vi "test exe main.vi"(6 "Offset":dbl=5.0, 7 "CustormMode":bool, 8 "error in":errorcluster, 10 "HWcurrent limt":sgl=0.5, 11 "Main State Cluster":T1={"Application Status"="", "Switch Output Array"=[], "Switch Value Configuration"=[], "NVH Configuration"={"NVH Station?"=FALSE, "nvh app instance path"="", "NVH_ErrorMessages sv url"="", "NVH_Inputs sv url"="", "NVH_MotionNumber sv url"="", "NVH_Outputs sv url"="", "NVH_PartNumber sv url"="", "NVH_PartNumber_Echo sv url"="", "NVH_SerialNumber sv url"="", "NVH_AmbientTempF sv url"=""}, "rs232 port map"={"PMAC"="COM3", "PS Port"="COM27", "LVDT Unit"="COM36", "RS232"="COM24"}, "ethernet address map"={"LVDT 1 Unit"="172.17.53.143", "LVDT Unit 1 port"=0}, "paths"={"Base Path"=path "", "system error log path"=path "", "Error Table Path"=path "C/Labview Code/System/Error Table", "Store errors log path"=path "C/Labview Code/System/Error Table", "data bytes log path"=path "C/Labview Code/System/Error Table", "network path"=path "C/Labview Code/System/Error Table"}, "Station Index"=0, "Store Data"={"Motion Data Array"=[], "Error Table"=[], "Sun Shade Close Force Limits"={"Overall Min"=0.0, "Overall Max"=0.0, "Avg Min"=0.0, "Avg Max"=0.0, "Truncation Start"=0.0, "Truncation End"=0.0, "Variance"=0.0, "Check Noise"=FALSE}, "Sun Shade Open Force Limits"={"Overall Min"=0.0, "Overall Max"=0.0, "Avg Min"=0.0, "Avg Max"=0.0, "Truncation Start"=0.0, "Truncation End"=0.0, "Variance"=0.0, "Check Noise"=FALSE}, "Sunshade Open Data"=[], "Sunshade Close Data"=[], "Module Info"={"Serial Number"="", "Pallet Number"="", "Sunshade Color"="", "Inalfa Part Number"="", "Customer Number"=""}, "Sunsahde Close Raw Data"=[], "Sunshade Open Raw Data"=[], "Software Version"=[], "Constant Version"=[], "Hardware Version"=[], "Inalfa Part Number ECU"=[], "LVDT Data"=[], "Communication Line 1"=[], "Communication Line 2"=[], "Anti Pinch Force"=[], "Cycle Time"="", "Anti Pinch Vent Force"=[], "iGPS LVDT Data"=[], "data bytes log"=""}, "D in map"={"Abort Test"=enum."Dev2/port2/line6", "Start Test"=enum."Dev2/port2/line6"}, "DO Task"="station 1 dio", "ctl refs"={"Start Test"=refnum, "Abort Test"=refnum, "Manual Control"=refnum, "Route to Repair"=refnum, "Waveform Graph"=refnum, "Motion Data"=refnum, "all station status"=refnum, "Individual Station Status"=refnum, "exit program"=refnum, "Sunshade Servo Data Open"=refnum, "Sunshade Servo Data Close"=refnum, "Red-Rabbit Mode"=refnum, "Direct Manual Ctrl"=refnum}, "misc station config"={"Station Name"="", "is AT station?"=FALSE, "is audit station?"=FALSE, "power supply type"=enum."GENser", "use alt China TP2 LVDT Logic Seq"=FALSE, "hmi operator abort timeout"=0, "dump all analog values even if pass"=FALSE, "debug log pre-filter ap stream bytes"=FALSE, "use separate lvdt x and z extend tags"=FALSE, "is print"=FALSE}, "ethernet tcp refs"={"LVDT Unit"=refnum}, "Sunshade Barcode Scan"={"Sunshade Number 2"="", "Sunshade Number 1"="", "Keyence tuning bank idx"=0}, "AP Test Data"={"Raw Sunshade AP Data"="", "Raw Glass AP Data"="", "PMAC Read Counter"=0.0, "Database AP Data"=[]}, "Motion Status"={"hmi operator abort start time"=0, "Current Data Index"=0, "Analog Data"=[], "Motor Position Hex"=0, "Messages Index"=0, "Last Bytes"=[], "Current Hall Position"=0, "Motion Stop Timer"=0, "Position Test"=enum."Not Tested", "Noise Test"=enum."Not Tested", "motion stop check initialized"=FALSE, "remote sense enabled"=FALSE, "Motion"=enum."Glass Teach"}, "LVDT Status"={"LVDT's stored config"=[], "lvdt precision"={"truncate instead of rounding"=FALSE, "decimal places"=0}}, "Sequence State"={"Step Description"="", "Cycle Start Time"=0, "Step Data String"="", "Pass?"=FALSE, "Seqence"=[], "Active Step"=0, "Testing?"=FALSE, "Red-Rabbit Mode"=FALSE, "route-to-repair mode"=FALSE, "NVH Status"={"Restart IRQ Counter"=0, "NVH Test Needed?"=FALSE, "NVH Test Running?"=FALSE}, "Present (s)"=0.0, "Hold Mode?"=FALSE, "Hold?"=FALSE, "Rx Invalid?"=FALSE}, "misc status"={"delay start time (ticks)"=0, "In Vehicle Mode?"=FALSE, "Diag Mode?"=FALSE, "Serial Port Configured?"=FALSE, "PS Voltage"=0.0, "Diag Serial Port"="", "Part Setup"={"Communication Type"=enum."None", "Send Messages to"=enum."Glass", "RAP Signal"=enum."High", "Motor Type"=enum."Smart Motor", "NVH Part Number"=0, "Turn Off Timer"=0, "Part Type"=""}, "Part History Number"="", "Plant Number"=0, "AP Data Type"=enum."91/61", "Real Rollo?"=FALSE}, "NVH Operator?"=FALSE, "NVH Pass?"=FALSE, "Operator Pass?"=FALSE, "Operator Action?"=FALSE, "Noise Source"=0, "USBHandle"=0, "PeakInfo"="", "PeakNumber"=0, "NVH Motion Steps"=[], "Second Check?"=FALSE, "Decibel data"=[], "Direct Control Info"={"EnableStopOnHome"=FALSE, "EnableStopOnPos"=FALSE, "TeachEvent"=FALSE, "open offset"=0, "close offset"=0, "Derect control"=FALSE, "set position"=[], "teach pass "=FALSE, "Drift offsets"=[], "Hall Positions"=[]}, "manual control(direct)"=FALSE, "LIN INFO"={"Toolkit Type"=enum."Inalfa LIN", "NAD"=36, "Inalfa LIN"={"Master Frame(3C)"="", "Slave Frame(3D)"="NIXNET_exampleLDF", "Request Schedule"="NIXNET_exampleLDF", "Response Schedule"="CEMLIN3DiagResponseSchedule\nSPA3414_ConfigurationsCMAGeely_CEMCALYPSOSDB34XX0Cfg_LIN3_190709_", "Frame Write SCU"="", "Frame Read SCU"="", "LIN Name"=""}, "ADCS LIN"={"Port"="MasterReq\nSPA3414_ConfigurationsCMAGeely_CEMCALYPSOSDB34XX0Cfg_LIN3_190709_", "HW select"=0, "XNET Cluster"="SlaveResp\nSPA3414_ConfigurationsCMAGeely_CEMCALYPSOSDB34XX0Cfg_LIN3_190709_", "ByteCmd Path"=path "C/Labview Code/System/ByteCmdConfig.txt"}, "TS LIN"={"ref info"=refnum, "LIN Channel"=0, "ByteCmd Path"=path "C/Labview Code/System/ByteCmdConfig.txt"}}, "Config Info"=variant} {"LIN INFO"."NAD" format="%.0x"; "LIN INFO"."ADCS LIN"."HW select" items=["NI-XNET", "NI-CAN"]; "LVDT Status"."LVDT's stored config"."Lower Limit" format="%.2f"; "LVDT Status"."LVDT's stored config"."Upper Limit" format="%.2f"; "Store Data"."Sun Shade Open Force Limits"."Variance" format="%.2g"; "Store Data"."Sun Shade Open Force Limits"."Truncation End" format="%.2g"; "Store Data"."Sun Shade Open Force Limits"."Truncation Start" format="%.2g"; "Store Data"."Sun Shade Open Force Limits"."Avg Max" format="%.2g"; "Store Data"."Sun Shade Open Force Limits"."Avg Min" format="%.2g"; "Store Data"."Sun Shade Open Force Limits"."Overall Max" format="%.2g"; "Store Data"."Sun Shade Open Force Limits"."Overall Min" format="%.2g"; "Store Data"."Sun Shade Close Force Limits"."Variance" format="%.2g"; "Store Data"."Sun Shade Close Force Limits"."Truncation End" format="%.2g"; "Store Data"."Sun Shade Close Force Limits"."Truncation Start" format="%.2g"; "Store Data"."Sun Shade Close Force Limits"."Avg Max" format="%.2g"; "Store Data"."Sun Shade Close Force Limits"."Avg Min" format="%.2g"; "Store Data"."Sun Shade Close Force Limits"."Overall Max" format="%.2g"; "Store Data"."Sun Shade Close Force Limits"."Overall Min" format="%.2g"; "Store Data"."Motion Data Array"."Motion Data Limits"."LIN Msg"."Msg" format="%02x"; "Store Data"."Motion Data Array"."Motion Data Limits"."LIN Msg"."ID" format="%02x"}) -> (0 "error out":errorcluster)   [LabVIEW 2018]
uses:
  02.Type Def's/main state cluster.ctl
  02.Type Def's/All Switch Configuration Cluster.ctl
  02.Type Def's/All Motions.ctl
  02.Type Def's/EOL Switch Value Configuration Cluster.ctl
  02.Type Def's/EOL Switch Max Min Check Cluster.ctl
  02.Type Def's/station nvh config.ctl
  02.Type Def's/station rs232 port map.ctl
  02.Type Def's/station ethernet address map.ctl
  02.Type Def's/station paths.ctl
  02.Type Def's/EOL Save Module Test Data Control.ctl
  02.Type Def's/EOL Motion Database Table.ctl
  05.UserVI's/type defs/17x Audit Motion Data Seq Control.ctl
  05.UserVI's/type defs/17x AP Data Type.ctl
  05.UserVI's/type defs/17x Sunshade Limts Seq.ctl
  02.Type Def's/EOL Module Info Control.ctl
  02.Type Def's/station DI map.ctl
  05.UserVI's/type defs/EOL Global Digital Input Control.ctl
  02.Type Def's/control refs.ctl
  02.Type Def's/station motion data indicator.ctl
  02.Type Def's/Screen Motion Data.ctl
  02.Type Def's/Pass Fail Control.ctl
  02.Type Def's/station hmi.ctl
  02.Type Def's/lvdt name val pair.ctl
  02.Type Def's/individual station status.ctl
  02.Type Def's/misc station config.ctl
  05.UserVI's/Lambda Power/power supply types.ctl
  05.UserVI's/type defs/EOL LVDT's Check Controller.ctl
  05.UserVI's/LVDT's/lvdt precision.ctl
  02.Type Def's/sequence state.ctl
  05.UserVI's/sequence/type defs/Sequence Info.ctl
  05.UserVI's/type defs/EOL Part Setup.ctl
  02.Type Def's/All Communication Types.ctl
  05.UserVI's/type defs/Communication with Motors.ctl
  05.UserVI's/type defs/RAP Signal Control.ctl
  05.UserVI's/type defs/EOL Motor Type.ctl
  02.Type Def's/station LIN config.ctl
  03.Inalfa LIN/LIN Device.ctl
  <vilib>/CMC.AME/Inalfa ADCS/Ctl'Def/ADCS_LIN info.ctl
  C:/Program Files (x86)/National Instruments/LabVIEW 2018/vi.lib/CMC.AME/Inalfa TS LIN/TOSUN/TSMaster/bin/Interop.TSMasterAPI.dll
  Program Files (x86)/National Instruments/LabVIEW 2018/vi.lib/CMC.AME/Inalfa TS LIN/TOSUN/TSMaster/bin/Interop.TSMasterAPI.dll
  Sub'VIs/Type Def's/Config Info.ctl
  02.Type Def's/NVH Mode Control 2.0.ctl
  02.Type Def's/NVH Digital Input.ctl
  02.Type Def's/EOL Analog Input Control.ctl
  02.Type Def's/failure behaviors.ctl
  05.UserVI's/type defs/RSLinx Boolean Cluster.ctl
  05.UserVI's/type defs/plc path and tag.ctl
  <vilib>/Platform/dataskt.llb/DataSocket Reference Type.ctl
  05.UserVI's/type defs/sequence goto step params.ctl
  05.UserVI's/type defs/EOL Global Digital Output Cluster Control.ctl
  05.UserVI's/type defs/EOL Global Digital Output Control.ctl
  05.UserVI's/BarCode/typedefs/barcode format params.ctl
  05.UserVI's/BarCode/typedefs/barcode printer types.ctl
  02.Type Def's/Sunshade Color Configuration Cluster.ctl
  05.UserVI's/type defs/Anti Pinch Test Data Control.ctl
  05.UserVI's/type defs/Goto Position Control.ctl
  02.Type Def's/NVH Digital Output.ctl
  <vilib>/Instr/_visa.llb/VISA Configure Serial Port (Instr).vi
  04.SubVI's/Fergus/ZUP_Current/Data buffer/ST0 current buffer.vi
  04.SubVI's/Fergus/ZUP_Current/Data buffer/ST1 current buffer.vi
  04.SubVI's/Fergus/ZUP_Current/Data buffer/ST2 current buffer.vi
  04.SubVI's/Fergus/ZUP_Current/Data buffer/ST3 current buffer.vi
  04.SubVI's/Fergus/ZUP_Current/Data buffer/ST4 current buffer.vi
  04.SubVI's/Fergus/ZUP_Current/Data buffer/ST5 current buffer.vi
  04.SubVI's/Others VI's/ftd2xx.dll
  <vilib>/Utility/config.llb/NI_LVConfig.lvlib
  <vilib>/Utility/config.llb/Read Key (String).vi
panel:
  in  "VI路径":path=path "C:/Labview Code/04.SubVI's/Direct Control Test/MotorDirectControl.vi"
  # "Sunroof Barcode"
  # "Pallet Number"
  # "Part Type"
  # "Application Status"
  # "Current Step"
  # "Cycle Time"
  # "Pass / Fail"
  # "Shade Close"
  # "Actual Data"
  # "Limits"
  # "Avg Current"
  # "Run Time"
  # "Speed"
  # "Noise Test"
  # "Position"
  # "Shade Open"
  # "Actual Data"
  # "Limits"
  # "Avg Current"
  # "Run Time"
  # "Speed"
  # "Noise Test"
  # "Position"
  # "Vent Close"
  # "Actual Data"
  # "Limits"
  # "Avg Current"
  # "Run Time"
  # "Speed"
  # "Noise Test"
  # "Position"
  # "Vent Open"
  # "Actual Data"
  # "Limits"
  # "Avg Current"
  # "Run Time"
  # "Speed"
  # "Noise Test"
  # "Position"
  # "Slide Close"
  # "Actual Data"
  # "Limits"
  # "Avg Current"
  # "Run Time"
  # "Speed"
  # "Noise Test"
  # "Position"
  # "Slide Open"
  # "Actual Data"
  # "Limits"
  # "Avg Current"
  # "Run Time"
  # "Speed"
  # "Noise Test"
  # "Position"
  # "Min"
  # "N"
  # "Min"
  # "Start"
  # "N"
  # "Max"
  # "N"
  # "Max"
  # "N"
  # "End"
  # "Min"
  # "N"
  # "Min"
  # "Start"
  # "N"
  # "Max"
  # "N"
  # "Max"
  # "N"
  # "End"
  # "Min"
  # "Max"
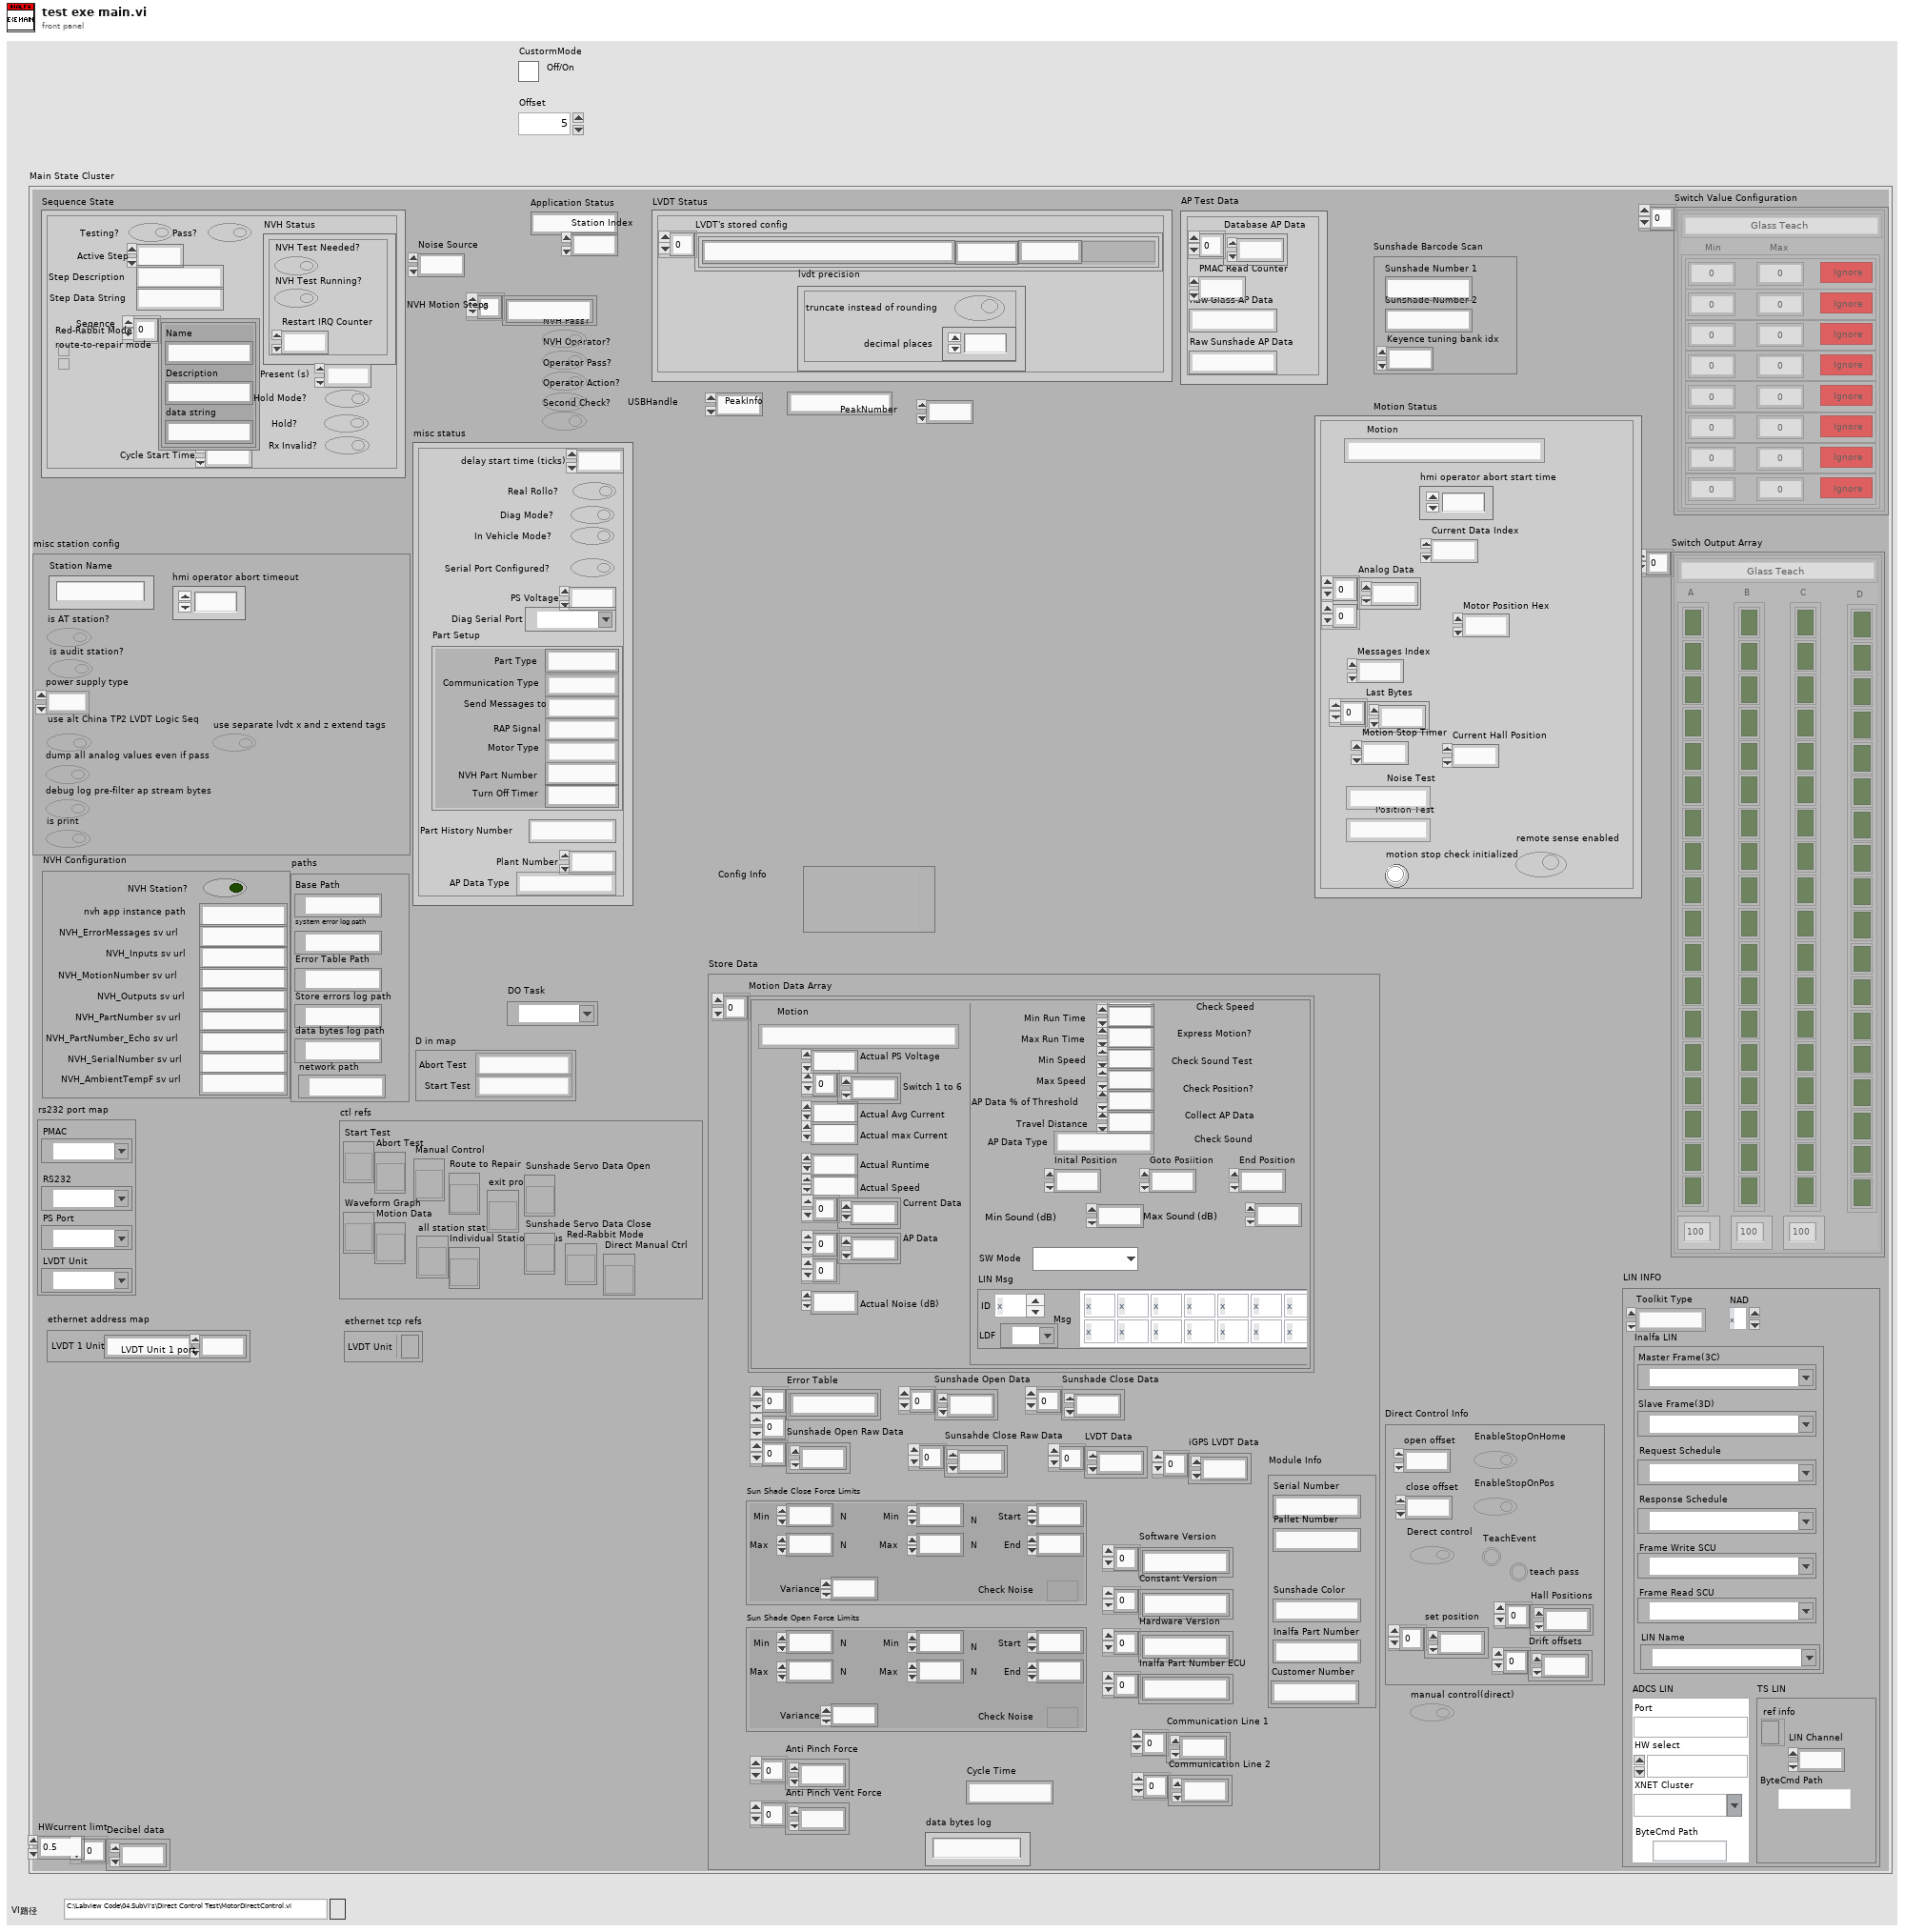
[diagram p1: front panel]
types:
  T1 = typedef "main state cluster.ctl" = cluster{"Application Status":string, "Switch Output Array":T2[], "Switch Value Configuration":T4[], "NVH Configuration":T6, "rs232 port map":T7, "ethernet address map":T8, "paths":T9, "Station Index":i32, "Store Data":T10, "D in map":T16, "DO Task":refnum<k21>, "ctl refs":T18, "misc station config":T19, "ethernet tcp refs":cluster{"LVDT Unit":refnum<k5>}, "Sunshade Barcode Scan":cluster{"Sunshade Number 2":string, "Sunshade Number 1":string, "Keyence tuning bank idx":i32}, "AP Test Data":cluster{"Raw Sunshade AP Data":string, "Raw Glass AP Data":string, "PMAC Read Counter":dbl, "Database AP Data":dbl[]}, "Motion Status":cluster{"hmi operator abort start time":u32, "Current Data Index":i32, "Analog Data":sgl[][], "Motor Position Hex":u16, "Messages Index":u16, "Last Bytes":u8[], "Current Hall Position":i16, "Motion Stop Timer":u32, "Position Test":T21, "Noise Test":T21, "motion stop check initialized":bool, "remote sense enabled":bool, "Motion":T3}, "LVDT Status":cluster{"LVDT's stored config":T22[], "lvdt precision":T23}, "Sequence State":T24, "misc status":cluster{"delay start time (ticks)":u32, "In Vehicle Mode?":bool, "Diag Mode?":bool, "Serial Port Configured?":bool, "PS Voltage":dbl, "Diag Serial Port":refnum<visa-resource-name>, "Part Setup":T26, "Part History Number":string, "Plant Number":u8, "AP Data Type":T13, "Real Rollo?":bool}, "NVH Operator?":bool, "NVH Pass?":bool, "Operator Pass?":bool, "Operator Action?":bool, "Noise Source":u32, "USBHandle":i32, "PeakInfo":string, "PeakNumber":i32, "NVH Motion Steps":string[], "Second Check?":bool, "Decibel data":dbl[], "Direct Control Info":cluster{"EnableStopOnHome":bool, "EnableStopOnPos":bool, "TeachEvent":bool, "open offset":i32, "close offset":i32, "Derect control":bool, "set position":i32[], "teach pass ":bool, "Drift offsets":i32[], "Hall Positions":i32[]}, "manual control(direct)":bool, "LIN INFO":T31, "Config Info":T34}
  T2 = typedef "All Switch Configuration Cluster.ctl" = cluster{"All Motions":T3, "A":bool[], "B":bool[], "C":bool[], "D":bool[], "A activation time (ms)":u32, "B activation time (ms)":u32, "C activation time (ms)":u32}
  T3 = typedef "All Motions.ctl" = enum16{"Glass Teach", "Glass Slide Open", "Glass Slide Close", "Glass Vent Open", "Glass Vent Close", "Sunshade Teach", "Sunshade Open", "Sunshade Close", "Idle", "Sunshade Open 2", "Sunshade Close 2", "Glass Slide Open Sunshade Open", "Glass Slide Open Sunshade Close", "Glass Slide Close Sunshade Open", "Glass Slide Close Sunshade Close", "Glass Vent Open Sunshade Open", "Glass Vent Open Sunshade Close", "Glass Vent Close Sunshade Open", "Glass Vent Close Sunshade Close", "Express Glass Slide Open", "Express Glass Slide Close", "Express Glass Vent Open", "Express Glass Vent Close", "Express Sunshade Open", "Express Sunshade Close", "Express Sunshade Open 2", "Express Sunshade Close 2", "Express Glass Slide Open Sunshade Open", "Express Glass Slide Open Sunshade Close", "Express Glass Slide Close Sunshade Open", "Express Glass Slide Close Sunshade Close", "Express Glass Vent Open Sunshade Open", "Express Glass Vent Open Sunshade Close", "Express Glass Vent Close Sunshade Open", "Express Glass Vent Close Sunshade Close", "Goto Position Glass", "Goto Position Sunshade", "Sunshade Teach 2"}
  T4 = typedef "EOL Switch Value Configuration Cluster.ctl" = cluster{"All Motions":T3, "Array":T5[]}
  T5 = typedef "EOL Switch Max Min Check Cluster.ctl" = cluster{"Min":dbl, "Max":dbl, "Check?":bool}
  T6 = typedef "station nvh config.ctl" = cluster{"NVH Station?":bool, "nvh app instance path":string, "NVH_ErrorMessages sv url":string, "NVH_Inputs sv url":string, "NVH_MotionNumber sv url":string, "NVH_Outputs sv url":string, "NVH_PartNumber sv url":string, "NVH_PartNumber_Echo sv url":string, "NVH_SerialNumber sv url":string, "NVH_AmbientTempF sv url":string}
  T7 = typedef "station rs232 port map.ctl" = cluster{"PMAC":refnum<visa-resource-name>, "PS Port":refnum<visa-resource-name>, "LVDT Unit":refnum<visa-resource-name>, "RS232":refnum<visa-resource-name>}
  T8 = typedef "station ethernet address map.ctl" = cluster{"LVDT 1 Unit":string, "LVDT Unit 1 port":u16}
  T9 = typedef "station paths.ctl" = cluster{"Base Path":path, "system error log path":path, "Error Table Path":path, "Store errors log path":path, "data bytes log path":path, "network path":path}
  T10 = typedef "EOL Save Module Test Data Control.ctl" = cluster{"Motion Data Array":T11[], "Error Table":string[][], "Sun Shade Close Force Limits":T14, "Sun Shade Open Force Limits":T14, "Sunshade Open Data":sgl[], "Sunshade Close Data":sgl[], "Module Info":T15, "Sunsahde Close Raw Data":sgl[], "Sunshade Open Raw Data":sgl[], "Software Version":string[], "Constant Version":string[], "Hardware Version":string[], "Inalfa Part Number ECU":string[], "LVDT Data":sgl[], "Communication Line 1":sgl[], "Communication Line 2":sgl[], "Anti Pinch Force":sgl[], "Cycle Time":string, "Anti Pinch Vent Force":sgl[], "iGPS LVDT Data":sgl[], "data bytes log":string}
  T11 = typedef "EOL Motion Database Table.ctl" = cluster{"Motion":T3, "Actual Avg Current":dbl, "Actual Runtime":dbl, "Actual Speed":dbl, "Current Data":sgl[], "Motion Data Limits":T12, "Switch 1 to 6":dbl[], "Actual PS Voltage":dbl, "AP Data":i16[][], "Actual max Current":dbl, "Actual Noise (dB)":dbl}
  T12 = typedef "17x Audit Motion Data Seq Control.ctl" = cluster{"Power Supply Voltage":dbl, "Min Avg Current":dbl, "Max Avg Current":dbl, "Min Run Time":dbl, "Max Run Time":dbl, "Min Speed":dbl, "Max Speed":dbl, "AP Data % of Threshold":dbl, "Travel Distance":dbl, "AP Data Type":T13, "Check Current":bool, "Check Run Time":bool, "Check Speed":bool, "Express Motion?":bool, "Check Sound Test":bool, "Check Position?":bool, "Collect AP Data":bool, "Inital Position":u16, "End Position":u16, "Goto Posiition":u16, "Max max Current":dbl, "Min max Current":dbl, "Check max Current":bool, "Check Sound":bool, "Min Sound (dB)":dbl, "Max Sound (dB)":dbl, "SW Mode":enum16{"Hard Switch", "Uncond Frame"}, "LIN Msg":cluster{"ID":u8, "Msg":u8[][], "LDF":refnum<k21>}}
  T13 = typedef "17x AP Data Type.ctl" = enum16{"91/61", "92/62", "93/63", "67", "68", "6F", "71", "91 Msg", "92 Msg", "93 Msg", "94 Msg", "HiRain 91", "HiRain 92 Speed", "HiRain 92 HS", "HiRain 92", "HiRain 93", "SnT"}
  T14 = typedef "17x Sunshade Limts Seq.ctl" = cluster{"Overall Min":dbl, "Overall Max":dbl, "Avg Min":dbl, "Avg Max":dbl, "Truncation Start":dbl, "Truncation End":dbl, "Variance":dbl, "Check Noise":bool}
  T15 = typedef "EOL Module Info Control.ctl" = cluster{"Serial Number":string, "Pallet Number":string, "Sunshade Color":string, "Inalfa Part Number":string, "Customer Number":string}
  T16 = typedef "station DI map.ctl" = cluster{"Abort Test":T17, "Start Test":T17}
  T17 = typedef "EOL Global Digital Input Control.ctl" = enum16{"Dev2/port0/line0", "Dev2/port0/line1", "Dev2/port0/line2", "Dev2/port0/line3", "Dev2/port0/line4", "Dev2/port0/line5", "Dev2/port0/line6", "Dev2/port0/line7", "Dev2/port1/line0", "Dev2/port1/line1", "Dev2/port1/line2", "Dev2/port1/line3", "Dev2/port1/line4", "Dev2/port1/line5", "Dev2/port1/line6", "Dev2/port1/line7", "Dev2/port2/line0", "Dev2/port2/line1", "Dev2/port2/line2", "Dev2/port2/line3", "Dev2/port2/line4", "Dev2/port2/line5", "Dev2/port2/line6", "Dev2/port2/line7", "Prerun Start Test", "Prerun Abort Test", "Audit Start Test", "Audit Abort Test", "Dev2/port3/line4", "Dev2/port3/line5", "Breakin Start Test", "Breakin Abort Test", "Not Implemented"}
  T18 = typedef "control refs.ctl" = cluster{"Start Test":refnum<vi>, "Abort Test":refnum<vi>, "Manual Control":refnum<vi>, "Route to Repair":refnum<vi>, "Waveform Graph":refnum<vi>, "Motion Data":refnum<vi>, "all station status":refnum<vi>, "Individual Station Status":refnum<vi>, "exit program":refnum<vi>, "Sunshade Servo Data Open":refnum<vi>, "Sunshade Servo Data Close":refnum<vi>, "Red-Rabbit Mode":refnum<vi>, "Direct Manual Ctrl":refnum<vi>}
  T19 = typedef "misc station config.ctl" = cluster{"Station Name":string, "is AT station?":bool, "is audit station?":bool, "power supply type":T20, "use alt China TP2 LVDT Logic Seq":bool, "hmi operator abort timeout":u32, "dump all analog values even if pass":bool, "debug log pre-filter ap stream bytes":bool, "use separate lvdt x and z extend tags":bool, "is print":bool}
  T20 = typedef "power supply types.ctl" = enum16{"GENser", "ZUPser", "GENeth", "Manual", "ITECH"}
  T21 = typedef "Pass Fail Control.ctl" = enum16{"Not Tested", "Pass", "Fail"}
  T22 = typedef "EOL LVDT's Check Controller.ctl" = cluster{"Upper Limit":dbl, "Lower Limit":dbl, "LVDT Name":string, "Check":bool}
  T23 = typedef "lvdt precision.ctl" = cluster{"truncate instead of rounding":bool, "decimal places":u8}
  T24 = typedef "sequence state.ctl" = cluster{"Step Description":string, "Cycle Start Time":u32, "Step Data String":string, "Pass?":bool, "Seqence":T25[], "Active Step":u8, "Testing?":bool, "Red-Rabbit Mode":bool, "route-to-repair mode":bool, "NVH Status":cluster{"Restart IRQ Counter":u8, "NVH Test Needed?":bool, "NVH Test Running?":bool}, "Present (s)":dbl, "Hold Mode?":bool, "Hold?":bool, "Rx Invalid?":bool}
  T25 = typedef "Sequence Info.ctl" = cluster{"Name":string, "Description":string, "data string":string}
  T26 = typedef "EOL Part Setup.ctl" = cluster{"Communication Type":T27, "Send Messages to":T28, "RAP Signal":T29, "Motor Type":T30, "NVH Part Number":u16, "Turn Off Timer":u16, "Part Type":string}
  T27 = typedef "All Communication Types.ctl" = enum16{"None", "CAN", "RS 232", "RS 232 LIN", "GM LIN", "SnT LIN", "K Line", "Robel CAN", "P42M-Continental", "Inalfa SCU LIN", "Spare 3"}
  T28 = typedef "Communication with Motors.ctl" = enum16{"Glass", "Rollo", "Both"}
  T29 = typedef "RAP Signal Control.ctl" = enum16{"High", "Low", "None"}
  T30 = typedef "EOL Motor Type.ctl" = enum16{"Smart Motor", "Sensor Motor"}
  T31 = typedef "station LIN config.ctl" = cluster{"Toolkit Type":enum16{"Inalfa LIN", "ADCS LIN", "TS LIN"}, "NAD":u8, "Inalfa LIN":T32, "ADCS LIN":T33, "TS LIN":cluster{"ref info":refnum<k24>, "LIN Channel":i32, "ByteCmd Path":path}}
  T32 = typedef "LIN Device.ctl" = cluster{"Master Frame(3C)":refnum<k21>, "Slave Frame(3D)":refnum<k21>, "Request Schedule":refnum<k21>, "Response Schedule":refnum<k21>, "Frame Write SCU":refnum<k21>, "Frame Read SCU":refnum<k21>, "LIN Name":refnum<k21>}
  T33 = typedef "ADCS_LIN info.ctl" = cluster{"Port":string, "HW select":u16, "XNET Cluster":string, "ByteCmd Path":path}
  T34 = typedef "Config Info.ctl" = variant
  T35 = typedef "lvdt name val pair.ctl" = cluster{"lvdt name":string, "value":dbl}
  T36 = typedef "NVH Mode Control 2.0.ctl" = enum16{"Init", "Write", "Write String", "Read", "Write Part Number", "Write Motion Number", "Write Ambient TempF"}
  T37 = typedef "EOL Analog Input Control.ctl" = enum16{"SW PS  Volage", "Switch A", "Switch B", "Switch C", "Motor Voltage", "Motor Current", "ATS"}
  T38 = typedef "failure behaviors.ctl" = enum16{"stop immediately", "stop immediately if not rabbit", "stop at next 'check sequence' if not rabbit"}
  T39 = typedef "sequence goto step params.ctl" = cluster{"Data Boolean":bool, "PLC Path and Tag":T40, "goto step":u8}
  T40 = typedef "plc path and tag.ctl" = cluster{"Tag Name":string, "Network Path":string, "use opc":bool, "DataSocket Reference":T41}
  T41 = typedef "DataSocket Reference Type.ctl" = cluster{"CWDSLib._DCWDataSocket":refnum<k7>, "CWDSLib._DCWData":refnum<k7>, "OnDataUpdated":u32, "OnStatusUpdated":u32}
  T42 = typedef "RSLinx Boolean Cluster.ctl" = cluster{"Data Boolean":bool, "PLC Path and Tag":T40, "Error No.":u16, "timeout (ms)":i32, "Continue on Fail for Red-Rabbit":bool}
  T43 = typedef "EOL Global Digital Output Control.ctl" = enum16{"Battery", "IGN High", "IGN Low", "LIN", "CAN", "Switch 1", "Switch 2", "Switch 3", "Switch 4", "Switch 5", "Switch 6", "Glass Analog Switch 1", "Glass Analog Switch 2", "Glass Analog Switch 3", "Glass Analog Switch 4", "Sunshade Analog Switch 1", "Sunshade Analog Switch 2", "Sunshade Analog Switch 3", "Sunshade Analog Switch 4", "Glass Motor Relay 1", "Glass Motor Relay 2", "Sunshade Motor Relay 1", "Sunshade Motor Relay 2"}
  T44 = typedef "EOL Global Digital Output Cluster Control.ctl" = cluster{"Status":bool, "Global DO Ch":T43}
  T45 = enum16{"Init", "Write", "Write All", "Clear All", "Stop"}
  T46 = typedef "Sunshade Color Configuration Cluster.ctl" = cluster{"Sunshade 1 Number":string, "Sunshade 2 Number":string, "keyence tuning bank param idx":i32}
  T47 = enum16{"SW PS Voltage", "SW IGN Bat", "Switch A", "Switch B", "Motor Voltage", "Motor Current"}
  T48 = typedef "Anti Pinch Test Data Control.ctl" = cluster{"Power Supply Voltage":dbl, "Glass  Max Reversal Force":dbl, "Rollo Max Reversal Force":dbl, "Rollo02 Max Reversal Force":dbl, "Vent Max Reversal Force":dbl}
  T49 = cluster{"Baud Rate":i32, "DataBits":u8, "StopBits":u8, "Parity":u8}
  T50 = typedef "Goto Position Control.ctl" = cluster{"AP Data Type":T13, "Glass Motor?":bool, "Collect AP Data?":bool, "Go To Position":u16, "Rear Rollo?":bool}
  T51 = typedef "individual station status.ctl" = cluster{"Line Number":u8, "Serial Port":bool, "Loop Stopped?":bool, "Nidec Serial #":string, "Platform Constant":string, "ATS Constant":string, "Position Constant":string, "Schematic Ver":string, "Bootloader Ver":string, "Hardware Ver":string, "Vehicle Type":string, "Inalfa Motor P/N":string, "System Mode":string, "DTC's?":bool, "Calibrated?":bool, "Slide Count":u16, "Vent Count":u16, "Glass Voltage":dbl, "Anti Pinch Test?":bool, "Station":string}
  T52 = typedef "station hmi.ctl" = cluster{"Error Table Br":string[][], "Pass / Fail":u32, "Cycle Time Br":dbl, "Sunroof Barcode":string, "Pallet Number":string, "Part Type":string, "Current Step Br":string, "Application Status":string, "Station Name":string, "Database LVDT's Data Out":T35[], "NVH System":bool, "Date":string, "Time":string}
  T53 = cluster{"Noise Test":T21, "Avg Current":dbl, "Run Time":dbl, "Speed":dbl, "Position":T21}
  T54 = typedef "station motion data indicator.ctl" = cluster{"Shade Close Limits":T55, "Shade Close Data 2":T55, "Shade Open Limits":T55, "Shade Open Data":T55, "Vent Close Limits":T55, "Vent Close Data":T55, "Vent Open Limits":T55, "Vent Open Data":T55, "Slide Close Limits":T55, "Slide Close Data":T55, "Slide Open Limits":T55, "Slide Open Data":T55}
  T55 = typedef "Screen Motion Data.ctl" = cluster{"Noise Test":T21, "Avg Current":dbl, "Run Time":dbl, "Speed":dbl, "Position":T21}
  T56 = typedef "plc comms params.ctl" = cluster{"PLC boolean read Tags":T57, "PLC bool write Tags":T58, "PLC string read Tags":T59, "PLC string write Tags":T60, "use opc":bool, "PLC/OPC Path":string}
  T57 = typedef "station plc read boolean tags.ctl" = cluster{"AT glass position":T40, "AT shade position":T40, "AT in glass wand lower pos":T40, "AT in glass wand up pos":T40, "AT in sunshad wand lower pos":T40, "AT in sunshad wand up pos":T40, "AT in wand home pos":T40, "LVDT's Extended":T40, "bolt check 1":T40, "bolt check 2":T40, "bolt check 3":T40, "bolt check 4":T40, "bolt check 5":T40, "bolt check 6":T40, "bolt check 7":T40, "bolt check 8":T40, "start":T40, "abort":T40, "LVDT's Retracted":T40, "manual barcode print":T40, "ss servo at open":T40, "ss servo at close":T40, "ss servo opening":T40, "ss servo closing":T40, "control slide at home":T40, "control slide left good":T40, "control slide left over stroke":T40, "control slide right good":T40, "control slide right over stroke":T40, "wind deflector high speed pos":T40, "wind deflector low speed pos":T40, "AT VentPMACatHome":T40, "AT VentPMACisExtend":T40, "SS Barcode Scanner Bypassed":T40, "Check Frame Barcode":T40, "Z LVDTs Extended":T40, "NVH Operator Pass":T40, "NVH Operator Fail":T40, "NVH Operator Express Glass Open":T40, "NVH Operator Express Glass Close":T40, "NVH Operator Express Rollo Open01":T40, "NVH Operator Express Rollo Close01":T40, "NVH Operator Express Rollo Open02":T40, "NVH Operator Express Rollo Close02":T40, "NVH Operator Vent Open Noise":T40, "NVH Operator Vent Close Noise":T40, "NVH Operator Sunshade Open Noise":T40, "NVH Operator Sunshade Close Noise":T40, "NVH Operator Glass Open Noise":T40, "NVH Operator Glass Close Noise":T40, "NVH Operator Finish":T40, "NVH Operator Check":T40, "windproof position":T40, "NVH Operator Express Glass vent Open":T40, "NVH Operator Express Glass Vent Close":T40, "NVH Operator Re-do":T40, "AT at vent ATS test pos":T40, "AT at vent ATS Home pos":T40, "Start Adjust LVDT":T40, "Finish Adjust LVDT":T40}
  T58 = typedef "station plc write boolean tags.ctl" = cluster{"AT set glass wand lower":T40, "AT set sunshade wand lower":T40, "AT set sunshade wand up":T40, "AT set glass wand up":T40, "AT set wand home pos":T40, "Test Complete Pass":T40, "Test Complete Fail":T40, "Test Started":T40, "Retract LVDT's":T40, "Extend LVDT's":T40, "ss servo open":T40, "ss servo close":T40, "control slide start":T40, "control slide stop":T40, "AT VentPMACHome":T40, "AT VentPMACExtended":T40, "Good Frame Barcode":T40, "Bad Frame Barcode":T40, "Extend Z LVDTS":T40, "NVH SunRoof Moving":T40, "NVH SunRoof Stop":T40, "NVH Pass":T40, "NVH Fail":T40, "NVH Operator Express Glass Opened":T40, "NVH Operator Express Glass Closed":T40, "NVH Operator Express Rollo Opened01":T40, "NVH Operator Express Rollo Closed01":T40, "NVH Operator Express Rollo Opened02":T40, "NVH Operator Pass":T40, "NVH Operator Fail":T40, "NVH Operator Check":T40, "NVH Operator Vent Open Noise":T40, "NVH Operator Vent Close Noise":T40, "NVH Operator Sunshade Open Noise":T40, "NVH Operator Sunshade Close Noise":T40, "NVH Operator Glass Open Noise":T40, "NVH Operator Glass Close Noise":T40, "NVH Operator Finish":T40, "Barcode01 OK":T40, "Barcode02 OK":T40, "AT set to Vent ATS Test Pos":T40, "AT set to Vent ATS Home Pos":T40, "Move LVDT Adjust Station":T40}
  T59 = typedef "station plc read string tags.ctl" = cluster{"Serial Number":T40, "Pallet Number":T40, "Inalfa Part Number":T40, "Shade Color":T40, "Model Type":T40, "Customer Number":T40, "Part History Number":T40, "Shade 1 Barcode":T40, "Shade 2 Barcode":T40, "Manual Serial Number":T40, "Manual Inalfa Part Number":T40, "Manual Shade Color":T40, "Manual Model Type":T40, "Manual Customer Number":T40, "Manual Part History Number":T40}
  T60 = typedef "station plc write string tags.ctl" = cluster{"barcode station error":T40, "error message 0":T40, "error message 1":T40, "error message 2":T40, "error message 3":T40}
  T61 = typedef "NVH Digital Input.ctl" = enum16{"Online", "Pass", "Fail", "Testing", "Ready for Model", "Error Bit 1", "Error Bit 2", "Error Bit 3", "Failure Bit 1", "Failure Bit 2", "Failure Bit 3", "Failure Bit 4", "Echo Bit 1", "Echo Bit 2", "Echo Bit 3", "Echo Bit 4", "Serial Number Read Ok", "Ready for Serrial Number"}
  T62 = typedef "barcode format params.ctl" = cluster{"Format String":string, "Print String":string, "Quantity":u8, "printer type":T63, "RS232 Port":string, "IP Address":string, "Ethernet Port":u32}
  T63 = typedef "barcode printer types.ctl" = enum16{"Intermec RS232", "Intermec Ethernet"}
  T64 = cluster{"Serial Number":string, "Pallet Number":string, "Inalfa Part Number":string, "Part Type":string, "Shade Color":string, "Customer Number":string, "Part History Number":string, "Sunshade Barcode 2":string, "Sunshade Barcode 1":string}
  T65 = cluster{"ref info":refnum<k24>, "LIN Channel":i32, "ByteCmd Path":path}
  T66 = enum16{"NO read", "Softeware version", "Hardware version", "Calfile version"}
  T67 = cluster{"Step Description":string, "Cycle Start Time":u32, "Step Data String":string, "Pass?":bool, "Seqence":cluster{"Name":string, "Description":string, "data string":string}[], "Active Step":u8, "Testing?":bool, "Red-Rabbit Mode":bool, "route-to-repair mode":bool, "NVH Status":cluster{"Restart IRQ Counter":u8, "NVH Test Needed?":bool, "NVH Test Running?":bool}, "Present (s)":dbl, "Hold Mode?":bool, "Hold?":bool, "Rx Invalid?":bool}
  T68 = typedef "NI_LVConfig.lvlib/Config Data RefNum.ctl" = refnum<k1>
  T69 = typedef "NVH Digital Output.ctl" = enum16{"Restart IRQ", "Abort Test IRQ", "Read Model", "Start Test", "Stop Test", "End of Test IRQ", "Test Bit 1", "Test Bit 2", "Test Bit 3", "Test Bit 4", "Model Bit 1", "Model Bit 2", "Model Bit 3", "Model Bit 4", "Manual Restart IRQ"}
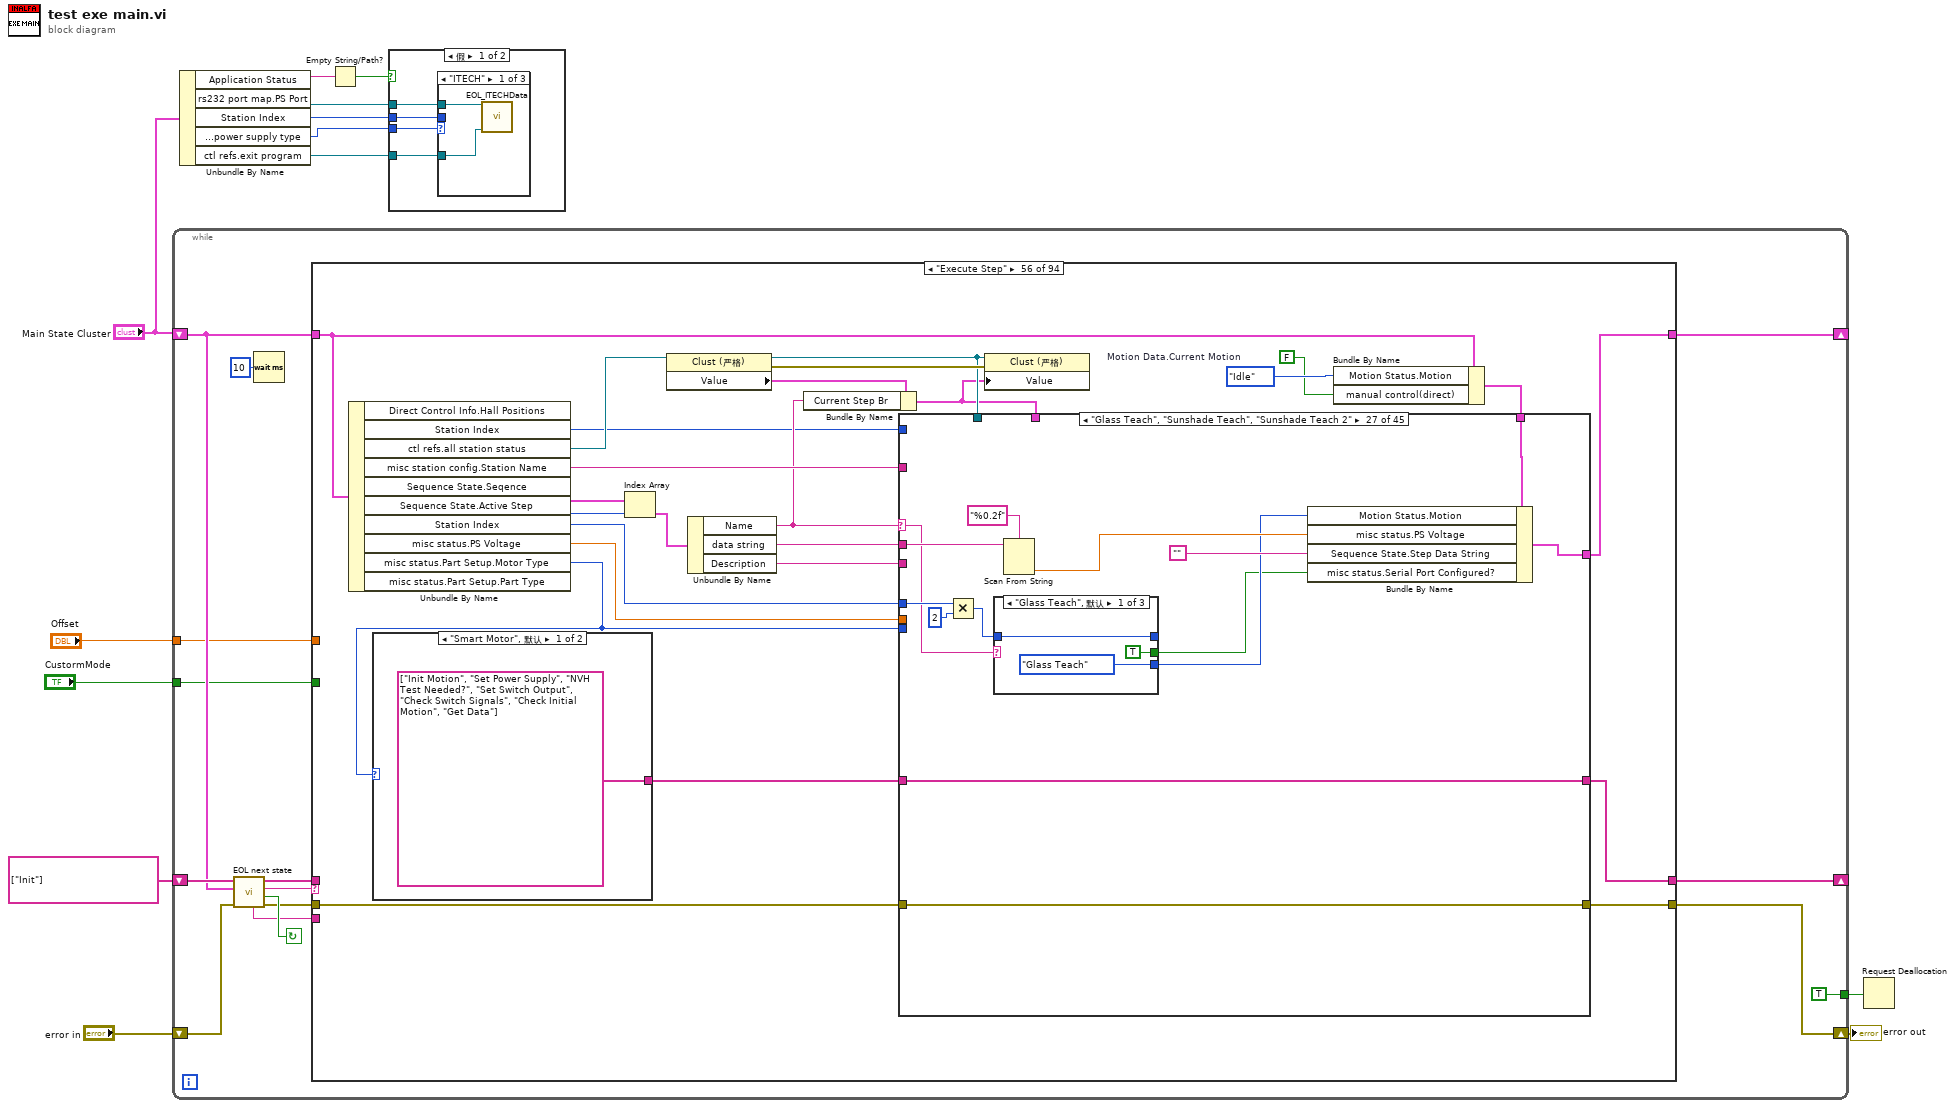
[diagram p0: block diagram]
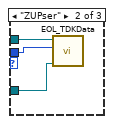
[diagram p2: hidden frame]
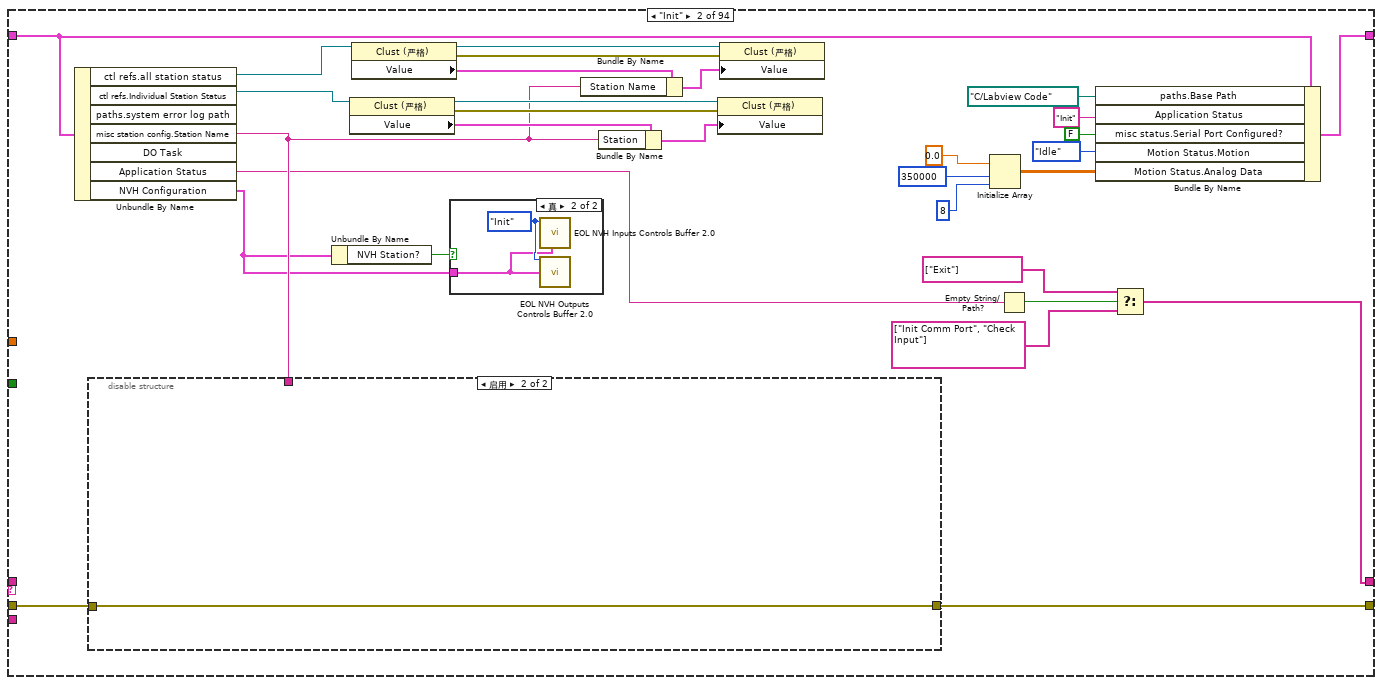
[diagram p6: hidden frame]
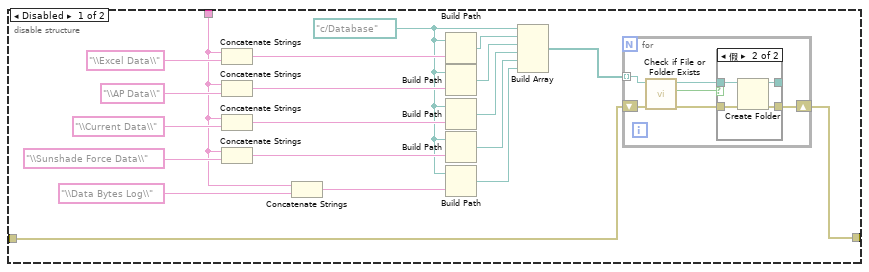
[diagram p7: hidden frame]
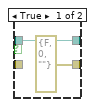
[diagram p8: hidden frame]
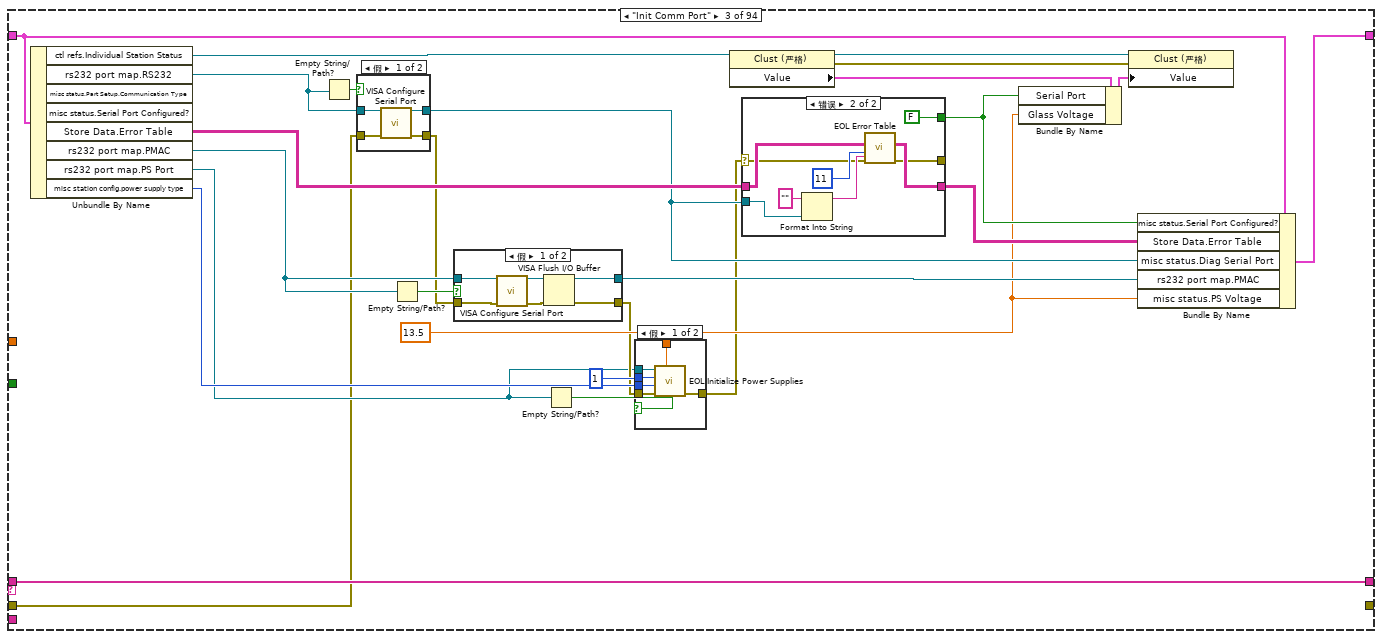
[diagram p10: hidden frame]
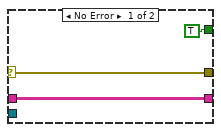
[diagram p14: hidden frame]
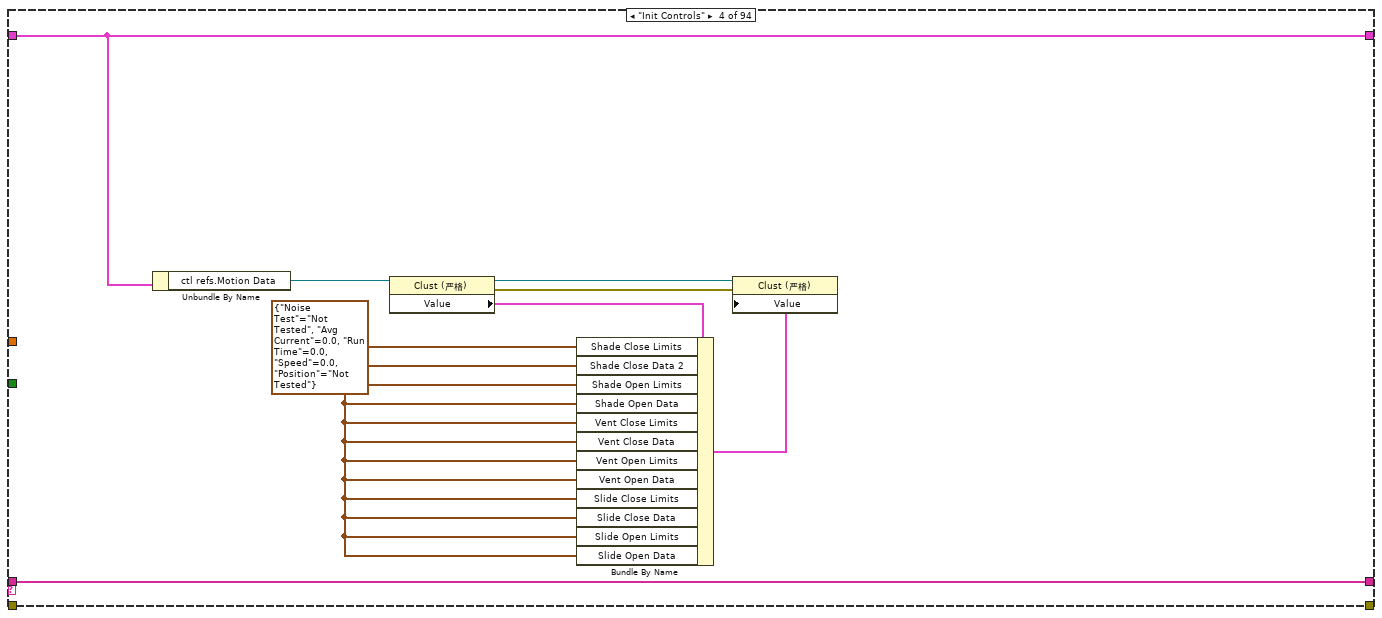
[diagram p15: hidden frame]
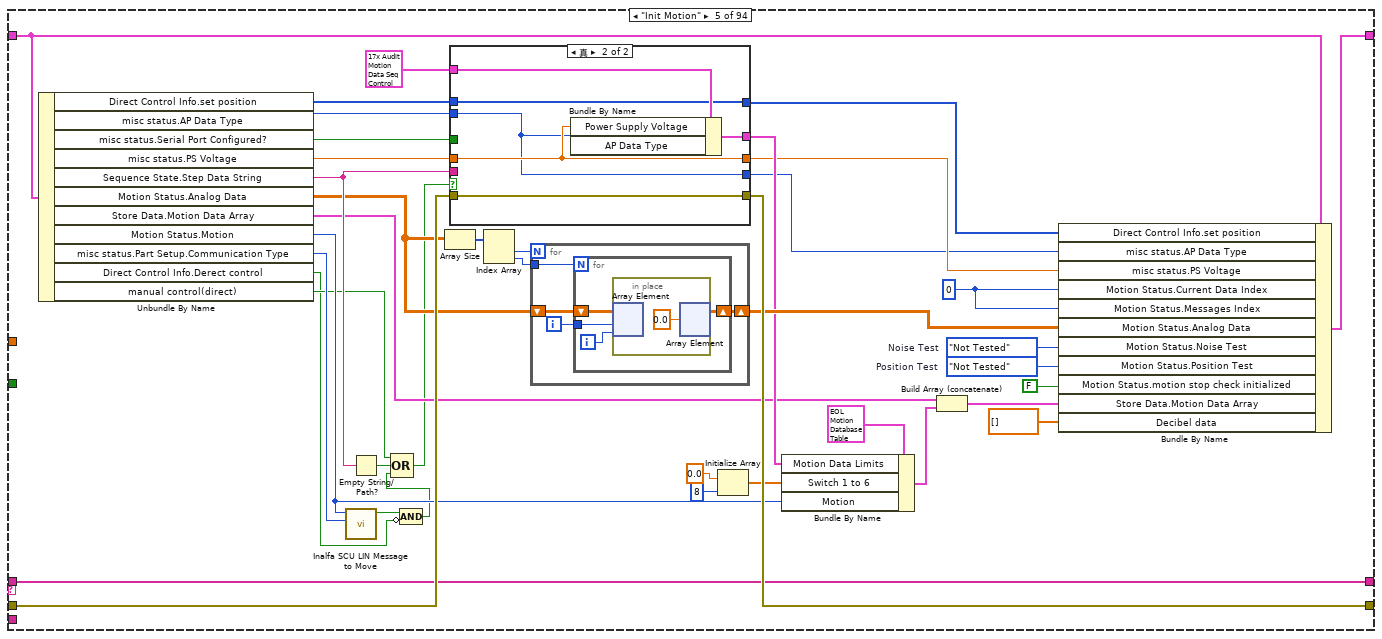
[diagram p16: hidden frame]
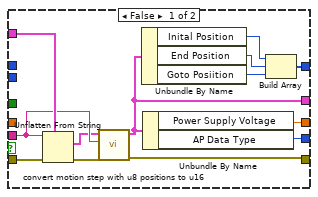
[diagram p17: hidden frame]
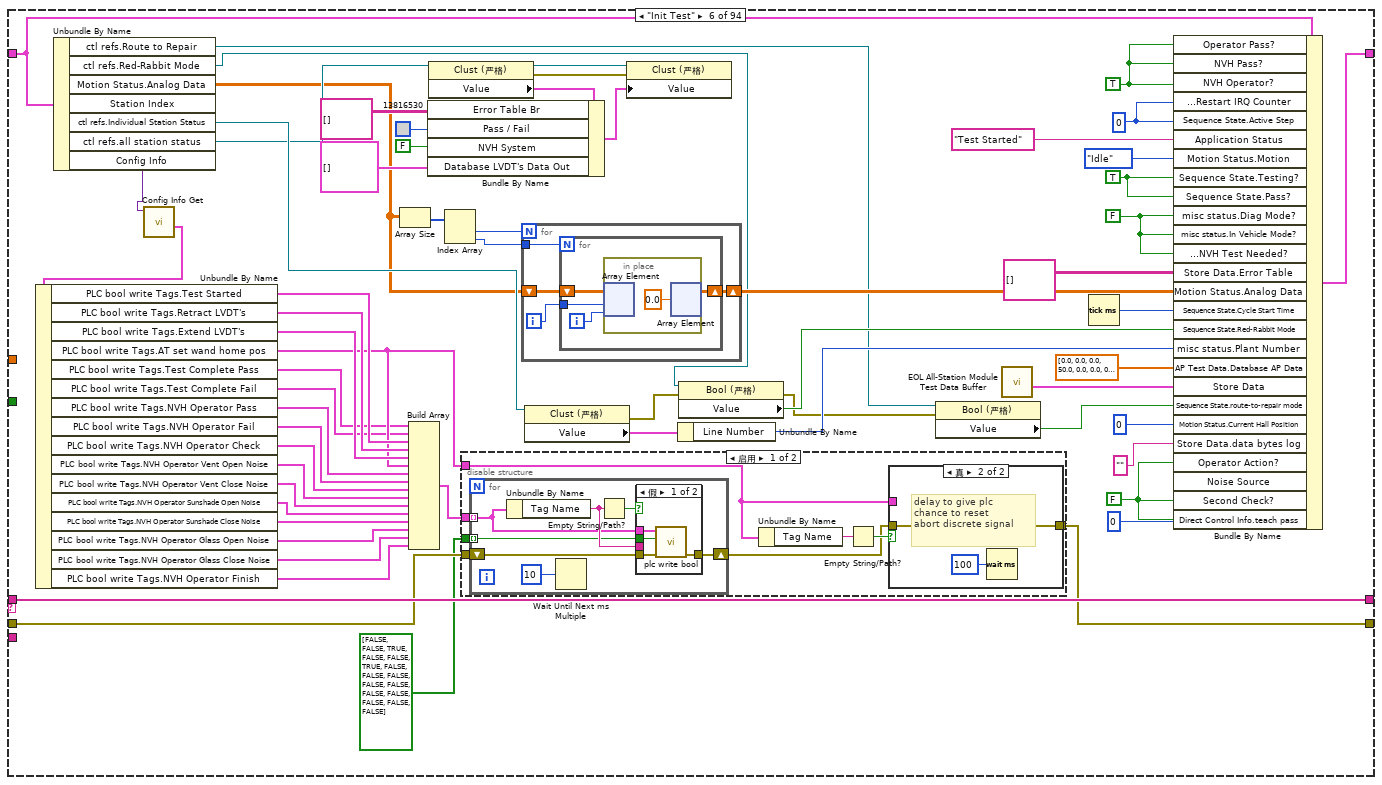
[diagram p18: hidden frame]
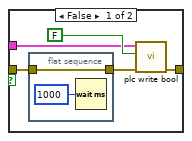
[diagram p19: hidden frame]
diagram:
  n1 = while {
    shift-right: [w28] -> _
    shift-left: string[] ["Init"] ("event queue out") -> [w25]
    shift-right: [w27] -> _
    shift-left: "Main State Cluster" -> [w20]
    shift-right: [w19] -> w13
    shift-left: "error in" -> [w23]
    tunnel: "Offset" -> [w16]
    tunnel: "CustormMode" -> [w15]
    tunnel: [TRUE ("标志")] -> w1
    stop <- w22 continue-if-true
    n2 = call "EOL next state.vi"("error in"=w23, "Main State Cluster"=w20, "event queue in"=w25) -> ("error out"=w17:errorcluster, "Condition (Exit:F)"=w22:bool, "next event"=w18:string, "event queue out"=w24:string[], "Previous Event"=w21:string)  [unwired: 4 in]
    n3 = Wait (ms)(milliseconds to wait=u32 10) -> ()  [unwired: 1 out]
    n4 = case shown="\"Execute Step\"" w18 {
      selector: w18 -> [_ _ _ _ _ _ _ _ _ _ _ _ _ _ _ _ _ _ _ _ _ _ _ _ _ _ _ _ _ _ _ _ _ _ _ _ _ _ _ w1332 _ _ w1426 w1483 _ w1567 _ _ _ _ _ _ _ _ _ _ _ _ _ _ _ _ _ _ _ _ _ _ _ _ _ _ _ _ _ _ _ _ _ _ _ _ _ w3187 _ w3224 _ _ _ _ _ _ _ w3775]
      tunnel: w24 -> [w30 _ w120 w163 w184 w285 w338 w361 _ _ _ w458 w471 w509 w533 _ w610 w624 w642 w660 w684 w717 _ w747 w757 w779 _ w846 _ w935 w989 w1018 w1059 w1175 w1196 _ w1226 w1245 w1290 w1324 w1380 w1411 w1431 w1473 w1507 w1570 w1639 w1658 w1677 w1689 w1707 w1717 w1729 w1747 _ _ w2236 _ w2330 w2339 _ _ w2490 w2498 w2536 w2576 w2600 w2632 w2671 w2717 w2753 w2826 w2897 _ _ w2988 w2995 w3035 w3057 w3077 w3111 w3117 w3146 w3188 w3213 w3219 w3258 w3289 w3297 w3329 w3356 w3385 _ w3769]
      tunnel: [w30 w34 w120 w163 w184 w285 w337 w361 string[] ["Init Controls", "Init Test", "Read Barcode", "Get Sequences", "Initialize NVH Test", "Turn RAP On", "Turn Power On", "Check Motor Connection", "Execute Step"] w367 w411 w457 w470 w508 w529 w569 w609 w622 w639 w656 w682 w716 w733 w747 w757 w778 w813 w846 w883 w935 w989 w1015 w1058 w1174 w1196 string[] ["Exit"] ("event queue out") w1226 w1246 w1291 w1323 w1381 w1411 w1431 w1472 w1506 w1569 w1639 w1658 w1677 w1688 w1707 w1717 w1728 w1747 w1757 w1782 w2234 w2295 w2330 w2339 w2371 w2457 w2490 w2497 w2535 w2575 w2600 w2631 w2670 w2718 w2752 w2825 w2896 w2948 string[] ["check NVH Operator result"] ("Event queue out") w2988 w2993 w3035 w3055 w3076 w3111 w3117 w3146 w3188 w3213 w3218 w3258 w3289 w3297 w3329 w3357 w3385 w3420 w3774] -> w28
      tunnel: w20 -> [w31 w41 w122 w158 w192 w239 w335 w362 w363 w375 w408 w466 w482 w499 w535 w554 w615 w629 w651 w663 w687 w720 w736 w746 w756 w786 w817 w845 w910 w932 w988 w1027 w1038 w1169 w1188 w1214 w1227 w1261 w1306 w1329 w1395 w1410 w1433 w1485 w1513 w1561 w1641 w1660 w1679 w1684 w1704 w1714 w1725 w1748 w1756 w1775 w2227 w2297 w2331 w2334 w2360 w2448 w2491 w2499 w2548 w2578 w2602 w2643 w2672 w2716 w2756 w2830 w2899 w2939 w2975 w2989 w3005 w3033 w3060 w3080 w3094 w3116 w3145 w3186 w3214 w3231 w3249 w3280 w3294 w3302 w3366 w3377 w3398 w3772]
      tunnel: [w31 w60 w121 w158 w202 w287 w336 w362 w363 w376 w412 w465 w481 w510 w523 w568 w616 w630 w652 w670 w694 w719 w737 w744 w756 w786 w816 w845 w909 w932 w990 w1028 w1039 w1170 w1188 w1214 w1227 w1260 w1305 w1336 w1394 w1410 w1432 w1484 w1512 w1588 w1640 w1659 w1678 w1693 w1704 w1714 w1736 w1748 w1755 w1783 w2253 w2308 w2331 w2338 w2372 w2458 w2491 w2496 w2547 w2577 w2601 w2629 w2669 w2715 w2757 w2829 w2898 w2946 w2975 w2989 w3004 w3033 w3067 w3087 w3109 w3116 w3145 w3186 w3214 w3225 w3249 w3279 w3294 w3302 w3365 w3377 w3421 w3771] -> w27
      tunnel: [w29 w38 _ _ w193 w277 _ w360 _ w371 w383 w462 w473 w494 w524 _ _ _ _ w661 w685 w703 w734 w741 _ _ _ _ w882 w916 w957 _ _ w1161 w1186 _ w1225 w1253 w1298 w1321 w1388 w1408 w1427 w1475 w1509 w1584 w1638 w1657 w1676 w1691 _ _ w1731 w1746 _ w1771 w2225 w2296 w2329 _ w2374 w2460 w2489 _ _ _ _ _ _ _ _ _ _ w2949 w2972 w2987 w2996 w3045 w3058 w3078 w3107 w3113 w3141 w3182 w3212 _ _ w3268 w3290 w3319 w3362 w3384 w3410 w3763] -> w19
      tunnel: w17 -> [w29 w37 w97 _ w194 w283 _ w360 _ w372 w385 w462 w474 w495 w524 _ _ _ _ w662 w686 w703 w734 w742 _ _ _ _ w882 w917 w987 _ _ w1165 w1187 _ w1225 w1254 w1299 w1335 w1389 w1409 w1430 w1476 w1510 w1575 w1638 w1657 w1676 w1692 _ _ w1735 w1746 _ w1772 w2244 w2281 w2329 _ w2374 w2460 w2489 _ _ _ _ _ _ _ _ _ _ w2949 _ w2987 w2997 w3046 w3059 w3079 w3095 w3112 w3142 w3183 w3212 _ _ w3269 w3291 w3311 w3354 w3384 w3411 w3764]
      tunnel: w21 -> [_ _ _ _ _ _ _ _ _ _ _ _ _ _ _ _ _ _ _ _ _ _ _ _ _ _ _ _ _ _ _ _ _ _ _ _ _ _ _ _ _ _ _ _ _ _ _ _ _ _ _ _ _ _ _ _ _ _ _ _ _ _ _ _ _ _ _ _ _ _ _ _ _ _ _ _ _ _ _ _ _ _ _ _ _ _ _ _ _ _ w3369 _ _ _]
      tunnel: w16 -> [_ _ _ _ _ _ _ _ _ _ _ _ _ _ _ _ _ _ _ _ _ _ _ _ _ _ _ _ _ _ _ _ _ _ _ _ _ _ _ _ _ _ _ _ _ _ w1629 w1647 w1666 _ _ _ _ _ _ _ _ _ _ _ _ _ _ _ _ _ _ _ _ _ _ _ _ _ _ _ _ _ _ _ _ _ _ _ _ _ _ _ _ _ _ _ _ _]
      tunnel: w15 -> [_ _ _ _ _ _ _ _ _ _ _ _ _ _ _ _ _ _ _ _ _ _ _ _ _ _ _ _ _ _ _ _ _ _ _ _ _ _ _ _ _ _ _ _ _ _ w1625 w1646 w1665 _ _ _ _ _ _ _ _ _ _ _ _ _ _ _ _ _ _ _ _ _ _ _ _ _ _ _ _ _ _ _ _ _ _ _ _ _ _ _ _ _ _ _ _ _]
      frame "--------Initialize--------" {
      }
      frame "Init" {
        n5 = Unbundle By Name(w41) -> ("ctl refs.all station status"=w50:refnum<vi>, "ctl refs.Individual Station Status"=w49:refnum<vi>, "misc station config.Station Name"=w48:string, "Application Status"=w36:string, "NVH Configuration"=w47:T6)  [unwired: 2 out]
        n6 = disable-structure shown="启用" {
          disable-tunnel: w48 -> [w72 _]
          disable-tunnel: [w63 w94] -> w38
          disable-tunnel: w37 -> [w62 w94]
          frame Disabled {
            w64 = path "c:/Database"
            n7 = Concatenate Strings(w72, "\\Excel Data\\" ("Audit")) -> (w76:string)
            n8 = Concatenate Strings(w72, "\\AP Data\\") -> (w75:string)
            n9 = Concatenate Strings(w72, "\\Current Data\\") -> (w74:string)
            n10 = Concatenate Strings(w72, "\\Sunshade Force Data\\") -> (w73:string)
            n11 = Concatenate Strings(w72, "\\Data Bytes Log\\" ("Audit")) -> (w71:string)
            n12 = Build Path(base path=w64, name or relative path=w76) -> (appended path=w70:path)
            n13 = Build Path(base path=w64, name or relative path=w75) -> (appended path=w68:path)
            n14 = Build Path(base path=w64, name or relative path=w74) -> (appended path=w67:path)
            n15 = Build Path(base path=w64, name or relative path=w73) -> (appended path=w66:path)
            n16 = Build Path(base path=w64, name or relative path=w71) -> (appended path=w65:path)
            n17 = Build Array(w64, w70, w68, w67, w66, w65) -> (w69:path[])
            n18 = for {
              shift-right: [w85] -> w63
              shift-left: w62 -> [w84]
              tunnel: w69 -> [w82] mode=indexing
              n19 = call <vilib>:"Check if File or Folder Exists.vi"("error in (no error)"=w84, "path"=w82) -> ("error out"=w83:errorcluster, "file or folder exists?"=w87:bool, "dup path"=w86:path)  [unwired: 7 in]
              n20 = case shown="假" w87 {
                tunnel: w86 -> [w89 w93]
                tunnel: [w89 w92] -> _
                tunnel: w83 -> [_ w91]
                tunnel: [errorcluster {"status"=FALSE, "code"=0, "source"=""} ("error out") w90] -> w85
                frame True {
                }
                frame False {
                  n21 = Create Folder(path (use dialog)=w93, error in=w91) -> (created path=w92:path, error out=w90:errorcluster)  [unwired: 1 in, 1 out]
                }
              }
            }
          }
          frame Enabled {
          }
        }
        n22 = Unbundle By Name(w47) -> ("NVH Station?"=w39:bool)
        n23 = property class="Clust (严格)"(reference=w49) -> (reference out=w51:refnum<vi>, error out=w54:errorcluster, "Value"=w53:T51)  [unwired: 1 in]
        n24 = property class="Clust (严格)"(reference=w50) -> (reference out=w58:refnum<vi>, error out=w55:errorcluster, "Value"=w56:T52)  [unwired: 1 in]
        n25 = case shown="真" w39 {
          tunnel: w47 -> [_ w95]
          frame False {
          }
          frame True {
            w96 = NVH_Mode_Control_2.0."Init" ("Mode")
            n26 = call "EOL NVH Inputs Controls Buffer 2.0.vi"("NVH Configuration"=w95, "Mode"=w96) -> ()  [unwired: 5 in, 5 out]
            n27 = call "EOL NVH Outputs Controls Buffer 2.0.vi"("Mode"=w96, "NVH Configuration"=w95) -> ()  [unwired: 8 in, 6 out]
          }
        }
        n28 = Bundle By Name(cluster=w56, "Station Name"=w48) -> (w57:T52)
        n29 = Bundle By Name(cluster=w53, "Station"=w48) -> (w52:T51)
        n30 = property class="Clust (严格)"(reference=w51, error in=w54, "Value"=w52) -> ()  [unwired: 2 out]
        n31 = property class="Clust (严格)"(reference=w58, error in=w55, "Value"=w57) -> ()  [unwired: 2 out]
        n32 = Initialize Array(sgl 0.0 ("element"), 350000 ("dimension size"), 8 ("dimension size")) -> (w42:sgl[][])
        n33 = Empty String/Path?(string/path=w36) -> (empty?=w35:bool)
        n34 = Bundle By Name(cluster=w41, "paths.Base Path"=path "C:/Labview Code", "Application Status"="Init", "misc status.Serial Port Configured?"=FALSE ("Serial Port Configured?"), "Motion Status.Motion"=All_Motions."Idle" ("Current Motion"), "Motion Status.Analog Data"=w42) -> (w60:T1)
        n35 = Select(t=string[] ["Exit"], s=w35, f=string[] ["Init Comm Port", "Check Input"] ("event queue out")) -> (s? t:f=w34:string[])
      }
      frame "Init Comm Port" {
        w101 = 13.5 ("Volt Limit")
        n36 = Unbundle By Name(w122) -> ("ctl refs.Individual Station Status"=w110:refnum<vi>, "rs232 port map.RS232"=w107:refnum<visa-resource-name>, "Store Data.Error Table"=w118:string[][], "rs232 port map.PMAC"=w117:refnum<visa-resource-name>, "rs232 port map.PS Port"=w99:refnum<visa-resource-name>, "misc station config.power supply type"=w102:T20)  [unwired: 2 out]
        n37 = Empty String/Path?(string/path=w107) -> (empty?=w108:bool)
        n38 = case shown="假" w108 {
          tunnel: w107 -> [w133 w134]
          tunnel: w97 -> [w132 w135]
          tunnel: [w131 w135] -> w106
          tunnel: [w130 w134] -> w105
          frame False {
            n39 = call-poly "VISA Configure Serial Port"("VISA resource name"=w133, "error in (no error)"=w132) -> ("VISA resource name out"=w130:refnum<visa-resource-name>, "error out"=w131:errorcluster)  [unwired: 12 in]
          }
          frame True {
          }
        }
        n40 = Empty String/Path?(string/path=w117) -> (empty?=w116:bool)
        n41 = case shown="假" w116 {
          tunnel: w117 -> [w140 w143]
          tunnel: [w139 w143] -> w115
          tunnel: w106 -> [w138 w142]
          tunnel: [w136 w142] -> w100
          frame False {
            n42 = call-poly "VISA Configure Serial Port"("VISA resource name"=w140, "error in (no error)"=w138) -> ("VISA resource name out"=w141:refnum<visa-resource-name>, "error out"=w137:errorcluster)  [unwired: 12 in]
            n43 = VISA Flush I/O Buffer(VISA resource name=w141, error in (no error)=w137) -> (VISA resource name out=w139:refnum<visa-resource-name>, error out=w136:errorcluster)  [unwired: 1 in]
          }
          frame True {
          }
        }
        n44 = Empty String/Path?(string/path=w99) -> (empty?=w103:bool)
        n45 = case shown="假" w103 {
          tunnel: [w128 w129] -> w98
          tunnel: w99 -> [w127 _]
          tunnel: 1 ("No. of Power Supplies") -> [w126 _]
          tunnel: w102 -> [w125 _]
          tunnel: w100 -> [w124 w129]
          tunnel: w101 -> [w123 _]
          frame False {
            n46 = call "EOL Initialize Power Supplies.vi"("Volt Limit"=w123, "Error In"=w124, "power supply model"=w125, "No. of Power Supplies"=w126, "VISA resource name"=w127) -> ("error out"=w128:errorcluster)  [unwired: 6 in]
          }
          frame True {
          }
        }
        n47 = property class="Clust (严格)"(reference=w110) -> (reference out=w114:refnum<vi>, error out=w111:errorcluster, "Value"=w112:T51)  [unwired: 1 in]
        n48 = case shown="错误" w98 {
          selector: w98 -> [w144 w148]
          tunnel: [w146 w151] -> w119
          tunnel: w105 -> [_ w154]
          tunnel: w118 -> [w146 w153]
          tunnel: [TRUE FALSE] -> w109
          tunnel: [w144 w147] -> _
          frame No Error {
          }
          frame Error {
            n49 = Format Into String(initial string="", w154) -> (resulting string=w149:string)  [unwired: 2 in, 1 out]
            n50 = call "EOL Error Table.vi"("Error Description"=w149, "error in"=w148, "Error No."=u16 11, "Error Table In"=w153) -> ("error out"=w147:errorcluster, "Error Table Out"=w151:string[][])  [unwired: 6 in]
          }
        }
        n51 = Bundle By Name(cluster=w112, "Serial Port"=w109, "Glass Voltage"=w101) -> (w113:T51)
        n52 = property class="Clust (严格)"(reference=w114, error in=w111, "Value"=w113) -> ()  [unwired: 2 out]
        n53 = Bundle By Name(cluster=w122, "misc status.Serial Port Configured?"=w109, "Store Data.Error Table"=w119, "misc status.Diag Serial Port"=w105, "rs232 port map.PMAC"=w115, "misc status.PS Voltage"=w101) -> (w121:T1)
      }
      frame "Init Controls" {
        w156 = T53 {"Noise Test"=enum."Not Tested", "Avg Current"=0.0, "Run Time"=0.0, "Speed"=0.0, "Position"=enum."Not Tested"}
        n54 = Unbundle By Name(w158) -> ("ctl refs.Motion Data"=w157:refnum<vi>)
        n55 = property class="Clust (严格)"(reference=w157) -> (reference out=w162:refnum<vi>, error out=w159:errorcluster, "Value"=w160:T54)  [unwired: 1 in]
        n56 = Bundle By Name(cluster=w160, "Shade Close Limits"=w156, "Shade Close Data 2"=w156, "Shade Open Limits"=w156, "Shade Open Data"=w156, "Vent Close Limits"=w156, "Vent Close Data"=w156, "Vent Open Limits"=w156, "Vent Open Data"=w156, "Slide Close Limits"=w156, "Slide Close Data"=w156, "Slide Open Limits"=w156, "Slide Open Data"=w156) -> (w161:T54)
        n57 = property class="Clust (严格)"(reference=w162, error in=w159, "Value"=w161) -> ()  [unwired: 2 out]
      }
      frame "Init Motion" {
        w201 = 0 ("Current Data Index")
        w198 = Pass_Fail_Control."Not Tested"  # Position Test
        w199 = Pass_Fail_Control."Not Tested"  # Noise Test
        n58 = Unbundle By Name(w192) -> ("Direct Control Info.set position"=w169:i32[], "misc status.AP Data Type"=w175:T13, "misc status.Serial Port Configured?"=w185:bool, "misc status.PS Voltage"=w195:dbl, "Sequence State.Step Data String"=w200:string, "Motion Status.Analog Data"=w189:sgl[][], "Store Data.Motion Data Array"=w179:T11[], "Motion Status.Motion"=w173:T3, "misc status.Part Setup.Communication Type"=w171:T27, "Direct Control Info.Derect control"=w164:bool, "manual control(direct)"=w165:bool)
        n59 = call "Inalfa SCU LIN Message to Move.vi"("Communication Type"=w171, "Motion"=w173) -> ("Have Swtich?"=w167:bool)  [unwired: 9 in]
        n60 = Empty String/Path?(string/path=w200) -> (empty?=w172:bool)
        n61 = Compound Arithmetic op=AND ("复合运算")(w167, invert w164) -> (w166:bool)
        n62 = Compound Arithmetic op=OR ("复合运算")(w165, w172, w166) -> (w170:bool)
        n63 = Array Size(array=w189) -> (size(s)=w188:i32[])
        n64 = case shown="真" w170 {
          tunnel: T12 {"Power Supply Voltage"=13.0, "Min Avg Current"=0.0, "Max Avg Current"=0.0, "Min Run Time"=0.0, "Max Run Time"=0.0, "Min Speed"=0.0, "Max Speed"=0.0, "AP Data % of Threshold"=0.0, "Travel Distance"=0.0, "AP Data Type"=enum."91/61", "Check Current"=FALSE, "Check Run Time"=FALSE, "Check Speed"=FALSE, "Express Motion?"=FALSE, "Check Sound Test"=FALSE, "Check Position?"=FALSE, "Collect AP Data"=FALSE, "Inital Position"=0, "End Position"=0, "Goto Posiition"=0, "Max max Current"=0.0, "Min max Current"=0.0, "Check max Current"=FALSE, "Check Sound"=FALSE, "Min Sound (dB)"=0.0, "Max Sound (dB)"=0.0, "SW Mode"=enum."Hard Switch", "LIN Msg"={"ID"=0, "Msg"=[], "LDF"="EX1H"}} ("Motion Data Cluster") -> [w225 w231]
          tunnel: [w214 w230] -> w183
          tunnel: w200 -> [w221 _]
          tunnel: [w224 w229] -> w177
          tunnel: w195 -> [_ w229]
          tunnel: w194 -> [w223 w228]
          tunnel: [w222 w228] -> w193
          tunnel: w185 -> [_ _]
          tunnel: [w218 w227] -> w176
          tunnel: w175 -> [_ w227]
          tunnel: [w213 w226] -> w168
          tunnel: w169 -> [_ w226]
          frame False {
            n65 = Unflatten From String(type=w225, binary string=w221, error in (no error)=w223) -> (value=w219:T12, error out=w220:errorcluster)  [unwired: 2 in, 1 out]
            n66 = call "convert motion step with u8 positions to u16.vi"("error in"=w220, "data string"=w221, "Motion Data Cluster in"=w219) -> ("error out"=w222:errorcluster, "Motion Data Cluster out"=w214:T12)  [unwired: 7 in]
            n67 = Unbundle By Name(w214) -> ("Inital Position"=w217:u16, "End Position"=w216:u16, "Goto Posiition"=w215:u16)
            n68 = Unbundle By Name(w214) -> ("Power Supply Voltage"=w224:dbl, "AP Data Type"=w218:T13)
            n69 = Build Array(w217, w216, w215) -> (w213:u16[])
          }
          frame True {
            n70 = Bundle By Name(cluster=w231, "Power Supply Voltage"=w229, "AP Data Type"=w227) -> (w230:T12)
          }
        }
        n71 = Index Array(array=w188) -> (element #1=w187:i32, element #2=w186:i32)  [unwired: 2 in]
        n72 = for {
          N: w187 -> [_]
          shift-right: [w206] -> w190
          shift-left: w189 -> [w207]
          tunnel: w186 -> [w205]
          i -> [w204]
          n73 = for {
            N: w205 -> [_]
            shift-right: [w210] -> w206
            shift-left: w207 -> [w211]
            tunnel: w204 -> [w209]
            i -> [w208]
            n74 = in-place {
              n75 = in-place-array #1(w211, w209, w208) -> ()  [unwired: 1 out]
              n76 = in-place-array #1(sgl 0.0 ("element")) -> (w210:sgl[][])  [unwired: 2 out]
            }
          }
        }
        n77 = Initialize Array(0.0 ("element"), 8 ("dimension size")) -> (w182:dbl[])
        n78 = Bundle By Name(cluster=T11 {"Motion"=enum."Glass Teach", "Actual Avg Current"=0.0, "Actual Runtime"=0.0, "Actual Speed"=0.0, "Current Data"=[], "Motion Data Limits"={"Power Supply Voltage"=0.0, "Min Avg Current"=0.0, "Max Avg Current"=0.0, "Min Run Time"=0.0, "Max Run Time"=0.0, "Min Speed"=0.0, "Max Speed"=0.0, "AP Data % of Threshold"=10.0, "Travel Distance"=0.0, "AP Data Type"=enum."91/61", "Check Current"=FALSE, "Check Run Time"=FALSE, "Check Speed"=FALSE, "Express Motion?"=FALSE, "Check Sound Test"=FALSE, "Check Position?"=FALSE, "Collect AP Data"=FALSE, "Inital Position"=0, "End Position"=0, "Goto Posiition"=0, "Max max Current"=0.0, "Min max Current"=0.0, "Check max Current"=FALSE, "Check Sound"=FALSE, "Min Sound (dB)"=0.0, "Max Sound (dB)"=0.0, "SW Mode"=enum."Hard Switch", "LIN Msg"={"ID"=0, "Msg"=[], "LDF"="EX1H"}}, "Switch 1 to 6"=[], "Actual PS Voltage"=0.0, "AP Data"=[], "Actual max Current"=0.0, "Actual Noise (dB)"=0.0} ("Motion Data"), "Motion Data Limits"=w183, "Switch 1 to 6"=w182, "Motion"=w173) -> (w180:T11)
        n79 = Build Array (concatenate)(w179, w180) -> (w178:T11[])
        n80 = Bundle By Name(cluster=w192, "Direct Control Info.set position"=w168, "misc status.AP Data Type"=w176, "misc status.PS Voltage"=w177, "Motion Status.Current Data Index"=w201, "Motion Status.Messages Index"=w201, "Motion Status.Analog Data"=w190, "Motion Status.Noise Test"=w199, "Motion Status.Position Test"=w198, "Motion Status.motion stop check initialized"=FALSE ("motion stop check initialized"), "Store Data.Motion Data Array"=w178, "Decibel data"=dbl[] []) -> (w202:T1)
      }
      frame "Init Test" {
        w241 = FALSE ("Operator Action?")
        w253 = TRUE ("NVH Operator?")
        w288 = FALSE ("Ext Diag Mode?")
        w291 = TRUE ("Cycling?")
        w289 = u8 0 ("Motion Index")
        n81 = Unbundle By Name(w239) -> ("ctl refs.Route to Repair"=w233:refnum<vi>, "ctl refs.Red-Rabbit Mode"=w234:refnum<vi>, "Motion Status.Analog Data"=w232:sgl[][], "ctl refs.Individual Station Status"=w236:refnum<vi>, "ctl refs.all station status"=w235:refnum<vi>, "Config Info"=w238:T34)  [unwired: 1 out]
        n82 = call "Config Info Get.vi"("Config Info"=w238) -> ("PLC Comms"=w237:T56)  [unwired: 7 in, 3 out]
        n83 = Unbundle By Name(w237) -> ("PLC bool write Tags.Test Started"=w282:T40, "PLC bool write Tags.Retract LVDT's"=w281:T40, "PLC bool write Tags.Extend LVDT's"=w280:T40, "PLC bool write Tags.AT set wand home pos"=w266:T40, "PLC bool write Tags.Test Complete Pass"=w264:T40, "PLC bool write Tags.Test Complete Fail"=w263:T40, "PLC bool write Tags.NVH Operator Pass"=w251:T40, "PLC bool write Tags.NVH Operator Fail"=w250:T40, "PLC bool write Tags.NVH Operator Check"=w249:T40, "PLC bool write Tags.NVH Operator Vent Open Noise"=w248:T40, "PLC bool write Tags.NVH Operator Vent Close Noise"=w247:T40, "PLC bool write Tags.NVH Operator Sunshade Open Noise"=w246:T40, "PLC bool write Tags.NVH Operator Sunshade Close Noise"=w245:T40, "PLC bool write Tags.NVH Operator Glass Open Noise"=w244:T40, "PLC bool write Tags.NVH Operator Glass Close Noise"=w243:T40, "PLC bool write Tags.NVH Operator Finish"=w242:T40)
        n84 = Array Size(array=w232) -> (size(s)=w262:i32[])
        n85 = Build Array(w264, w263, w282, w281, w280, w266, w251, w250, w249, w248, w247, w246, w245, w244, w243, w242) -> (w279:T40[])
        n86 = property class="Clust (严格)"(reference=w235) -> (reference out=w275:refnum<vi>, error out=w272:errorcluster, "Value"=w273:T52)  [unwired: 1 in]
        n87 = Bundle By Name(cluster=w273, "Error Table Br"=string[][] [] ("Error Table Au"), "Pass / Fail"=u32 13816530 ("Pass/Fail AU"), "NVH System"=FALSE ("B&K System"), "Database LVDT's Data Out"=T35[] []) -> (w274:T52)
        n88 = Index Array(array=w262) -> (element #1=w261:i32, element #2=w260:i32)  [unwired: 2 in]
        n89 = disable-structure shown="启用" {
          disable-tunnel: w283 -> [w301 _]
          disable-tunnel: w279 -> [w300 _]
          disable-tunnel: bool[] [FALSE, FALSE, TRUE, FALSE, FALSE, TRUE, FALSE, FALSE, FALSE, FALSE, FALSE, FALSE, FALSE, FALSE, FALSE, FALSE] -> [w299 _]
          disable-tunnel: [w295 _] -> w277
          disable-tunnel: w266 -> [w294 _]
          frame Enabled {
            n90 = for {
              tunnel: w300 -> [w313] mode=indexing
              shift-right: [w316] -> w296
              shift-left: w301 -> [w317]
              tunnel: w299 -> [w312] mode=indexing
              n91 = Unbundle By Name(w313) -> ("Tag Name"=w314:string)
              n92 = Wait Until Next ms Multiple(millisecond multiple=u32 10 ("milliseconds to wait")) -> ()  [unwired: 1 out]
              n93 = Empty String/Path?(string/path=w314) -> (empty?=w315:bool)
              n94 = case shown="假" w315 {
                tunnel: w317 -> [w320 w322]
                tunnel: w314 -> [_ _]
                tunnel: [w321 w322] -> w316
                tunnel: w313 -> [w319 _]
                tunnel: w312 -> [w318 _]
                frame False {
                  n95 = call "plc write bool.vi"("error in"=w320, "value"=w318, "addr,tag"=w319) -> ("error out"=w321:errorcluster)  [unwired: 8 in]
                }
                frame True {
                }
              }
            }
            n96 = Unbundle By Name(w294) -> ("Tag Name"=w298:string)
            n97 = Empty String/Path?(string/path=w298) -> (empty?=w297:bool)
            n98 = case shown="真" w297 {
              tunnel: w296 -> [w306 w310]
              tunnel: [w305 w310] -> w295
              tunnel: w294 -> [w302 _]
              frame False {
                n99 = flat-sequence {
                  tunnel: [w307] -> w304
                  tunnel: w306 -> [w307]
                  frame #0 {
                    n100 = Wait (ms)(milliseconds to wait=u32 1000) -> ()  [unwired: 1 out]
                  }
                }
                n101 = call "plc write bool.vi"("error in"=w304, "value"=FALSE, "addr,tag"=w302) -> ("error out"=w305:errorcluster)  [unwired: 8 in]
              }
              frame True {
                # "delay to give plc\nchance to reset\nabort discrete signal"
                n102 = Wait (ms)(milliseconds to wait=u32 100) -> ()  [unwired: 1 out]
              }
            }
          }
          frame Disabled {
          }
        }
        n103 = for {
          N: w261 -> [_]
          shift-right: [w325] -> w259
          shift-left: w232 -> [w326]
          tunnel: w260 -> [w324]
          i -> [w323]
          n104 = for {
            N: w324 -> [_]
            shift-right: [w329] -> w325
            shift-left: w326 -> [w330]
            tunnel: w323 -> [w328]
            i -> [w327]
            n105 = in-place {
              n106 = in-place-array #2(w330, w328, w327) -> ()  [unwired: 1 out]
              n107 = in-place-array #2(sgl 0.0 ("element")) -> (w329:sgl[][])  [unwired: 2 out]
            }
          }
        }
        n108 = property class="Clust (严格)"(reference=w236) -> (error out=w258:errorcluster, "Value"=w268:T51)  [unwired: 1 in, 1 out]
        n109 = property class="Clust (严格)"(reference=w275, error in=w272, "Value"=w274) -> ()  [unwired: 2 out]
        n110 = Unbundle By Name(w268) -> ("Line Number"=w267:u8)
        n111 = property class="Bool (严格)"(reference=w234, error in=w258) -> (error out=w256:errorcluster, "Value"=w257:bool)  [unwired: 1 out]
        n112 = property on="Property Node" class="Bool (严格)"(reference=w233, error in=w256) -> ("Value"=w255:bool)  [unwired: 2 out]
        n113 = call "EOL All-Station Module Test Data Buffer.vi"() -> ("Store Data out"=w276:T10)  [unwired: 11 in]
        n114 = Tick Count (ms)() -> (millisecond timer value=w286:u32)
        n115 = Bundle By Name(cluster=w239, "Operator Pass?"=w253, "NVH Pass?"=w253, "NVH Operator?"=w253, "Sequence State.NVH Status.Restart IRQ Counter"=w289, "Sequence State.Active Step"=w289, "Application Status"="Test Started", "Motion Status.Motion"=All_Motions."Idle" ("Current Motion"), "Sequence State.Testing?"=w291, "Sequence State.Pass?"=w291, "misc status.Diag Mode?"=w288, "misc status.In Vehicle Mode?"=w288, "Sequence State.NVH Status.NVH Test Needed?"=w288, "Store Data.Error Table"=string[][] [] ("Error Table"), "Motion Status.Analog Data"=w259, "Sequence State.Cycle Start Time"=w286, "Sequence State.Red-Rabbit Mode"=w257, "misc status.Plant Number"=w267, "AP Test Data.Database AP Data"=dbl[] [0.0, 0.0, 0.0, 50.0, 0.0, 0.0, 0.0, 0.0, 0.0] ("Database AP Data"), "Store Data"=w276, "Sequence State.route-to-repair mode"=w255, "Motion Status.Current Hall Position"=i16 0, "Store Data.data bytes log"="", "Operator Action?"=w241, "Noise Source"=u32 0, "Second Check?"=w241, "Direct Control Info.teach pass"=w241) -> (w287:T1)
      }
      frame "Initialize NVH Test" {
        n116 = Unbundle By Name(w335) -> ("ctl refs.all station status"=w333:refnum<vi>, "NVH Configuration.NVH Station?"=w334:bool, "NVH Configuration"=w332:T6)
        n117 = case shown="真" w334 {
          tunnel: w338 -> [w339 w351]
          tunnel: [w339 w350] -> w337
          tunnel: [w340 w349] -> w336
          tunnel: w335 -> [w340 w348]
          tunnel: w333 -> [_ w343]
          tunnel: w332 -> [_ w342]
          frame False {
          }
          frame True {
            w357 = T61[] [enum."Online", enum."Ready for Model"] items=["Online", "Pass", "Fail", "Testing", "Ready for Model", "Error Bit 1", "Error Bit 2", "Error Bit 3", "Failure Bit 1", "Failure Bit 2", "Failure Bit 3", "Failure Bit 4", "Echo Bit 1", "Echo Bit 2", "Echo Bit 3", "Echo Bit 4", "Serial Number Read Ok", "Ready for Serrial Number"] ("B&K Inputs Control")
            n118 = property class="Clust (严格)"(reference=w343) -> (reference out=w347:refnum<vi>, error out=w344:errorcluster, "Value"=w345:T52)  [unwired: 1 in]
            n119 = call "EOL NVH Inputs Controls Buffer 2.0.vi"("NVH Configuration"=w342, "NVHK Inputs Control"=w357, "Mode"=NVH_Mode_Control_2.0."Read") -> ("NVH Inputs Out"=w352:bool[])  [unwired: 4 in, 4 out]
            n120 = Index Array(array=w352) -> (element #1=w341:bool, element #2=w356:bool)  [unwired: 2 in]
            n121 = Bundle By Name(cluster=w345, "NVH System"=w341) -> (w346:T52)
            n122 = Bundle By Name(cluster=w348, "Sequence State.NVH Status.NVH Test Running?"=w341) -> (w349:T1)
            n123 = Compound Arithmetic op=AND(w341, invert w356) -> (w355:bool)
            n124 = property class="Clust (严格)"(reference=w347, error in=w344, "Value"=w346) -> ()  [unwired: 2 out]
            n125 = Select(t=string[] ["NVH Check Echo"] ("event queue out"), s=w355, f=string[] ["NVH Restart IRQ"] ("event queue out")) -> (s? t:f=w359:string[])
            n126 = call "Insert Multiple Events.vi"("Events to Insert"=w359, "Event queue in"=w351) -> ("Event queue out"=w350:string[])  [unwired: 2 in, 3 out]
          }
        }
      }
      frame "--------Test Loop--------" {
      }
      frame "Start Test" {
      }
      frame "Abort Test" {
        n127 = Unbundle By Name(w375) -> ("Store Data.Error Table"=w377:string[][], "Sequence State"=w368:T24)
        n128 = call "EOL Error Table.vi"("error in"=w372, "Error No."=u16 28, "Error Table In"=w377) -> ("error out"=w371:errorcluster, "Error Table Out"=w374:string[][])  [unwired: 7 in]
        n129 = call "pass fail action decision.vi"("Pass?"=FALSE, "Sequence State in"=w368, "event queue in"=string[] []) -> ("Sequence State out"=w366:T24, "Event queue out"=w367:string[])  [unwired: 7 in]
        n130 = Bundle By Name(cluster=w375, "Store Data.Error Table"=w374, "Sequence State"=w366, "Sequence State.Testing?"=FALSE) -> (w376:T1)
      }
      frame "Check Input" {
        w384 = FALSE ("Testing?")
        n131 = Unbundle By Name(w408) -> ("NVH Configuration"=w388:T6, "Station Index"=w389:i32, "ctl refs.Individual Station Status"=w400:refnum<vi>, "ctl refs.Manual Control"=w397:refnum<vi>, "ctl refs.Start Test"=w396:refnum<vi>, "ctl refs.exit program"=w395:refnum<vi>, "misc status.Serial Port Configured?"=w399:bool, "ctl refs.Direct Manual Ctrl"=w381:refnum<vi>, "D in map.Start Test"=w382:T17, "D in map.Abort Test"=w407:T17)
        n132 = Wait (ms)(milliseconds to wait=u32 100) -> ()  [unwired: 1 out]
        n133 = Build Array(w382, w407) -> (w386:T17[])
        n134 = call "EOL Digital Inputs v2.vi"("Sys Error In"=w385, "Digital Inputs Array"=w386, "Mode"=enum16{"Init", "Read", "Read All", "Close"}."Read") -> ("Sys Error Out"=w394:errorcluster, "DI Status"=w419:bool[])  [unwired: 6 in, 1 out]
        n135 = call "Elapsed Time"("Time Target (s)"=2.0) -> ("Time has Elapsed"=w390:bool)  [unwired: 11 in, 7 out]
        n136 = case shown="真" w390 {
          tunnel: w389 -> [_ w431]
          tunnel: w388 -> [_ w423]
          frame False {
          }
          frame True {
            n137 = call "EOL All-Station AI Circular Data Buffer.vi"("station idx"=w431, "Mode"=enum16{"Initialize", "Read", "Write"}."Read") -> ("Data Read (Samp-Ro, Ch-Col)"=w425:sgl[][])  [unwired: 9 in]
            n138 = Index Array(array=w425, index (col)=EOL_Analog_Input_Control."Motor Current" ("Analog Control")) -> (element=w428:sgl[])  [unwired: 1 in]
            n139 = Array Size(array=w428) -> (size(s)=w430:i32)
            n140 = Add Array Elements(numeric array=w428) -> (sum=w429:sgl)
            n141 = Divide(x=w429, y=w430) -> (x/y=w427:sgl)
            n142 = call "EOL NVH Outputs Controls Buffer 2.0.vi"("Mode"=NVH_Mode_Control_2.0."Write Ambient TempF", "NVH Configuration"=w423, "ambient  temp (deg F)"=w427) -> ()  [unwired: 7 in, 6 out]
          }
        }
        n143 = property class="Clust (严格)"(reference=w400, error in=w394) -> (reference out=w404:refnum<vi>, error out=w401:errorcluster, "Value"=w402:T51)
        n144 = Bundle By Name(cluster=w402, "Serial Port"=w399) -> (w403:T51)
        n145 = property class="Clust (严格)"(reference=w404, error in=w401, "Value"=w403) -> (error out=w393:errorcluster)  [unwired: 1 out]
        n146 = property on="Property Node" class="Bool (严格)"(reference=w397, error in=w393) -> (error out=w392:errorcluster, "Value"=w406:bool)  [unwired: 1 out]
        n147 = property on="Property Node" class="Bool (严格)"(reference=w396, error in=w392) -> (error out=w387:errorcluster, "Value"=w405:bool)  [unwired: 1 out]
        n148 = Index Array(array=w419) -> (element #1=w418:bool, element #2=w410:bool)  [unwired: 2 in]
        n149 = Compound Arithmetic op=AND(w418, invert w410) -> (w409:bool)
        n150 = Or(x=w405, y=w409) -> (x .or. y?=w414:bool)
        n151 = property on="Property Node" class="Bool (严格)"(reference=w395, error in=w387) -> (error out=w380:errorcluster, "Value"=w398:bool)  [unwired: 1 out]
        n152 = Bundle By Name(cluster=w408, "Application Status"="Idle", "Sequence State.Testing?"=w384, "Sequence State.Hold Mode?"=w384, "Sequence State.Hold?"=w384, "Sequence State.Rx Invalid?"=w384) -> (w412:T1)
        n153 = property on="Property Node" class="Bool (严格)"(reference=w381, error in=w380) -> (error out=w378:errorcluster, "Value"=w379:bool)  [unwired: 1 out]
        n154 = Build Array(w406, w414, w398, w379) -> (w417:bool[])
        n155 = Search 1D Array(1D array=w417, element=TRUE) -> (index of element=w415:i32)  [unwired: 1 in]
        n156 = Increment(x=w415) -> (x+1=w413:i32)
        n157 = case shown="1" w413 {
          tunnel: [string[] ["Check Input"] ("f") string[] ["Start Test"] ("t") string[] ["Exit"] ("t") string[] ["Direct Manual Control", "Check Input"] ("t") string[] ["Manual Control", "Check Input"] ("t")] -> w411
          frame 0, Default {
          }
          frame 2 {
          }
          frame 3 {
          }
          frame 4 {
          }
          frame 1 {
          }
        }
        n158 = call <vilib>:"Clear Errors.vi"("error in (no error)"=w378) -> ("error out"=w383:errorcluster)  [unwired: 5 in, 1 out]
      }
      frame "Check Current Data" {
        n159 = Unbundle By Name(w466) -> ("Station Index"=w446:i32, "misc status.Part Setup.Motor Type"=w463:T30, "Sequence State"=w460:T24, "Store Data.Error Table"=w467:string[][], "Store Data.Motion Data Array"=w453:T11[], "Motion Status.Motion"=w441:T3, "Decibel data"=w443:dbl[])
        n160 = Array Size(array=w453) -> (size(s)=w456:i32)
        n161 = Decrement(x=w456) -> (x-1=w455:i32)
        n162 = Index Array(array=w453, index=w455) -> (element=w451:T11)
        n163 = Unbundle By Name(w451) -> ("Motion Data Limits"=w442:T12)
        n164 = call "EOL All-Station AI Debug Buffer Speed.vi"("station idx"=w446, "Mode"=enum16{"Initialize", "Read", "Write"}."Read") -> ("Data Read (Samp-Ro, Ch-Col)"=w445:sgl[][])  [unwired: 9 in]
        n165 = call "EOL Check Current Data.vi"("Motor Type"=w463, "Motion Data"=w445, "Decibel data"=w443, "Current Motion"=w441, "Audit Motion Data Cluster"=w442, "Error Table In"=w467) -> ("max Current"=w448:dbl, "Current Out"=w450:sgl[], "Pass? Out"=w461:bool, "Run Time"=w439:dbl, "Sound (dB)"=w444:dbl, "Avg Current"=w440:dbl, "Error Table Out"=w464:string[][], "Speed"=w438:dbl)  [unwired: 2 in]
        n166 = Bundle By Name(cluster=w451, "Current Data"=w450, "Actual Runtime"=w439, "Actual Avg Current"=w440, "Actual Speed"=w438, "Actual max Current"=w448, "Actual Noise (dB)"=w444) -> (w454:T11)
        n167 = call "pass fail action decision.vi"("fail behavior"=failure_behaviors."stop at next 'check sequence' if not rabbit", "Pass?"=w461, "Sequence State in"=w460, "event queue in"=w458) -> ("Sequence State out"=w459:T24, "Event queue out"=w457:string[])  [unwired: 6 in]
        n168 = Replace Array Subset(array=w453, new element=w454, index=w455) -> (w452:T11[])
        n169 = Bundle By Name(cluster=w466, "Store Data.Motion Data Array"=w452, "Sequence State"=w459, "Store Data.Error Table"=w464) -> (w465:T1)
      }
      frame "Check Digital Input" {
        n170 = Unbundle By Name(w482) -> ("Sequence State"=w468:T24, "Sequence State.Step Data String"=w480:string, "Sequence State.Step Description"=w476:string, "Store Data.Error Table"=w479:string[][])
        n171 = call "State Check Digital Input 2.0.vi"("Sys Error In"=w474, "Step Description"=w476, "Step Data String"=w480) -> ("Sys Error Out"=w473:errorcluster, "Error No."=w478:u16, "Error String"=w475:string, "Pass?"=w472:bool)  [unwired: 5 in]
        n172 = case shown="假" w472 {
          tunnel: w479 -> [w486 w487]
          tunnel: [w485 w487] -> w477
          tunnel: w475 -> [w484 _]
          tunnel: w478 -> [w483 _]
          frame False {
            n173 = call "EOL Error Table.vi"("Error Description"=w484, "Error No."=w483, "Error Table In"=w486) -> ("Error Table Out"=w485:string[][])  [unwired: 7 in, 1 out]
          }
          frame True {
          }
        }
        n174 = call "pass fail action decision.vi"("Pass?"=w472, "Sequence State in"=w468, "event queue in"=w471) -> ("Sequence State out"=w469:T24, "Event queue out"=w470:string[])  [unwired: 7 in]
        n175 = Bundle By Name(cluster=w482, "Sequence State"=w469, "Store Data.Error Table"=w477) -> (w481:T1)
      }
      frame "Check Goto Step" {
        n176 = Unbundle By Name(w499) -> ("Sequence State.Active Step"=w507:u8, "Sequence State.Step Data String"=w488:string)
        n177 = Unflatten From String(type=T39 {"Data Boolean"=FALSE, "PLC Path and Tag"={"Tag Name"="S060.PXI.Signals.PlltData.SN", "Network Path"="172.15.51.1,1,0", "use opc"=FALSE, "DataSocket Reference"={"CWDSLib._DCWDataSocket"=refnum, "CWDSLib._DCWData"=refnum, "OnDataUpdated"=0, "OnStatusUpdated"=0}}, "goto step"=0}, binary string=w488, error in (no error)=w495) -> (value=w492:T39, error out=w497:errorcluster)  [unwired: 2 in, 1 out]
        n178 = Unbundle By Name(w492) -> ("Data Boolean"=w491:bool, "PLC Path and Tag"=w490:T40, "goto step"=w489:u8)
        n179 = Bundle By Name(cluster=T42 {"Data Boolean"=FALSE, "PLC Path and Tag"={"Tag Name"="", "Network Path"="", "use opc"=FALSE, "DataSocket Reference"={"CWDSLib._DCWDataSocket"=refnum, "CWDSLib._DCWData"=refnum, "OnDataUpdated"=0, "OnStatusUpdated"=0}}, "Error No."=157, "timeout (ms)"=0, "Continue on Fail for Red-Rabbit"=FALSE} ("RSLinx String Cluster in"), "Data Boolean"=w491, "PLC Path and Tag"=w490, "Error No."=u16 0, "timeout (ms)"=0) -> (w502:T42)
        n180 = Flatten To String(anything=w502, error in (no error)=w497) -> (data string=w501:string, error out=w498:errorcluster)  [unwired: 2 in, 1 out]
        n181 = call "State Check RSLinx Tag Boolean 2.0.vi"("Sys Error In"=w498, "Main State Cluster"=w499, "Step Data String"=w501) -> ("Sys Error Out"=w493:errorcluster, "Pass?"=w500:bool)  [unwired: 4 in, 3 out]
        n182 = case shown="真" w500 {
          tunnel: [w513 w519] -> w508
          tunnel: w509 -> [w513 w518]
          tunnel: w489 -> [_ w516]
          tunnel: [w512 w515] -> w506
          tunnel: w507 -> [w512 _]
          tunnel: [w511 w517] -> w494
          tunnel: w493 -> [w511 w517]
          frame False {
          }
          frame True {
            # "*** -2 becuase sequence definition number are base 1, but seqeuence exe step numbers are base 0.  also, the 'check sequence' state increments the step number"
            n183 = Subtract(x=w516, y=2) -> (x-y=w515:i32)
            n184 = call "Insert Multiple Events.vi"("Events to Insert"=string[] ["Check Sequence"], "Event queue in"=w518) -> ("Event queue out"=w519:string[])  [unwired: 5 in]
          }
        }
        n185 = Bundle By Name(cluster=w499, "Sequence State.Active Step"=w506) -> (w510:T1)
      }
      frame "Check Initial Motion" {
        n186 = Unbundle By Name(w535) -> ("Sequence State"=w532:T24, "Motion Status.Analog Data"=w538:sgl[][], "Motion Status.Current Data Index"=w537:i32, "Motion Status.Motion"=w527:T3, "Store Data.Error Table"=w540:string[][], "Station Index"=w526:i32, "misc status.Part Setup.Motor Type"=w534:T30)
        n187 = call "EOL Check Initial Motion.vi"("Motor Type"=w534, "Station Index"=w526, "Error Table In"=w540, "Current Motion"=w527, "Current Data Index"=w537, "Current Data"=w538) -> ("Error Table"=w539:string[][], "Pass?"=w522:bool, "Current Data Index Out"=w536:i32, "Current Data Out"=w525:sgl[][])  [unwired: 2 in]
        n188 = call "pass fail action decision.vi"("Pass?"=w522, "Sequence State in"=w532, "event queue in"=w533) -> ("Sequence State out"=w531:T24, "Event queue out"=w530:string[])  [unwired: 7 in]
        n189 = Not(x=w522) -> (.not. x?=w521:bool)
        n190 = Bundle By Name(cluster=w535, "Sequence State"=w531, "Motion Status.Analog Data"=w525, "Motion Status.Current Data Index"=w536, "Store Data.Error Table"=w539) -> (w523:T1)
        n191 = call "Insert Multiple Events.vi"("Insert all? (T)"=w521, "Events to Insert"=string[] ["Reset Switch Outputs"], "Event queue in"=w530) -> ("Event queue out"=w529:string[])  [unwired: 4 in]
      }
      frame "Check Motion Stop Current" {
        w541 = 160 ("length")
        n192 = Unbundle By Name(w554) -> ("Motion Status.Motion"=w558:T3, "Motion Status.Motion Stop Timer"=w574:u32, "Motion Status.Analog Data"=w565:sgl[][], "Motion Status.Current Data Index"=w570:i32, "misc status.Part Setup.Motor Type"=w566:T30, "Motion Status.motion stop check initialized"=w560:bool, "Operator Action?"=w557:bool)
        n193 = Unbundle By Name(w554) -> ("Station Index"=w553:i32)
        n194 = case shown="0, 默认" w553 {
          tunnel: enum16{"Read", "Write"}."Read" ("Mode") -> [w578 w580 w582 w584 w586 w588]
          tunnel: [w577 w579 w581 w583 w585 w587] -> w551
          frame 0, Default {
            n195 = call-poly "EOL_GetPS Data.vi"("Mode"=w578) -> ("out(ALL)"=w577:dbl[])  [unwired: 9 in, 1 out]
          }
          frame 1 {
            n196 = call-poly "EOL_GetPS Data.vi"("Mode"=w580) -> ("out(ALL)"=w579:dbl[])  [unwired: 9 in, 1 out]
          }
          frame 2 {
            n197 = call-poly "EOL_GetPS Data.vi"("Mode"=w582) -> ("out(ALL)"=w581:dbl[])  [unwired: 9 in, 1 out]
          }
          frame 3 {
            n198 = call-poly "EOL_GetPS Data.vi"("Mode"=w584) -> ("out(ALL)"=w583:dbl[])  [unwired: 9 in, 1 out]
          }
          frame 4 {
            n199 = call-poly "EOL_GetPS Data.vi"("Mode"=w586) -> ("out(ALL)"=w585:dbl[])  [unwired: 9 in, 1 out]
          }
          frame 5 {
            n200 = call-poly "EOL_GetPS Data.vi"("Mode"=w588) -> ("out(ALL)"=w587:dbl[])  [unwired: 9 in, 1 out]
          }
        }
        n201 = Tick Count (ms)() -> (millisecond timer value=w575:u32)
        n202 = case shown="\"Glass Teach\", \"Sunshade Teach\", \"Sunshade Teach 2\"" w558 {
          tunnel: [u32 6000 ("y") u32 1000 ("y")] -> w567
          tunnel: [TRUE FALSE] -> _
          frame "Glass Teach", "Sunshade Teach", "Sunshade Teach 2" {
            (unwired) u32 2000 ("y")
            (unwired) u32 7000 ("y")
          }
          frame Default {
            (unwired) u32 500 ("y")
          }
        }
        n203 = call "select current channel.vi"("Current Motion"=w558, "Motor Type"=w566) -> ("Analog channel"=w563:T37)  [unwired: 9 in]
        n204 = Array Max & Min(array=w551) -> (max value=w548:dbl)  [unwired: 3 out]
        n205 = Subtract(x=w570, y=w541) -> (x-y=w564:i32)
        n206 = Equal To 0?(x=w551) -> (x = 0?=w550:bool[])
        n207 = And Array Elements(Boolean array=w550) -> (logical AND=w545:bool)
        n208 = Less Or Equal?(x=w548, y="HWcurrent limt") -> (x <= y?=w544:bool)
        n209 = Subtract(x=w575, y=w574) -> (x-y=w573:u32)
        n210 = Array Subset(array=w565, index (row)=w564, length (row)=w541, index (col)=w563, length (col)=1 ("length")) -> (w547:sgl[][])
        n211 = Less Or Equal?(x=w547, y="HWcurrent limt") -> (x <= y?=w571:bool[][])
        n212 = Empty Array?(array=w547) -> (empty?=w556:bool)
        n213 = And Array Elements(Boolean array=w571) -> (logical AND=w546:bool)
        n214 = Not(x=w556) -> (.not. x?=w555:bool)
        n215 = Greater Or Equal?(x=w573, y=w567) -> (x >= y?=w572:bool)
        n216 = Select(t=w546, s=w545, f=w544) -> (s? t:f=w549:bool)
        n217 = Compound Arithmetic op=AND(w555, w549, w560) -> (w543:bool)
        n218 = case shown="假" w543 {
          tunnel: [string[] ["Get Data"] ("event queue out") w598] -> w569
          tunnel: w574 -> [_ w597]
          tunnel: [w593 w597] -> w576
          tunnel: w572 -> [_ w596]
          tunnel: w557 -> [_ w595]
          frame False {
            n219 = Tick Count (ms)() -> (millisecond timer value=w593:u32)
          }
          frame True {
            n220 = case shown="假" w596 {
              tunnel: [string[] ["Get Data"] ("event queue out") w601] -> w598
              tunnel: w595 -> [_ w600]
              frame False {
              }
              frame True {
                n221 = case shown="真" w600 {
                  tunnel: [string[] ["Reset Switch Outputs", "Check Current Data", "Display Data", "wait for operator action"] ("event queue out") string[] ["Reset Switch Outputs", "Check Current Data", "NVH Stop Test", "Display Data", "Check Sequence"] ("event queue out")] -> w601
                  frame True {
                  }
                  frame False {
                  }
                }
              }
            }
          }
        }
        n222 = Tick Count (ms)() -> (millisecond timer value=w559:u32)
        n223 = Bundle By Name(cluster=w554, "Motion Status.Analog Data"=w565, "Motion Status.Motion Stop Timer"=w576, "Motion Status.motion stop check initialized"=TRUE ("motion stop check initialized"), "Motion Status.hmi operator abort start time"=w559) -> (w568:T1)
      }
      frame "Check Motor Connection" {
        n224 = Unbundle By Name(w615) -> ("Motion Status.Motion"=w605:T3, "misc status.Part Setup.Communication Type"=w606:T27, "Sequence State"=w608:T24, "Switch Value Configuration"=w612:T4[], "Store Data.Error Table"=w613:string[][], "Station Index"=w611:i32)
        n225 = call "EOL All-Station Check Switch Signals.vi"("Switch Value Configuration"=w612, "Communication Type"=w606, "Motion"=w605, "Check Switch Signals"=All_Motions."Idle", "Error Table In"=w613, "station idx"=w611) -> ("Pass?"=w604:bool, "Error Table Out"=w617:string[][])  [unwired: 5 in, 3 out]
        n226 = call "pass fail action decision.vi"("Pass?"=w604, "Sequence State in"=w608, "event queue in"=w610) -> ("Sequence State out"=w607:T24, "Event queue out"=w609:string[])  [unwired: 7 in]
        n227 = Bundle By Name(cluster=w615, "Sequence State"=w607, "Store Data.Error Table"=w617) -> (w616:T1)
      }
      frame "Check Motor Low Current" {
        n228 = Unbundle By Name(w629) -> ("Sequence State"=w621:T24, "Store Data.Error Table"=w627:string[][], "Motion Status.Analog Data"=w626:sgl[][], "Motion Status.Motion"=w619:T3, "misc status.Part Setup.Motor Type"=w625:T30)
        n229 = call "EOL Check Motor Low Current Detection.vi"("Error Table In"=w627, "Current Motion"=w619, "Current Data"=w626, "Motor Type"=w625) -> ("Pass? Out"=w623:bool, "Error Table Out"=w628:string[][])  [unwired: 6 in]
        n230 = call "pass fail action decision.vi"("fail behavior"=failure_behaviors."stop immediately if not rabbit", "Pass?"=w623, "Sequence State in"=w621, "event queue in"=w624) -> ("Sequence State out"=w620:T24, "Event queue out"=w622:string[])  [unwired: 6 in]
        n231 = Bundle By Name(cluster=w629, "Sequence State"=w620, "Store Data.Error Table"=w628) -> (w630:T1)
      }
      frame "Check Power Data" {
        n232 = Unbundle By Name(w651) -> ("misc station config.power supply type"=w644:T20, "Sequence State"=w641:T24, "rs232 port map.PS Port"=w650:refnum<visa-resource-name>, "misc status.PS Voltage"=w649:dbl, "Store Data.Error Table"=w648:string[][], "misc station config.Station Name"=w646:string, "Station Index"=w645:i32, "misc status.Part Setup.Motor Type"=w643:T30, "Store Data.Motion Data Array"=w634:T11[])
        n233 = case shown="\"Smart Motor\", 默认" w643 {
          tunnel: [EOL_Analog_Input_Control."Motor Voltage" ("Analog Control") EOL_Analog_Input_Control."SW PS  Volage" ("Analog Control")] -> w647
          frame "Smart Motor", Default {
          }
          frame "Sensor Motor" {
          }
        }
        n234 = call "Check Power Data.vi"("PS Channel Control"=w647, "station name"=w646, "power supply type"=w644, "Error Table In"=w648, "station idx"=w645, "Power Supply Voltage"=w649, "Power Supply Comm Port"=w650) -> ("Error Table Out"=w653:string[][], "Actual Voltage"=w633:dbl, "Pass?"=w631:bool)  [unwired: 2 in]
        n235 = Array Size(array=w634) -> (size(s)=w638:i32)
        n236 = Decrement(x=w638) -> (x-1=w637:i32)
        n237 = call "pass fail action decision.vi"("Pass?"=w631, "Sequence State in"=w641, "event queue in"=w642) -> ("Sequence State out"=w640:T24, "Event queue out"=w639:string[])  [unwired: 7 in]
        n238 = Index Array(array=w634, index=w637) -> (element=w636:T11)
        n239 = Bundle By Name(cluster=w636, "Actual PS Voltage"=w633) -> (w635:T11)
        n240 = Replace Array Subset(array=w634, new element=w635, index=w637) -> (w632:T11[])
        n241 = Bundle By Name(cluster=w651, "Sequence State"=w640, "Store Data.Motion Data Array"=w632, "Store Data.Error Table"=w653) -> (w652:T1)
      }
      frame "Check RSLinx Tag String" {
        n242 = Unbundle By Name(w663) -> ("Sequence State"=w658:T24, "Sequence State.Step Data String"=w669:string, "Sequence State.Step Description"=w665:string, "Store Data.Error Table"=w668:string[][])
        n243 = call "State Check RSLinx Tag String 2.0.vi"("Sys Error In"=w662, "Main State Cluster"=w663, "Step Description"=w665, "Step Data String"=w669) -> ("Sys Error Out"=w661:errorcluster, "Error No."=w667:u16, "Error String"=w664:string, "Pass?"=w659:bool)  [unwired: 4 in]
        n244 = case shown="假" w659 {
          tunnel: w668 -> [w674 w675]
          tunnel: [w673 w675] -> w666
          tunnel: w664 -> [w672 _]
          tunnel: w667 -> [w671 _]
          frame False {
            n245 = call "EOL Error Table.vi"("Error Description"=w672, "Error No."=w671, "Error Table In"=w674) -> ("Error Table Out"=w673:string[][])  [unwired: 7 in, 1 out]
          }
          frame True {
          }
        }
        n246 = call "pass fail action decision.vi"("Pass?"=w659, "Sequence State in"=w658, "event queue in"=w660) -> ("Sequence State out"=w657:T24, "Event queue out"=w656:string[])  [unwired: 7 in]
        n247 = Bundle By Name(cluster=w663, "Sequence State"=w657, "Store Data.Error Table"=w666) -> (w670:T1)
      }
      frame "Check RSLinx Tag Boolean" {
        n248 = Unbundle By Name(w687) -> ("Sequence State"=w681:T24, "Sequence State.Step Data String"=w693:string, "Sequence State.Step Description"=w689:string, "Store Data.Error Table"=w692:string[][])
        n249 = call "State Check RSLinx Tag Boolean 2.0.vi"("Sys Error In"=w686, "Main State Cluster"=w687, "Step Description"=w689, "Step Data String"=w693) -> ("Sys Error Out"=w685:errorcluster, "Error No."=w691:u16, "Error String"=w688:string, "Pass?"=w683:bool, "Continue on Fail for Red-Rabbit"=w679:bool)  [unwired: 3 in]
        n250 = case shown="假" w683 {
          tunnel: w692 -> [w698 w699]
          tunnel: [w697 w699] -> w690
          tunnel: w688 -> [w696 _]
          tunnel: w691 -> [w695 _]
          frame False {
            n251 = call "EOL Error Table.vi"("Error Description"=w696, "Error No."=w695, "Error Table In"=w698) -> ("Error Table Out"=w697:string[][])  [unwired: 7 in, 1 out]
          }
          frame True {
          }
        }
        n252 = Select(t=failure_behaviors."stop immediately if not rabbit" ("fail behavior"), s=w679, f=failure_behaviors."stop immediately" ("fail behavior")) -> (s? t:f=w676:T38)
        n253 = call "pass fail action decision.vi"("fail behavior"=w676, "Pass?"=w683, "Sequence State in"=w681, "event queue in"=w684) -> ("Sequence State out"=w680:T24, "Event queue out"=w682:string[])  [unwired: 6 in]
        n254 = Bundle By Name(cluster=w687, "Sequence State"=w680, "Store Data.Error Table"=w690) -> (w694:T1)
      }
      frame "Check Switch Signals" {
        n255 = Unbundle By Name(w720) -> ("Sequence State"=w714:T24, "Switch Value Configuration"=w718:T4[], "Motion Status.Analog Data"=w723:sgl[][], "Motion Status.Current Data Index"=w722:i32, "Store Data.Motion Data Array"=w709:T11[], "Store Data.Error Table"=w724:string[][], "Station Index"=w706:i32, "Motion Status.Motion"=w701:T3, "misc status.Part Setup.Communication Type"=w702:T27)
        n256 = Array Size(array=w709) -> (size(s)=w713:i32)
        n257 = Decrement(x=w713) -> (x-1=w712:i32)
        n258 = Index Array(array=w709, index=w712) -> (element=w710:T11)
        n259 = call "EOL All-Station Check Switch Signals.vi"("Current Data In"=w723, "Switch Value Configuration"=w718, "Communication Type"=w702, "Current Data Index In"=w722, "Motion"=w701, "Check Switch Signals"=w701, "Error Table In"=w724, "station idx"=w706) -> ("Current Data Out"=w705:sgl[][], "Current Data Index Out"=w721:i32, "Pass?"=w700:bool, "Switches 1 to 8"=w708:dbl[], "Error Table Out"=w704:string[][])  [unwired: 3 in]
        n260 = Bundle By Name(cluster=w710, "Switch 1 to 6"=w708) -> (w711:T11)
        n261 = call "pass fail action decision.vi"("Pass?"=w700, "Sequence State in"=w714, "event queue in"=w717) -> ("Sequence State out"=w715:T24, "Event queue out"=w716:string[])  [unwired: 7 in]
        n262 = Replace Array Subset(array=w709, new element=w711, index=w712) -> (w707:T11[])
        n263 = Bundle By Name(cluster=w720, "Sequence State"=w715, "Motion Status.Analog Data"=w705, "Motion Status.Current Data Index"=w721, "Store Data.Error Table"=w704, "Store Data.Motion Data Array"=w707) -> (w719:T1)
      }
      frame "Choose Noise Source" {
        n264 = Unbundle By Name(w736) -> ("Store Data.Error Table"=w738:string[][], "Noise Source"=w730:u32, "Config Info"=w728:T34)
        n265 = call "Config Info Get.vi"("Config Info"=w728) -> ("PLC Comms"=w727:T56)  [unwired: 7 in, 3 out]
        n266 = Unbundle By Name(w727) -> ("PLC boolean read Tags"=w726:T57, "PLC bool write Tags"=w725:T58)
        n267 = Wait (ms)(milliseconds to wait=u32 100) -> ()  [unwired: 1 out]
        n268 = call "check noise source.vi"("PLC bool write Tags"=w725, "Noise Source Input"=w730, "Error Table In"=w738, "input cluster"=w726) -> ("Operator Finish?"=w732:bool, "Noise Source output"=w729:u32, "Error Table Out"=w735:string[][])  [unwired: 5 in]
        n269 = case shown="真" w732 {
          tunnel: [string[] ["Choose Noise Source"] ("Event queue out") string[] ["Sequence Complete"] ("Event queue out")] -> w733
          frame False {
          }
          frame True {
          }
        }
        n270 = Bundle By Name(cluster=w736, "Store Data.Error Table"=w735, "Noise Source"=w729) -> (w737:T1)
      }
      frame "Close Comm Port" {
        n271 = Unbundle By Name(w746) -> ("misc status.Diag Serial Port"=w748:refnum<visa-resource-name>, "misc status.Serial Port Configured?"=w745:bool)
        n272 = Bundle By Name(cluster=w746, "misc status.Serial Port Configured?"=FALSE ("Serial Port Configured?")) -> (w744:T1)
        n273 = case shown="真" w745 {
          tunnel: w748 -> [_ w752]
          tunnel: w742 -> [w749 w751]
          tunnel: [w749 w750] -> w741
          frame False {
          }
          frame True {
            n274 = VISA Close(VISA resource name=w752, error in (no error)=w751) -> (error out=w750:errorcluster)
          }
        }
      }
      frame "Cycle RAP" {
        n275 = Unbundle By Name(w756) -> ("DO Task"=w753:refnum<k21>)
        n276 = flat-sequence {
          tunnel: [w760] -> w754
          tunnel: w753 -> [w758]
          tunnel: [w765] -> w755
          tunnel: w754 -> [w765]
          tunnel: w755 -> [w771]
          tunnel: w753 -> [w767]
          frame #0 {
            n277 = Bundle By Name(cluster=T44 {"Status"=FALSE, "Global DO Ch"=enum."Battery"} ("Cluster"), "Status"=FALSE, "Global DO Ch"=EOL_Global_Digital_Output_Control."IGN High") -> (w760:T44)
            n278 = Build Array(w760) -> (w761:T44[])
            n279 = call "EOL Digital Outputs v3.vi"("task/channels in"=w758, "DO Status"=w761, "Mode"=T45."Write") -> ()  [unwired: 7 in, 2 out]
          }
          frame #1 {
            n280 = Wait (ms)(milliseconds to wait=u32 3000) -> ()  [unwired: 1 out]
          }
          frame #2 {
            n281 = Bundle By Name(cluster=w771, "Status"=TRUE) -> (w769:T44)
            n282 = Build Array(w769) -> (w768:T44[])
            n283 = call "EOL Digital Outputs v3.vi"("task/channels in"=w767, "DO Status"=w768, "Mode"=T45."Write") -> ()  [unwired: 7 in, 2 out]
          }
        }
      }
      frame "Delay" {
        n284 = Unbundle By Name(w786) -> ("Sequence State.Step Data String"=w782:string, "misc status.delay start time (ticks)"=w777:u32)
        n285 = Scan From String(format string="%0.2f", input string=w782) -> (output 1=w783:dbl)  [unwired: 3 in, 3 out]
        n286 = Tick Count (ms)() -> (millisecond timer value=w776:u32)
        n287 = Subtract(x=w776, y=w777) -> (x-y=w775:u32)
        n288 = Multiply(x=w783, y=1000.0) -> (x*y=w774:dbl)
        n289 = Greater Or Equal?(x=w775, y=w774) -> (x >= y?=w773:bool)
        n290 = Not(x=w773) -> (.not. x?=w780:bool)
        n291 = call "Insert Multiple Events.vi"("Insert all? (T)"=w780, "Events to Insert"=string[] ["Delay"], "Event queue in"=w779) -> ("Event queue out"=w778:string[])  [unwired: 4 in]
      }
      frame "DirectControl" {
        n292 = Unbundle By Name(w817) -> ("misc status.Part Setup.Part Type"=w803:string, "ctl refs.all station status"=w810:refnum<vi>, "Motion Status.Analog Data"=w798:sgl[][], "ctl refs.Abort Test"=w807:refnum<vi>, "Store Data.Error Table"=w812:string[][], "Station Index"=w804:i32, "manual control(direct)"=w791:bool, "Direct Control Info.set position"=w802:i32[], "Motion Status.Motion"=w801:T3, "Config Info"=w790:T34)
        n293 = call "Config Info Get.vi"("Config Info"=w790) -> ("PLC Comms"=w789:T56)  [unwired: 7 in, 3 out]
        n294 = Unbundle By Name(w789) -> ("PLC boolean read Tags.NVH Operator Express Rollo Open01"=w788:T40, "PLC boolean read Tags.NVH Operator Express Rollo Close01"=w787:T40)
        n295 = case shown="真" w791 {
          tunnel: [string[] ["Reset Switch Outputs", "Check Current Data", "Check Sequence"] string[] ["Reset Switch Outputs", "Check Current Data", "Manual control operator action", "Check Sequence"]] -> w815
          tunnel: ["Direct Control" "Manual Direct Control"] -> w796
          tunnel: ["CMD-" "ManualCMD-"] -> w793
          frame False {
          }
          frame True {
          }
        }
        n296 = property class="Clust (严格)"(reference=w810) -> ("Controls[]"=w808:refnum<vi>[])  [unwired: 1 in, 2 out]
        n297 = Index Array(array=w808, index=9) -> (element=w800:refnum<vi>)
        n298 = call "MotorDirectControl.vi"("station index"=w804, "Hall Positions"=w802, "JKI_Prefix"=w793, "Exit Refnum"=w807, "Motion"=w801, "PatrType"=w803, "AnalogData in"=w798, "Manual operation"=w791, "open Switch"=w788, "test mode"=FALSE, "close Switch"=w787, "Position Refnum"=w800) -> ("AnalogData out"=w799:dbl[][], "结果"=w806:bool, "Error"=w805:string)  [unwired: 4 in, 1 out]
        n299 = case shown="假" w806 {
          selector: w806 -> [_ w829]
          tunnel: [FALSE ("PASS") w829] -> w797
          tunnel: w812 -> [w826 w830]
          tunnel: [w825 w830] -> w811
          tunnel: w805 -> [w824 _]
          frame False {
            n300 = call "EOL Error Table.vi"("Error Description"=w824, "Error No."=u16 212, "Error Table In"=w826) -> ("Error Table Out"=w825:string[][])  [unwired: 7 in, 1 out]
          }
          frame True {
          }
        }
        n301 = Select(t=w796, s=w797, f="Manual Direct Control") -> (s? t:f=w794:string)
        n302 = Bundle By Name(cluster=w817, "Application Status"=w794, "Motion Status.Analog Data"=w799, "Store Data.Error Table"=w811, "Sequence State.Pass?"=w797, "Direct Control Info.teach pass"=w797) -> (w816:T1)
        n303 = Select(t=w815, s=w797, f=string[] ["direct manual action"]) -> (s? t:f=w813:string[])
      }
      frame "Display Data" {
        n304 = Unbundle By Name(w845) -> ("ctl refs.Motion Data"=w838:refnum<vi>, "Store Data.Motion Data Array"=w833:T11[], "Motion Status.Noise Test"=w842:T21, "Motion Status.Position Test"=w841:T21)
        n305 = Array Size(array=w833) -> (size(s)=w835:i32)
        n306 = Decrement(x=w835) -> (x-1=w834:i32)
        n307 = property class="Clust (严格)"(reference=w838) -> (reference out=w840:refnum<vi>, error out=w839:errorcluster, "Value"=w836:T54)  [unwired: 1 in]
        n308 = Index Array(array=w833, index=w834) -> (element=w831:T11)
        n309 = Unbundle By Name(w831) -> ("Motion"=w832:T3)
        n310 = call "EOL Audit Display Data.vi"("Check Position"=w841, "Check Noise Test"=w842, "Audit Motion Database Table"=w831) -> ("Limits Data"=w843:T55, "Actual Data"=w844:T55)  [unwired: 5 in]
        n311 = case shown="\"Glass Vent Open Sunshade Close\"" w832 {
          tunnel: w844 -> [_ w849 w853 w857 w861 w865 w869 _ _ _ _ _ _ _ _ _ _]
          tunnel: w843 -> [_ w848 w852 w856 w860 w864 w868 _ _ _ _ _ _ _ _ _ _]
          tunnel: [w847 w850 w854 w858 w862 w866 w870 w872 w873 w874 w875 w876 w877 w878 w879 w880 w881] -> w837
          tunnel: w836 -> [w847 w851 w855 w859 w863 w867 w871 w872 w873 w874 w875 w876 w877 w878 w879 w880 w881]
          frame "Glass Teach" {
          }
          frame "Glass Slide Open", "Express Glass Slide Open" {
            n312 = Bundle By Name(cluster=w851, "Slide Open Data"=w849, "Slide Open Limits"=w848) -> (w850:T54)
          }
          frame "Glass Slide Close", "Express Glass Slide Close" {
            n313 = Bundle By Name(cluster=w855, "Slide Close Data"=w853, "Slide Close Limits"=w852) -> (w854:T54)
          }
          frame "Glass Vent Open", "Express Glass Vent Open" {
            n314 = Bundle By Name(cluster=w859, "Vent Open Data"=w857, "Vent Open Limits"=w856) -> (w858:T54)
          }
          frame "Glass Vent Close", "Express Glass Vent Close" {
            n315 = Bundle By Name(cluster=w863, "Vent Close Data"=w861, "Vent Close Limits"=w860) -> (w862:T54)
          }
          frame "Sunshade Open", "Sunshade Open 2", "Express Sunshade Open" {
            n316 = Bundle By Name(cluster=w867, "Shade Open Data"=w865, "Shade Open Limits"=w864) -> (w866:T54)
          }
          frame "Sunshade Close", "Sunshade Close 2", "Express Sunshade Close" {
            n317 = Bundle By Name(cluster=w871, "Shade Close Data 2"=w869, "Shade Close Limits"=w868) -> (w870:T54)
          }
          frame "Idle", Default {
          }
          frame "Sunshade Teach" {
          }
          frame "Glass Slide Open Sunshade Open" {
          }
          frame "Glass Slide Open Sunshade Close" {
          }
          frame "Glass Slide Close Sunshade Open" {
          }
          frame "Glass Slide Close Sunshade Close" {
          }
          frame "Glass Vent Open Sunshade Open" {
          }
          frame "Glass Vent Open Sunshade Close" {
          }
          frame "Glass Vent Close Sunshade Open" {
          }
          frame "Glass Vent Close Sunshade Close" {
          }
        }
        n318 = property class="Clust (严格)"(reference=w840, error in=w839, "Value"=w837) -> ()  [unwired: 2 out]
      }
      frame "Get Data" {
        # "***temporarily just writing current hall position for both glass and sunshade since we dont track both.\neventually we will have up to 3 motors to track.  probably should just update nvh hmi to display one motion\nat a time and only update 1 single hall position value for the relevant motion/grahpic/glass/rollo1/rollo2"
        n319 = Unbundle By Name(w910) -> ("Decibel data"=w896:dbl[], "rs232 port map.RS232"=w897:refnum<visa-resource-name>, "Motion Status.Analog Data"=w906:sgl[][], "Motion Status.Current Data Index"=w907:i32, "misc status.Part Setup.Communication Type"=w886:T27, "Motion Status.Last Bytes"=w884:u8[], "Motion Status.Current Hall Position"=w911:i16, "Store Data.Motion Data Array"=w902:T11[], "Station Index"=w898:i32, "Store Data.Motion Data Array"=w891:T11[], "Sequence State"=w889:T24, "Motion Status.Motion"=w887:T3)  [unwired: 3 out]
        n320 = Array Size(array=w891) -> (size(s)=w894:i32)
        n321 = Decrement(x=w894) -> (x-1=w893:i32)
        n322 = Index Array(array=w891, index=w893) -> (element=w892:T11)
        n323 = Unbundle By Name(w892) -> ("Motion Data Limits.Check Sound"=w890:bool)
        n324 = call "EOL All-Station Current Buffer.vi"("Check sound?"=w890, "RS232 in"=w897, "Decibel data in"=w896, "station idx"=w898, "Data Index In"=w907, "Data In"=w906) -> ("Decibel data out"=w895:dbl[], "Data Index Out"=w885:i32, "Data Out"=w908:sgl[][])  [unwired: 3 in]
        n325 = Array Size(array=w902) -> (size(s)=w905:i32)
        n326 = Decrement(x=w905) -> (x-1=w901:i32)
        n327 = Index Array(array=w902, index=w901) -> (element=w903:T11)
        n328 = Unbundle By Name(w903) -> ("AP Data"=w904:i16[][])  [unwired: 1 out]
        n329 = call "hold eol seesion decision.vi"("Communication Type"=w886, "Sequence State in"=w889, "Motion Status.Motion"=w887) -> ("Sequence State out"=w888:T24, "Event queue out"=w883:string[])  [unwired: 7 in]
        n330 = Bundle By Name(cluster=w903, "AP Data"=w904) -> (w900:T11)
        n331 = Replace Array Subset(array=w902, new element=w900, index=w901) -> (w899:T11[])
        n332 = Bundle By Name(cluster=w910, "Decibel data"=w895, "Motion Status.Analog Data"=w908, "Motion Status.Current Data Index"=w885, "Motion Status.Last Bytes"=w884, "Store Data.Motion Data Array"=w899, "Motion Status.Current Hall Position"=w911, "Sequence State"=w888) -> (w909:T1)
      }
      frame "Print 2D Barcode" {
        # "pass, and not in bypass to repair mode, and is audit station"
        n333 = Unbundle By Name(w932) -> ("paths.Base Path"=w920:path, "misc status.Plant Number"=w927:u8, "Sequence State.Pass?"=w928:bool, "Store Data.Module Info.Inalfa Part Number"=w931:string, "Store Data.Module Info.Serial Number"=w934:string, "Store Data.Module Info.Sunshade Color"=w933:string, "misc status.Part Setup.Part Type"=w915:string, "misc status.Part History Number"=w930:string, "Store Data.Module Info.Customer Number"=w929:string, "misc station config.is audit station?"=w925:bool, "Sequence State.route-to-repair mode"=w913:bool, "Sequence State.Red-Rabbit Mode"=w914:bool, "misc station config.is print"=w912:bool)
        n334 = call "get path to audit barcode formats.vi"("product"=w915, "paths.Base Path"=w920) -> ("path"=w921:path)  [unwired: 9 in]
        n335 = call <vilib>:"Check if File or Folder Exists.vi"("error in (no error)"=w917, "path"=w921) -> ("error out"=w922:errorcluster, "file or folder exists?"=w924:bool, "dup path"=w923:path)  [unwired: 7 in]
        n336 = Compound Arithmetic op=AND(w928, w925, invert w913, invert w914, w912) -> (w926:bool)
        n337 = case shown="真" w924 {
          tunnel: w923 -> [_ w941]
          tunnel: w922 -> [w937 w940]
          tunnel: [w937 w939] -> w919
          tunnel: [w936 w938] -> w918
          frame False {
            w936 = T62[] []  # Frame Barcode Formats
          }
          frame True {
            n338 = call "read barcode formats.vi"("error in"=w940, "configuration file path"=w941) -> ("error out"=w939:errorcluster, "Frame Barcode Formats"=w938:T62[])  [unwired: 8 in]
          }
        }
        n339 = case shown="真" w926 {
          tunnel: w934 -> [_ w953]
          tunnel: w933 -> [_ w952]
          tunnel: w931 -> [_ w951]
          tunnel: w930 -> [_ w945]
          tunnel: w929 -> [_ w946]
          tunnel: w927 -> [_ w947]
          tunnel: w919 -> [w942 w950]
          tunnel: w918 -> [_ w949]
          tunnel: [w942 w948] -> w916
          tunnel: w915 -> [_ w943]
          frame False {
          }
          frame True {
            n340 = call "Barcode Print.vi"("part type"=w943, "Manual?"=FALSE, "error in"=w950, "Part History Number"=w945, "Plant Number"=w947, "Customer Number"=w946, "Color"=w952, "Serial Number"=w953, "Inalfa Part Number"=w951, "Frame Barcode Formats"=w949) -> ("error out"=w948:errorcluster)  [unwired: 1 in]
          }
        }
      }
      frame "Read Barcode" {
        n341 = Unbundle By Name(w988) -> ("ctl refs.all station status"=w976:refnum<vi>, "paths.Base Path"=w970:path, "Config Info"=w956:T34)
        n342 = call "Config Info Get.vi"("Config Info"=w956) -> ("PLC Comms"=w955:T56)  [unwired: 7 in, 3 out]
        n343 = Unbundle By Name(w955) -> ("PLC string read Tags"=w954:T59)
        n344 = call "WKLXF25 Get Part Information 3.0.vi"("error in"=w987, "PLC Tags"=w954) -> ("error out"=w986:errorcluster, "part info"=w985:T64)  [unwired: 7 in, 1 out]
        n345 = Unbundle By Name(w985) -> ("Serial Number"=w972:string, "Pallet Number"=w974:string, "Inalfa Part Number"=w981:string, "Part Type"=w973:string, "Shade Color"=w982:string, "Customer Number"=w983:string, "Part History Number"=w984:string, "Sunshade Barcode 2"=w964:string, "Sunshade Barcode 1"=w965:string)
        n346 = Build Path(base path=w970, name or relative path="System\\Part Configuration\\Sunshade Color.txt") -> (appended path=w969:path)
        n347 = property class="Clust (严格)"(reference=w976) -> (reference out=w980:refnum<vi>, error out=w977:errorcluster, "Value"=w978:T52)  [unwired: 1 in]
        n348 = Format Into String(error in=w986, w973) -> (resulting string=w975:string, error out=w958:errorcluster)  [unwired: 2 in]
        n349 = call <vilib>:"Check if File or Folder Exists.vi"("error in (no error)"=w958, "path"=w969) -> ("error out"=w959:errorcluster, "file or folder exists?"=w967:bool, "dup path"=w968:path)  [unwired: 7 in]
        n350 = case shown="真" w967 {
          tunnel: w968 -> [_ w1005]
          tunnel: [_ w1003] -> w966
          tunnel: w959 -> [w1000 w1002]
          tunnel: [w1000 w1001] -> w957
          frame False {
          }
          frame True {
            n351 = call <vilib>:"Read Characters From File.vi"("file path (dialog if empty)"=w1005) -> ("character string"=w1004:string)  [unwired: 5 in, 3 out]
            n352 = Unflatten From String(type=T46[] [] ("Array"), binary string=w1004, error in (no error)=w1002) -> (value=w1003:T46[], error out=w1001:errorcluster)  [unwired: 2 in, 1 out]
          }
        }
        n353 = Bundle By Name(cluster=w978, "Part Type"=w975, "Pallet Number"=w974, "Sunroof Barcode"=w972) -> (w979:T52)
        n354 = for {
          tunnel: w966 -> [w999] mode=indexing
          tunnel: w965 -> [w998]
          tunnel: w964 -> [w997]
          tunnel: [w992] -> w963
          tunnel: [w991] -> w962
          stop <- w992 stop-if-true
          n355 = Unbundle By Name(w999) -> ("Sunshade 1 Number"=w996:string, "Sunshade 2 Number"=w995:string, "keyence tuning bank param idx"=w991:i32)
          n356 = Equal?(x=w998, y=w996) -> (x = y?=w993:bool)
          n357 = Equal?(x=w997, y=w995) -> (x = y?=w994:bool)
          n358 = And(x=w993, y=w994) -> (x .and. y?=w992:bool)
        }
        n359 = Select(t=w962, s=w963, f=0) -> (s? t:f=w961:i32)
        n360 = property class="Clust (严格)"(reference=w980, error in=w977, "Value"=w979) -> ()  [unwired: 2 out]
        n361 = Bundle By Name(cluster=w988, "misc status.Part History Number"=w984, "Store Data.Module Info.Customer Number"=w983, "misc status.Part Setup.Part Type"=w973, "Store Data.Module Info.Pallet Number"=w974, "Store Data.Module Info.Serial Number"=w972, "Store Data.Module Info.Sunshade Color"=w982, "Store Data.Module Info.Inalfa Part Number"=w981, "Sunshade Barcode Scan.Sunshade Number 1"=w965, "Sunshade Barcode Scan.Sunshade Number 2"=w964, "Sunshade Barcode Scan.Keyence tuning bank idx"=w961) -> (w990:T1)
      }
      frame "Set Power Supply" {
        n362 = Unbundle By Name(w1027) -> ("misc station config.power supply type"=w1020:T20, "Sequence State"=w1017:T24, "rs232 port map.PS Port"=w1026:refnum<visa-resource-name>, "misc status.PS Voltage"=w1025:dbl, "Store Data.Error Table"=w1024:string[][], "misc station config.Station Name"=w1022:string, "Station Index"=w1021:i32, "misc status.Part Setup.Motor Type"=w1019:T30, "Store Data.Motion Data Array"=w1010:T11[])
        n363 = case shown="\"Smart Motor\", 默认" w1019 {
          tunnel: [T47."Motor Voltage" EOL_Analog_Input_Control."SW PS  Volage" ("Analog Control")] -> w1023
          frame "Smart Motor", Default {
          }
          frame "Sensor Motor" {
          }
        }
        n364 = call "EOL Set Power Supply Voltage.vi"("PS Channel Control"=w1023, "station name"=w1022, "power supply type"=w1020, "Error Table In"=w1024, "station idx"=w1021, "Power Supply Voltage"=w1025, "Power Supply Comm Port"=w1026) -> ("Error Table Out"=w1029:string[][], "Actual Voltage"=w1009:dbl, "Pass?"=w1007:bool)  [unwired: 2 in]
        n365 = Array Size(array=w1010) -> (size(s)=w1014:i32)
        n366 = Decrement(x=w1014) -> (x-1=w1013:i32)
        n367 = call "pass fail action decision.vi"("Pass?"=w1007, "Sequence State in"=w1017, "event queue in"=w1018) -> ("Sequence State out"=w1016:T24, "Event queue out"=w1015:string[])  [unwired: 7 in]
        n368 = Index Array(array=w1010, index=w1013) -> (element=w1012:T11)
        n369 = Bundle By Name(cluster=w1012, "Actual PS Voltage"=w1009) -> (w1011:T11)
        n370 = Replace Array Subset(array=w1010, new element=w1011, index=w1013) -> (w1008:T11[])
        n371 = Bundle By Name(cluster=w1027, "Sequence State"=w1016, "Store Data.Motion Data Array"=w1008, "Store Data.Error Table"=w1029) -> (w1028:T1)
      }
      frame "Send LIN Message for inalfa SCU" {
        n372 = Unbundle By Name(w1038) -> ("LIN INFO.NAD"=w1032:u8, "LIN INFO.Toolkit Type"=w1035:enum16{"Inalfa LIN", "ADCS LIN", "TS LIN"}, "misc status.Part Setup.Part Type"=w1047:string, "Sequence State"=w1057:T24, "LIN INFO.Inalfa LIN"=w1056:T32, "Store Data.data bytes log"=w1055:string, "Sequence State.Step Description"=w1036:string, "Sequence State.Step Data String"=w1054:string, "LIN INFO.ADCS LIN"=w1034:T33, "LIN INFO.TS LIN"=w1033:T65, "Store Data.Error Table"=w1060:string[][], "Motion Status.Motion"=w1049:T3, "misc status.Part Setup.Communication Type"=w1048:T27, "ctl refs.Individual Station Status"=w1037:refnum<vi>)
        n373 = case shown="\"Inalfa LIN\", 默认" w1035 {
          tunnel: w1057 -> [w1076 w1090 w1105]
          tunnel: w1056 -> [w1075 _ _]
          tunnel: w1055 -> [w1074 w1089 w1104]
          tunnel: w1054 -> [w1073 w1087 w1103]
          tunnel: [w1072 w1085 w1101] -> w1053
          tunnel: [w1071 w1082 w1098] -> w1052
          tunnel: [w1070 w1083 w1099] -> w1051
          tunnel: [w1069 w1081 w1097] -> w1050
          tunnel: w1047 -> [w1068 w1086 w1102]
          tunnel: [w1067 w1079 w1095] -> w1046
          tunnel: [w1066 w1078 w1094] -> w1045
          tunnel: [w1065 w1084 w1100] -> w1044
          tunnel: [w1064 w1077 w1092] -> w1043
          tunnel: [w1063 w1080 w1096] -> w1040
          tunnel: w1036 -> [w1062 w1091 w1106]
          tunnel: w1034 -> [_ w1088 _]
          tunnel: w1033 -> [_ _ w1093]
          tunnel: w1032 -> [w1061 _ _]
          frame "Inalfa LIN", Default {
            n374 = call "Inalfa SCU_LIN Message.vi"("Sequence State in"=w1076, "LIN Device"=w1075, "data bytes log in"=w1074, "Sequence State.Step Description"=w1062, "Sequence State.Step Data String"=w1073, "Mode type"=w1068, "NAD"=w1061) -> ("Software version"=w1066:string[], "Calfile version"=w1064:string[], "Hardware version"=w1067:string[], "data bytes log out"=w1063:string, "Response Good?"=w1070:bool, "Error Description"=w1071:string, "version type"=w1065:T66, "Sequence State out"=w1069:T24, "Error No."=w1072:u16)  [unwired: 3 in, 1 out]
          }
          frame "ADCS LIN" {
            n375 = call <vilib>:"Inalfa ADCS LIN.vi"("seq in"=w1091, "Sequence State.Step Data String"=w1087, "ADCS_LIN info"=w1088, "Mode type"=w1086, "LINbyteLog"=w1089, "Sequence State in"=w1090) -> ("Software version"=w1078:string[], "Sequence State out"=w1081:T67, "Cal file version"=w1077:string[], "Hardware version"=w1079:string[], "error description"=w1082:string, "pass?"=w1083:bool, "version type"=w1084:T66, "error code"=w1085:u16, "LIN.LINbyteLog"=w1080:string)  [unwired: 3 in, 2 out]
          }
          frame "TS LIN" {
            n376 = call <vilib>:"Inalfa TS LIN.vi"("seq in"=w1106, "Sequence State.Step Data String"=w1103, "Ts_LIN info"=w1093, "Mode type"=w1102, "LINbyteLog"=w1104, "Sequence State in"=w1105) -> ("Software version"=w1094:string[], "Sequence State out"=w1097:T67, "Cal file version"=w1092:string[], "Hardware version"=w1095:string[], "Error Description"=w1098:string, "pass?"=w1099:bool, "version type"=w1100:T66, "error code"=w1101:u16, "LIN.LINbyteLog"=w1096:string)  [unwired: 3 in, 2 out]
          }
        }
        n377 = case shown="假" w1051 {
          tunnel: w1060 -> [w1155 w1156]
          tunnel: [w1154 w1156] -> w1042
          tunnel: w1053 -> [w1153 _]
          tunnel: w1052 -> [w1152 _]
          frame False {
            n378 = call "EOL Error Table.vi"("Error Description"=w1152, "Error No."=w1153, "Error Table In"=w1155) -> ("Error Table Out"=w1154:string[][])  [unwired: 7 in, 1 out]
          }
          frame True {
          }
        }
        n379 = call "pass fail action decision.vi"("Communication Type"=w1048, "Motion"=w1049, "Pass?"=w1051, "Sequence State in"=w1050, "event queue in"=w1059) -> ("Sequence State out"=w1041:T24, "Event queue out"=w1058:string[])  [unwired: 5 in]
        n380 = case shown="\"Hardware version\"" w1044 {
          tunnel: w1046 -> [_ _ w1138 _]
          tunnel: w1045 -> [_ w1117 _ _]
          tunnel: w1043 -> [_ _ _ w1151]
          tunnel: w1042 -> [w1109 w1114 w1143 w1150]
          tunnel: w1041 -> [w1111 w1116 w1145 w1147]
          tunnel: w1040 -> [w1110 w1115 w1144 w1146]
          tunnel: [w1108 w1112 w1142 w1149] -> w1039
          tunnel: w1038 -> [w1107 w1113 w1141 w1148]
          tunnel: w1037 -> [_ _ w1140 _]
          frame "NO read", Default {
            n381 = Bundle By Name(cluster=w1107, "Sequence State"=w1111, "Store Data.data bytes log"=w1110, "Store Data.Error Table"=w1109) -> (w1108:T1)
          }
          frame "Softeware version" {
            n382 = Bundle By Name(cluster=w1113, "Store Data.Software Version"=w1117, "Sequence State"=w1116, "Store Data.data bytes log"=w1115, "Store Data.Error Table"=w1114) -> (w1112:T1)
          }
          frame "Hardware version" {
            n383 = property class="Clust (严格)"(reference=w1140) -> (reference out=w1137:refnum<vi>, error out=w1135:errorcluster, "Value"=w1139:T51)  [unwired: 1 in]
            n384 = Index Array(array=w1138) -> (element #1=w1128:string, element #2=w1121:string)  [unwired: 2 in]
            n385 = Scan From String(format string="%x" ("格式字符串"), input string=w1121, default 1=u16 0) -> (output 1=w1126:u16)  [unwired: 2 in, 3 out]
            n386 = Scan From String(format string="%x" ("格式字符串"), input string=w1128, default 1=u16 0) -> (output 1=w1133:u16)  [unwired: 2 in, 3 out]
            n387 = Split Number(x=w1126) -> (hi(x)=w1125:u8, lo(x)=w1124:u8)
            n388 = Split Number(x=w1133) -> (hi(x)=w1132:u8, lo(x)=w1131:u8)
            n389 = Build Array(w1125, w1124) -> (w1123:u8[])
            n390 = Build Array(w1132, w1131) -> (w1130:u8[])
            n391 = Byte Array To String(unsigned byte array=w1123) -> (string=w1119:string)
            n392 = Byte Array To String(unsigned byte array=w1130) -> (string=w1120:string)
            n393 = Bundle By Name(cluster=w1139, "Hardware Ver"=w1120) -> (w1136:T51)
            n394 = property class="Clust (严格)"(reference=w1137, error in=w1135, "Value"=w1136) -> ()  [unwired: 2 out]
            n395 = Build Array(w1120, w1119) -> (w1118:string[])
            n396 = Bundle By Name(cluster=w1141, "Store Data.Hardware Version"=w1118, "Sequence State"=w1145, "Store Data.data bytes log"=w1144, "Store Data.Error Table"=w1143) -> (w1142:T1)
          }
          frame "Calfile version" {
            n397 = Bundle By Name(cluster=w1148, "Store Data.Constant Version"=w1151, "Sequence State"=w1147, "Store Data.data bytes log"=w1146, "Store Data.Error Table"=w1150) -> (w1149:T1)
          }
        }
      }
      frame "Send LIN Uncond Frame" {
        w1159 = TRUE
        n398 = Unbundle By Name(w1169) -> ("Store Data.data bytes log"=w1157:string, "LIN INFO.Toolkit Type"=w1168:enum16{"Inalfa LIN", "ADCS LIN", "TS LIN"}, "Sequence State"=w1160:T24, "LIN INFO.Inalfa LIN"=w1167:T32, "Sequence State.Step Data String"=w1164:string, "LIN INFO.TS LIN"=w1166:T65, "Store Data.Error Table"=w1176:string[][], "LIN INFO.ADCS LIN"=w1158:T33, "Motion Status.Motion"=w1163:T3, "misc status.Part Setup.Communication Type"=w1173:T27)
        n399 = call "Expr_Send LIN Uncond Frame.vi"("Toolkit Type"=w1168, "data string"=w1164, "byte log"=w1157, "Inalfa LIN"=w1167, "TS LIN"=w1166, "ADCS LIN"=w1158, "error in"=w1165, "Current Motion"=w1163) -> ("byte log"=w1162:string, "error out"=w1161:errorcluster)  [unwired: 6 in]
        n400 = case shown="假" w1159 {
          tunnel: w1176 -> [w1179 w1180]
          tunnel: [w1178 w1180] -> w1172
          frame False {
            n401 = call "EOL Error Table.vi"("Error No."=u16 132, "Error Table In"=w1179) -> ("Error Table Out"=w1178:string[][])  [unwired: 8 in, 1 out]
          }
          frame True {
          }
        }
        n402 = call "pass fail action decision.vi"("Communication Type"=w1173, "Motion"=w1163, "Pass?"=w1159, "Sequence State in"=w1160, "event queue in"=w1175) -> ("Sequence State out"=w1171:T24, "Event queue out"=w1174:string[])  [unwired: 5 in]
        n403 = Bundle By Name(cluster=w1169, "Sequence State"=w1171, "Store Data.data bytes log"=w1162, "Store Data.Error Table"=w1172) -> (w1170:T1)
      }
      frame "Save Data" {
        n404 = Unbundle By Name(w1188) -> ("Sequence State.Red-Rabbit Mode"=w1192:bool, "Sequence State.route-to-repair mode"=w1191:bool, "Sequence State"=w1189:T24, "Store Data.Module Info.Serial Number"=w1195:string, "misc station config.is audit station?"=w1194:bool, "ctl refs.all station status"=w1184:refnum<vi>)
        n405 = property class="Clust (严格)"(reference=w1184) -> ("Controls[]"=w1185:refnum<vi>[])  [unwired: 1 in, 2 out]
        n406 = Unbundle By Name(w1189) -> ("Pass?"=w1190:bool)
        n407 = Index Array(array=w1185, index=6 ("索引")) -> (element=w1182:refnum<vi>)
        n408 = Compound Arithmetic op=AND(w1194, invert w1192, invert w1191) -> (w1193:bool)
        n409 = property class="Ctl"(reference=w1182, "Value"="Sequence Completed and Save Data") -> ()  [unwired: 1 in, 2 out]
        n410 = disable-structure shown="禁用" {
          disable-tunnel: w1195 -> [w1199 _]
          disable-tunnel: w1193 -> [w1198 _]
          disable-tunnel: w1190 -> [w1197 _]
          frame Disabled {
            n411 = case shown="真" w1198 {
              tunnel: w1197 -> [_ w1201]
              tunnel: w1199 -> [_ w1200]
              frame False {
              }
              frame True {
                n412 = call "Cockpit Data Loging ver5.vi"("Serial Number"=w1200, "Pass/Fail"=w1201) -> ()  [unwired: 10 in]
              }
            }
          }
          frame Enabled {
          }
        }
        n413 = call "EOL Save Module Test Data v2.6.vi"("error in"=w1187, "main state cluster"=w1188) -> ("error out"=w1186:errorcluster)  [unwired: 9 in]
      }
      frame "Exit" {
        n414 = Unbundle By Name(w1214) -> ("ctl refs.Individual Station Status"=w1209:refnum<vi>, "ethernet tcp refs"=w1207:cluster{"LVDT Unit":refnum<k5>}, "rs232 port map.RS232"=w1204:refnum<visa-resource-name>, "LIN INFO.Toolkit Type"=w1203:enum16{"Inalfa LIN", "ADCS LIN", "TS LIN"}, "LIN INFO.TS LIN.ref info"=w1202:refnum<k24>)
        n415 = Cluster To Array(cluster=w1207) -> (array=w1206:refnum<k5>[])
        n416 = case shown="\"TS LIN\"" w1203 {
          tunnel: w1202 -> [_ _ w1217]
          frame "Inalfa LIN", Default {
          }
          frame "ADCS LIN" {
          }
          frame "TS LIN" {
            n417 = call <vilib>:"Ts_Ref_Close.vi"("TsRef in"=w1217) -> ("错误输出"=w1216:errorcluster)  [unwired: 10 in]
            n418 = call <vilib>:"Clear Errors.vi"("error in (no error)"=w1216) -> ()  [unwired: 5 in, 2 out]
          }
        }
        n419 = property class="Clust (严格)"(reference=w1209) -> (reference out=w1213:refnum<vi>, error out=w1210:errorcluster, "Value"=w1211:T51)  [unwired: 1 in]
        n420 = for {
          tunnel: w1206 -> [w1220] mode=indexing
          n421 = Not Equal?(x=w1220, y=refnum<k5> refnum) -> (x != y?=w1221:bool)
          n422 = case shown="真" w1221 {
            tunnel: w1220 -> [_ w1224]
            frame False {
            }
            frame True {
              n423 = TCP Close Connection(connection ID=w1224) -> (error out=w1223:errorcluster)  [unwired: 2 in, 1 out]
              n424 = call <vilib>:"Clear Errors.vi"("error in (no error)"=w1223) -> ()  [unwired: 5 in, 2 out]
            }
          }
        }
        n425 = Empty String/Path?(string/path=w1204) -> (empty?=w1205:bool)
        n426 = Bundle By Name(cluster=w1211, "Loop Stopped?"=TRUE ("Boolean")) -> (w1212:T51)
        n427 = case shown="假" w1205 {
          tunnel: w1204 -> [w1219 _]
          frame False {
            n428 = VISA Close(VISA resource name=w1219) -> (error out=w1218:errorcluster)  [unwired: 1 in]
            n429 = call <vilib>:"Clear Errors.vi"("error in (no error)"=w1218) -> ()  [unwired: 5 in, 2 out]
          }
          frame True {
          }
        }
        n430 = property class="Clust (严格)"(reference=w1213, error in=w1210, "Value"=w1212) -> ()  [unwired: 2 out]
      }
      frame "--------ATS--------" {
      }
      frame "AT Check Data Glass" {
        w1228 = 75.0 ("new element/subarray")
        n431 = Unbundle By Name(w1261) -> ("ctl refs.Individual Station Status"=w1249:refnum<vi>, "AP Test Data.Database AP Data"=w1269:dbl[], "AP Test Data.Raw Glass AP Data"=w1256:string, "AP Test Data.Raw Sunshade AP Data"=w1255:string, "Store Data.Error Table"=w1258:string[][], "rs232 port map.PMAC"=w1241:refnum<visa-resource-name>, "AP Test Data.PMAC Read Counter"=w1262:dbl, "Sequence State.Step Data String"=w1263:string, "Sequence State"=w1247:T24)  [unwired: 1 out]
        n432 = Unflatten From String(type=T48 {"Power Supply Voltage"=10.0, "Glass  Max Reversal Force"=10.0, "Rollo Max Reversal Force"=10.0, "Rollo02 Max Reversal Force"=10.0, "Vent Max Reversal Force"=0.0} ("Anti Pinch Test Data Control"), binary string=w1263, error in (no error)=w1254) -> (value=w1264:T48, error out=w1259:errorcluster)  [unwired: 2 in, 1 out]
        n433 = Unbundle By Name(w1264) -> ("Power Supply Voltage"=w1266:dbl, "Glass  Max Reversal Force"=w1273:dbl, "Rollo Max Reversal Force"=w1267:dbl, "Rollo02 Max Reversal Force"=w1238:dbl, "Vent Max Reversal Force"=w1233:dbl)
        n434 = call "EOL PMAC Clear Read History.vi"("Sys Error In"=w1259, "PMAC Read History Counter"=w1262, "Prerun PMAC"=w1241) -> ("Sys Error Out"=w1231:errorcluster)  [unwired: 8 in]
        n435 = Replace Array Subset(array=w1269, new element=w1266, index=0) -> (w1271:dbl[])
        n436 = Replace Array Subset(array=w1271, new element=w1273, index=2) -> (w1272:dbl[])
        n437 = property class="Clust (严格)"(reference=w1249) -> (reference out=w1252:refnum<vi>, error out=w1248:errorcluster, "Value"=w1250:T51)  [unwired: 1 in]
        n438 = Replace Array Subset(array=w1272, new element=w1267, index=4) -> (w1239:dbl[])
        n439 = Replace Array Subset(array=w1239, new element=w1238, index=6) -> (w1235:dbl[])
        n440 = Replace Array Subset(array=w1235, new element=w1233, index=8) -> (w1232:dbl[])
        n441 = Replace Array Subset(array=w1232, new element #1=w1228, index #1=5 ("index"), new element #2=w1228, index #2=7) -> (w1237:dbl[])
        n442 = call "EOL AP Check Data.vi"("Raw Rollo AP Data"=w1255, "Raw Glass AP Data"=w1256, "error in"=w1231, "Error Table"=w1258, "Database AP Data"=w1237) -> ("error out"=w1253:errorcluster, "Error Table Out"=w1257:string[][], "Pass? Out"=w1244:bool)  [unwired: 4 in]
        n443 = Bundle By Name(cluster=w1250, "Anti Pinch Test?"=w1244) -> (w1251:T51)
        n444 = call "pass fail action decision.vi"("fail behavior"=failure_behaviors."stop at next 'check sequence' if not rabbit", "Pass?"=w1244, "Sequence State in"=w1247, "event queue in"=w1245) -> ("Sequence State out"=w1243:T24, "Event queue out"=w1246:string[])  [unwired: 6 in]
        n445 = Bundle By Name(cluster=w1261, "Store Data.Error Table"=w1257, "Store Data.Anti Pinch Force"=w1237, "Sequence State"=w1243, "AP Test Data.Database AP Data"=w1232) -> (w1260:T1)
        n446 = property class="Clust (严格)"(reference=w1252, error in=w1248, "Value"=w1251) -> ()  [unwired: 2 out]
      }
      frame "AT Check Data" {
        n447 = Unbundle By Name(w1306) -> ("ctl refs.Individual Station Status"=w1294:refnum<vi>, "AP Test Data.Database AP Data"=w1314:dbl[], "AP Test Data.Raw Glass AP Data"=w1301:string, "AP Test Data.Raw Sunshade AP Data"=w1300:string, "Store Data.Error Table"=w1303:string[][], "rs232 port map.PMAC"=w1286:refnum<visa-resource-name>, "AP Test Data.PMAC Read Counter"=w1307:dbl, "Sequence State.Step Data String"=w1308:string, "Sequence State"=w1292:T24)  [unwired: 1 out]
        n448 = Unflatten From String(type=T48 {"Power Supply Voltage"=10.0, "Glass  Max Reversal Force"=10.0, "Rollo Max Reversal Force"=10.0, "Rollo02 Max Reversal Force"=10.0, "Vent Max Reversal Force"=0.0} ("Anti Pinch Test Data Control"), binary string=w1308, error in (no error)=w1299) -> (value=w1309:T48, error out=w1304:errorcluster)  [unwired: 2 in, 1 out]
        n449 = Unbundle By Name(w1309) -> ("Power Supply Voltage"=w1311:dbl, "Glass  Max Reversal Force"=w1318:dbl, "Rollo Max Reversal Force"=w1312:dbl, "Rollo02 Max Reversal Force"=w1283:dbl, "Vent Max Reversal Force"=w1277:dbl)
        n450 = call "EOL PMAC Clear Read History.vi"("Sys Error In"=w1304, "PMAC Read History Counter"=w1307, "Prerun PMAC"=w1286) -> ("Sys Error Out"=w1276:errorcluster)  [unwired: 8 in]
        n451 = Replace Array Subset(array=w1314, new element=w1311, index=0) -> (w1316:dbl[])
        n452 = Replace Array Subset(array=w1316, new element=w1318, index=2) -> (w1317:dbl[])
        n453 = property class="Clust (严格)"(reference=w1294) -> (reference out=w1297:refnum<vi>, error out=w1293:errorcluster, "Value"=w1295:T51)  [unwired: 1 in]
        n454 = Replace Array Subset(array=w1317, new element=w1312, index=4) -> (w1284:dbl[])
        n455 = Replace Array Subset(array=w1284, new element=w1283, index=6) -> (w1280:dbl[])
        n456 = Replace Array Subset(array=w1280, new element=w1277, index=8) -> (w1279:dbl[])
        n457 = Replace Array Subset(array=w1279, new element=75.0 ("new element/subarray"), index=5) -> (w1282:dbl[])
        n458 = call "EOL AP Check Data.vi"("Raw Rollo AP Data"=w1300, "Raw Glass AP Data"=w1301, "error in"=w1276, "Error Table"=w1303, "Database AP Data"=w1282) -> ("error out"=w1298:errorcluster, "Error Table Out"=w1302:string[][], "Pass? Out"=w1289:bool)  [unwired: 4 in]
        n459 = Bundle By Name(cluster=w1295, "Anti Pinch Test?"=w1289) -> (w1296:T51)
        n460 = call "pass fail action decision.vi"("fail behavior"=failure_behaviors."stop at next 'check sequence' if not rabbit", "Pass?"=w1289, "Sequence State in"=w1292, "event queue in"=w1290) -> ("Sequence State out"=w1288:T24, "Event queue out"=w1291:string[])  [unwired: 6 in]
        n461 = Bundle By Name(cluster=w1306, "Store Data.Error Table"=w1302, "Store Data.Anti Pinch Force"=w1282, "Sequence State"=w1288) -> (w1305:T1)
        n462 = property class="Clust (严格)"(reference=w1297, error in=w1293, "Value"=w1296) -> ()  [unwired: 2 out]
      }
      frame "AT Check Glass Position", "AT Check Sunshade Position", "Check LVDT's Retracted", "Check Windproof position" {
        n463 = Unbundle By Name(w1329) -> ("Store Data.Error Table"=w1338:string[][], "D in map.Abort Test"=w1333:T17, "Sequence State"=w1327:T24, "Config Info"=w1320:T34)
        n464 = call "Config Info Get.vi"("Config Info"=w1320) -> ("PLC Comms"=w1319:T56)  [unwired: 7 in, 3 out]
        n465 = case shown="\"AT Check Glass Position\", 默认" w1332 {
          tunnel: [w1341 w1346 w1349 w1354] -> w1331
          tunnel: [" - Rollo Open" ("Error Description") _ _ " - Glass Open" ("Error Description")] -> w1330
          tunnel: w1319 -> [w1342 w1347 w1351 w1355]
          tunnel: [u16 21 ("Error No.") u16 21 ("Error No.") u16 44 ("Error No.") u16 21 ("Error No.")] -> w1328
          tunnel: [failure_behaviors."stop immediately" ("fail behavior") failure_behaviors."stop immediately" ("fail behavior") failure_behaviors."stop immediately" ("fail behavior") failure_behaviors."stop immediately" ("fail behavior")] -> w1325
          frame "AT Check Sunshade Position" {
            n466 = Unbundle By Name(w1342) -> ("PLC boolean read Tags.AT shade position"=w1341:T40)
          }
          frame "Check Windproof position" {
            n467 = Unbundle By Name(w1347) -> ("PLC boolean read Tags.windproof position"=w1346:T40)
          }
          frame "Check LVDT's Retracted" {
            n468 = Unbundle By Name(w1351) -> ("PLC boolean read Tags.LVDT's Extended"=w1349:T40)
          }
          frame "AT Check Glass Position", Default {
            n469 = Unbundle By Name(w1355) -> ("PLC boolean read Tags.AT glass position"=w1354:T40)
          }
        }
        n470 = call "wait for plc bit.vi"("error in"=w1335, "tag"=w1331, "Abort Test"=w1333) -> ("error out"=w1334:errorcluster, "final values"=w1322:bool)  [unwired: 7 in]
        n471 = call "pass fail action decision.vi"("fail behavior"=w1325, "Pass?"=w1322, "Sequence State in"=w1327, "event queue in"=w1324) -> ("Sequence State out"=w1326:T24, "Event queue out"=w1323:string[])  [unwired: 6 in]
        n472 = case shown="假" w1322 {
          tunnel: w1338 -> [w1362 w1364]
          tunnel: [w1361 w1364] -> w1337
          tunnel: w1334 -> [w1360 w1363]
          tunnel: [w1359 w1363] -> w1321
          tunnel: w1330 -> [w1358 _]
          tunnel: w1328 -> [w1357 _]
          frame False {
            n473 = call "EOL Error Table.vi"("Error Description"=w1358, "error in"=w1360, "Error No."=w1357, "Error Table In"=w1362) -> ("error out"=w1359:errorcluster, "Error Table Out"=w1361:string[][])  [unwired: 6 in]
          }
          frame True {
          }
        }
        n474 = Bundle By Name(cluster=w1329, "Store Data.Error Table"=w1337, "Sequence State"=w1326) -> (w1336:T1)
      }
      frame "AT Check PAMC3000 Data" {
        w1366 = 75.0 ("new element/subarray")
        n475 = Unbundle By Name(w1395) -> ("ctl refs.Individual Station Status"=w1384:refnum<vi>, "AP Test Data.Database AP Data"=w1403:dbl[], "AP Test Data.Raw Glass AP Data"=w1391:string, "AP Test Data.Raw Sunshade AP Data"=w1390:string, "Store Data.Error Table"=w1393:string[][], "Sequence State.Step Data String"=w1396:string, "Sequence State"=w1382:T24)  [unwired: 3 out]
        n476 = Unflatten From String(type=T48 {"Power Supply Voltage"=10.0, "Glass  Max Reversal Force"=10.0, "Rollo Max Reversal Force"=10.0, "Rollo02 Max Reversal Force"=10.0, "Vent Max Reversal Force"=0.0} ("Anti Pinch Test Data Control"), binary string=w1396, error in (no error)=w1389) -> (value=w1398:T48, error out=w1372:errorcluster)  [unwired: 2 in, 1 out]
        n477 = Unbundle By Name(w1398) -> ("Power Supply Voltage"=w1400:dbl, "Glass  Max Reversal Force"=w1407:dbl, "Rollo Max Reversal Force"=w1401:dbl, "Rollo02 Max Reversal Force"=w1374:dbl, "Vent Max Reversal Force"=w1368:dbl)
        n478 = Replace Array Subset(array=w1403, new element=w1400, index=0) -> (w1405:dbl[])
        n479 = Replace Array Subset(array=w1405, new element=w1407, index=2) -> (w1406:dbl[])
        n480 = property class="Clust (严格)"(reference=w1384) -> (reference out=w1387:refnum<vi>, error out=w1383:errorcluster, "Value"=w1385:T51)  [unwired: 1 in]
        n481 = Replace Array Subset(array=w1406, new element=w1401, index=4) -> (w1375:dbl[])
        n482 = Replace Array Subset(array=w1375, new element=w1374, index=6) -> (w1371:dbl[])
        n483 = Replace Array Subset(array=w1371, new element=w1368, index=8) -> (w1370:dbl[])
        n484 = Replace Array Subset(array=w1370, new element #1=w1366, index #1=5 ("index"), new element #2=w1366, index #2=7 ("index")) -> (w1373:dbl[])
        n485 = call "EOL AP Check Data.vi"("Raw Rollo AP Data"=w1390, "Raw Glass AP Data"=w1391, "error in"=w1372, "Error Table"=w1393, "Database AP Data"=w1373) -> ("error out"=w1388:errorcluster, "Error Table Out"=w1392:string[][], "Pass? Out"=w1379:bool)  [unwired: 4 in]
        n486 = Bundle By Name(cluster=w1385, "Anti Pinch Test?"=w1379) -> (w1386:T51)
        n487 = call "pass fail action decision.vi"("fail behavior"=failure_behaviors."stop at next 'check sequence' if not rabbit", "Pass?"=w1379, "Sequence State in"=w1382, "event queue in"=w1380) -> ("Sequence State out"=w1378:T24, "Event queue out"=w1381:string[])  [unwired: 6 in]
        n488 = Bundle By Name(cluster=w1395, "Store Data.Error Table"=w1392, "Store Data.Anti Pinch Force"=w1373, "Sequence State"=w1378) -> (w1394:T1)
        n489 = property class="Clust (严格)"(reference=w1387, error in=w1383, "Value"=w1386) -> ()  [unwired: 2 out]
      }
      frame "AT Clear PMAC Data" {
        n490 = Unbundle By Name(w1410) -> ("rs232 port map.PMAC"=w1412:refnum<visa-resource-name>)
        n491 = while {
          tunnel: w1412 -> [w1419]
          shift-right: [w1415] -> w1408
          shift-left: w1409 -> [w1417]
          stop <- w1413 stop-if-true
          n492 = property class="Instr"(reference=w1419, error in=w1417) -> (reference out=w1418:refnum<visa-resource-name>, error out=w1416:errorcluster, "Serial Settings:Number of Bytes at Serial Port"=w1414:u32)
          n493 = Less Or Equal To 0?(x=w1414) -> (x <= 0?=w1413:bool)
          n494 = case shown="假" w1413 {
            tunnel: w1418 -> [w1423 _]
            tunnel: w1416 -> [w1422 w1424]
            tunnel: [w1421 w1424] -> w1415
            tunnel: w1414 -> [w1420 _]
            frame False {
              n495 = VISA Read(VISA resource name=w1423, byte count=w1420, error in (no error)=w1422) -> (error out=w1421:errorcluster)  [unwired: 3 out]
            }
            frame True {
            }
          }
        }
      }
      frame "AT Get PMAC Data Glass", "AT Get PMAC Data Sunshade" {
        n496 = Unbundle By Name(w1433) -> ("AP Test Data.Database AP Data"=w1447:dbl[], "rs232 port map.PMAC"=w1446:refnum<visa-resource-name>, "AP Test Data.PMAC Read Counter"=w1435:dbl)
        n497 = property class="Instr"(reference=w1446, error in=w1430) -> (reference out=w1444:refnum<visa-resource-name>, error out=w1429:errorcluster, "Serial Settings:Number of Bytes at Serial Port"=w1445:u32)
        n498 = case shown="\"AT Get PMAC Data Glass\", 默认" w1426 {
          tunnel: [1 ("index") 3 ("index")] -> w1425
          frame "AT Get PMAC Data Glass", Default {
          }
          frame "AT Get PMAC Data Sunshade" {
          }
        }
        n499 = VISA Read(VISA resource name=w1444, byte count=w1445, error in (no error)=w1429) -> (read buffer=w1434:string, error out=w1428:errorcluster)  [unwired: 2 out]
        n500 = String Subset(string=w1434, offset (0)=8) -> (substring=w1442:string)  [unwired: 1 in]
        n501 = Match Pattern(string=w1442, regular expression=" ") -> (before substring=w1440:string)  [unwired: 1 in, 3 out]
        n502 = Empty String/Path?(string/path=w1440) -> (empty?=w1439:bool)
        n503 = case shown="假" w1439 {
          tunnel: w1440 -> [w1463 _]
          tunnel: [w1461 0.0 ("default value 1")] -> w1448
          tunnel: [w1452 w1464] -> w1427
          tunnel: [w1456 w1465] -> w1436
          tunnel: w1435 -> [_ w1465]
          tunnel: w1434 -> [w1455 _]
          tunnel: w1428 -> [w1454 w1464]
          frame False {
            n504 = Scan From String(format string="%0.3f", input string=w1463, error in=w1454, default 1=0.0 ("default value 1")) -> (error out=w1453:errorcluster, output 1=w1461:dbl)  [unwired: 1 in, 2 out]
            n505 = String Subset(string=w1455, offset (0)=2, length (rest)=4 ("length (rest)")) -> (substring=w1459:string)
            n506 = Scan From String(input string=w1459, error in=w1453) -> (error out=w1452:errorcluster, output 1=w1456:dbl)  [unwired: 3 in, 2 out]
          }
          frame True {
          }
        }
        n507 = Match Pattern(string=w1434, regular expression="\n") -> (before substring=w1437:string)  [unwired: 1 in, 3 out]
        n508 = Replace Array Subset(array=w1447, new element=w1448, index=w1425) -> (w1449:dbl[])
        n509 = Bundle By Name(cluster=w1433, "AP Test Data.Database AP Data"=w1449, "AP Test Data.PMAC Read Counter"=w1436, "AP Test Data.Raw Sunshade AP Data"=w1437) -> (w1432:T1)
      }
      frame "AT Get PMAC3000 Data Glass", "AT Get PMAC3000 Data Sunshade", "AT Get PMAC3000 Data Sunshade02" {
        n510 = Unbundle By Name(w1485) -> ("AP Test Data.Database AP Data"=w1486:dbl[], "USBHandle"=w1467:i32, "PeakNumber"=w1480:i32, "Store Data.Error Table"=w1478:string[][], "Sequence State"=w1471:T24)
        n511 = case shown="\"AT Get PMAC3000 Data Glass\", 默认" w1483 {
          tunnel: [1 ("index") 3 ("index") 5 ("index")] -> w1482
          frame "AT Get PMAC3000 Data Glass", Default {
          }
          frame "AT Get PMAC3000 Data Sunshade" {
          }
          frame "AT Get PMAC3000 Data Sunshade02" {
          }
        }
        n512 = Increment(x=w1480) -> (x+1=w1479:i32)
        n513 = call "PMAC3000 get peak.vi"("Handle"=w1467) -> ("error out"=w1468:errorcluster, "peaknumber"=w1474:i32, "LivePeak"=w1481:sgl)  [unwired: 7 in, 1 out]
        n514 = Equal?(x=w1474, y=w1479) -> (x = y?=w1469:bool)
        n515 = dll-call lib="C:/Labview Code/04.SubVI's/Others VI's/FTD2XX.dll" fn="FT_Close"(error in=w1468, "Handle"=w1467) -> ()  [unwired: 4 in, 2 out]
        n516 = case shown="假" w1469 {
          tunnel: w1478 -> [w1491 w1494]
          tunnel: [w1490 w1494] -> w1477
          tunnel: w1476 -> [w1489 w1493]
          tunnel: [w1488 w1493] -> w1475
          frame False {
            n517 = call "EOL Error Table.vi"("error in"=w1489, "Error No."=u16 46, "Error Table In"=w1491) -> ("error out"=w1488:errorcluster, "Error Table Out"=w1490:string[][])  [unwired: 7 in]
          }
          frame True {
          }
        }
        n518 = call "pass fail action decision.vi"("Pass?"=w1469, "Sequence State in"=w1471, "event queue in"=w1473) -> ("Sequence State out"=w1470:T24, "Event queue out"=w1472:string[])  [unwired: 7 in]
        n519 = Replace Array Subset(array=w1486, new element=w1481, index=w1482) -> (w1487:dbl[])
        n520 = Bundle By Name(cluster=w1485, "AP Test Data.Database AP Data"=w1487, "PeakNumber"=w1474, "Store Data.Error Table"=w1477, "Sequence State"=w1470) -> (w1484:T1)
      }
      frame "AT Get PMAC3000 Peaknumber" {
        w1515 = string[] ["2.03", "2.04", "2.05", "2.06", "2.07", "2.08", "2.09"]  # VersionNumbers
        # "USB handle close"
        n521 = Unbundle By Name(w1513) -> ("USBHandle"=w1521:i32, "Store Data.Error Table"=w1503:string[][], "Sequence State"=w1505:T24)
        n522 = dll-call lib="C:/Labview Code/04.SubVI's/Others VI's/FTD2XX.dll" fn="FT_Close"(error in=w1510, "Handle"=w1521) -> (error out=w1500:errorcluster)  [unwired: 4 in, 1 out]
        n523 = call "Elapsed Time5"("error in (no error)"=w1500) -> ("Present (s)"=w1498:dbl, "error out"=w1499:errorcluster)  [unwired: 11 in, 6 out]
        n524 = while {
          tunnel: "90424" ("Software Number") -> [w1539]
          tunnel: 200 ("RD/WR Timeouts") -> [w1538]
          tunnel: u8 5 ("Latency Timer") -> [w1537]
          tunnel: T49 {"Baud Rate"=6000000, "DataBits"=8, "StopBits"=0, "Parity"=0} ("Data Set-Up") -> [w1536]
          tunnel: cluster{"FlowControl":u16, "Xon":u8, "Xoff":u8} {"FlowControl"=256, "Xon"=0, "Xoff"=0} ("Flow Control Input") -> [w1535]
          tunnel: w1515 -> [w1534]
          tunnel: w1499 -> [w1532]
          tunnel: [w1528] -> w1511
          tunnel: [w1531] -> w1508
          tunnel: [w1523] -> w1501
          tunnel: w1498 -> [w1526]
          stop <- w1522 stop-if-true
          n525 = call "PMAC3000 SetUpDeviceOnUSB.vi"("RD/WR Timeouts"=w1538, "Software Number"=w1539, "VersionNumbers"=w1534, "Latency Timer"=w1537, "Data Set-Up"=w1536, "Flow Control Input"=w1535, "Show Not Found Message"=FALSE, "error in (no error)"=w1532) -> ("USB Device Found"=w1523:bool, "USB Handle"=w1531:i32, "error out"=w1530:errorcluster)  [unwired: 2 in, 3 out]
          n526 = call "Elapsed Time4"("error in (no error)"=w1530) -> ("Present (s)"=w1527:dbl, "error out"=w1528:errorcluster)  [unwired: 11 in, 6 out]
          n527 = Subtract(x=w1527, y=w1526) -> (x-y=w1525:dbl)
          n528 = Greater Or Equal?(x=w1525, y=3.0) -> (x >= y?=w1524:bool)
          n529 = Or(x=w1523, y=w1524) -> (x .or. y?=w1522:bool)
        }
        n530 = case shown="真" w1501 {
          tunnel: w1508 -> [w1547 w1551]
          tunnel: [0 ("peaknumber") w1550] -> w1514
          tunnel: w1511 -> [w1545 w1549]
          tunnel: [w1544 w1548] -> w1509
          frame False {
            n531 = dll-call lib="C:/Labview Code/04.SubVI's/Others VI's/FTD2XX.dll" fn="FT_Close"(error in=w1545, "Handle"=w1547) -> (error out=w1544:errorcluster)  [unwired: 4 in, 1 out]
          }
          frame True {
            n532 = call "PMAC3000 get peak.vi"("error in (no error)"=w1549, "Handle"=w1551) -> ("error out"=w1548:errorcluster, "peaknumber"=w1550:i32)  [unwired: 6 in, 2 out]
          }
        }
        n533 = case shown="假" w1501 {
          tunnel: w1503 -> [w1541 w1543]
          tunnel: [w1540 w1543] -> w1502
          frame False {
            n534 = call "EOL Error Table.vi"("Error No."=u16 135, "Error Table In"=w1541) -> ("Error Table Out"=w1540:string[][])  [unwired: 8 in, 1 out]
          }
          frame True {
          }
        }
        n535 = call "pass fail action decision.vi"("Pass?"=w1501, "Sequence State in"=w1505, "event queue in"=w1507) -> ("Sequence State out"=w1504:T24, "Event queue out"=w1506:string[])  [unwired: 7 in]
        n536 = Bundle By Name(cluster=w1513, "USBHandle"=w1508, "PeakNumber"=w1514, "Store Data.Error Table"=w1502, "Sequence State"=w1504) -> (w1512:T1)
      }
      frame "AT Set Glass Wand Lower Bit", "AT Set Glass Wand Up Bit", "AT Set Sunshade Wand Lower Bit", "AT Set Sunshade Wand Up Bit", "AT Set Wand Home Position", "AT Set to Vent ATS pos", "AT Set to Vent Home pos" {
        n537 = Unbundle By Name(w1561) -> ("Store Data.Error Table"=w1560:string[][], "D in map.Abort Test"=w1559:T17, "Sequence State"=w1558:T24, "Config Info"=w1556:T34)
        n538 = call "Config Info Get.vi"("Config Info"=w1556) -> ("PLC Comms"=w1557:T56)  [unwired: 7 in, 3 out]
        n539 = Unbundle By Name(w1557) -> ("PLC bool write Tags.AT set glass wand lower"=w1583:T40, "PLC boolean read Tags.AT in glass wand lower pos"=w1586:T40, "PLC bool write Tags.AT set glass wand up"=w1553:T40, "PLC boolean read Tags.AT in glass wand up pos"=w1552:T40, "PLC bool write Tags.AT set sunshade wand lower"=w1581:T40, "PLC boolean read Tags.AT in sunshad wand lower pos"=w1578:T40, "PLC bool write Tags.AT set wand home pos"=w1580:T40, "PLC boolean read Tags.AT in wand home pos"=w1579:T40, "PLC bool write Tags.AT set sunshade wand up"=w1554:T40, "PLC boolean read Tags.AT in sunshad wand up pos"=w1555:T40, "PLC bool write Tags.AT set to Vent ATS Test Pos"=w1565:T40, "PLC boolean read Tags.AT at vent ATS test pos"=w1564:T40, "PLC bool write Tags.AT set to Vent ATS Home Pos"=w1563:T40, "PLC boolean read Tags.AT at vent ATS Home pos"=w1562:T40)
        n540 = case shown="\"AT Set to Vent Home pos\"" w1567 {
          tunnel: w1586 -> [w1593 _ _ _ _ _ _]
          tunnel: [w1593 w1594 w1598 w1602 w1606 w1610 w1613] -> w1587
          tunnel: [" - To Glass Position" ("Error Description") " - To Glass Position" ("Error Description") " - To Rollo Position" ("Error Description") " - To Rollo Position" ("Error Description") _ "to vent test position" ("Error Description") "to vent home position" ("Error Description")] -> w1585
          tunnel: [w1591 w1595 w1599 w1603 w1607 w1609 w1614] -> w1577
          tunnel: w1583 -> [w1591 _ _ _ _ _ _]
          tunnel: [u16 42 ("Error No.") u16 42 ("Error No.") u16 42 ("Error No.") u16 204 ("Error No.") u16 41 ("Error No.") u16 208 ("Error No.") u16 209 ("Error No.")] -> w1582
          tunnel: w1581 -> [_ _ w1599 _ _ _ _]
          tunnel: w1580 -> [_ _ _ _ w1607 _ _]
          tunnel: w1579 -> [_ _ _ _ w1606 _ _]
          tunnel: w1578 -> [_ _ w1598 _ _ _ _]
          tunnel: w1565 -> [_ _ _ _ _ w1609 _]
          tunnel: w1564 -> [_ _ _ _ _ w1610 _]
          tunnel: w1563 -> [_ _ _ _ _ _ w1614]
          tunnel: w1562 -> [_ _ _ _ _ _ w1613]
          tunnel: w1555 -> [_ _ _ w1602 _ _ _]
          tunnel: w1554 -> [_ _ _ w1603 _ _ _]
          tunnel: w1553 -> [_ w1595 _ _ _ _ _]
          tunnel: w1552 -> [_ w1594 _ _ _ _ _]
          frame "AT Set Glass Wand Lower Bit", Default {
          }
          frame "AT Set Glass Wand Up Bit" {
          }
          frame "AT Set Sunshade Wand Lower Bit" {
          }
          frame "AT Set Sunshade Wand Up Bit" {
          }
          frame "AT Set Wand Home Position" {
          }
          frame "AT Set to Vent ATS pos" {
          }
          frame "AT Set to Vent Home pos" {
          }
        }
        n541 = call "plc write bool.vi"("error in"=w1575, "value"=TRUE, "addr,tag"=w1577) -> ("error out"=w1574:errorcluster)  [unwired: 8 in]
        n542 = call "wait for plc bit.vi"("error in"=w1574, "tag"=w1587, "Abort Test"=w1559) -> ("error out"=w1573:errorcluster, "final values"=w1568:bool)  [unwired: 7 in]
        n543 = call "plc write bool.vi"("error in"=w1573, "value"=FALSE, "addr,tag"=w1577) -> ("error out"=w1576:errorcluster)  [unwired: 8 in]
        n544 = case shown="假" w1568 {
          tunnel: w1560 -> [w1622 w1624]
          tunnel: [w1621 w1624] -> w1589
          tunnel: w1576 -> [w1620 w1623]
          tunnel: w1585 -> [w1619 _]
          tunnel: [w1618 w1623] -> w1584
          tunnel: w1582 -> [w1617 _]
          frame False {
            n545 = call "EOL Error Table.vi"("Error Description"=w1619, "error in"=w1620, "Error No."=w1617, "Error Table In"=w1622) -> ("error out"=w1618:errorcluster, "Error Table Out"=w1621:string[][])  [unwired: 6 in]
          }
          frame True {
          }
        }
        n546 = call "pass fail action decision.vi"("Pass?"=w1568, "Sequence State in"=w1558, "event queue in"=w1570) -> ("Sequence State out"=w1566:T24, "Event queue out"=w1569:string[])  [unwired: 7 in]
        n547 = Bundle By Name(cluster=w1561, "Store Data.Error Table"=w1589, "Sequence State"=w1566) -> (w1588:T1)
      }
      frame "AT Get Side ATS data" {
        n548 = Unbundle By Name(w1641) -> ("AP Test Data.Database AP Data"=w1642:dbl[], "Station Index"=w1636:i32)  [unwired: 2 out]
        n549 = call "EOL All-Station AI Debug Buffer.vi"("station idx"=w1636, "Mode"=enum16{"Initialize", "Read", "Write"}."Read") -> ("Data Read (Samp-Ro, Ch-Col)"=w1637:sgl[][])  [unwired: 9 in]
        n550 = Index Array(array=w1637, index (col)=EOL_Analog_Input_Control."ATS" ("Analog Control")) -> (element=w1633:sgl[])  [unwired: 1 in]
        n551 = Array Max & Min(array=w1633) -> (max value=w1632:sgl)  [unwired: 3 out]
        n552 = Multiply(x=w1632, y=sgl 20.0) -> (x*y=w1627:sgl)
        n553 = Subtract(x=w1627, y=w1629) -> (x-y=w1628:dbl)
        n554 = Select(t=w1628, s=w1625, f=w1627) -> (s? t:f=w1626:dbl)
        n555 = Replace Array Subset(array=w1642, new element=w1626, index=1 ("数值")) -> (w1643:dbl[])
        n556 = Bundle By Name(cluster=w1641, "AP Test Data.Database AP Data"=w1643) -> (w1640:T1)
      }
      frame "AT Get Rollo ATS data" {
        n557 = Unbundle By Name(w1660) -> ("AP Test Data.Database AP Data"=w1661:dbl[], "Station Index"=w1655:i32)  [unwired: 2 out]
        n558 = call "EOL All-Station AI Debug Buffer.vi"("station idx"=w1655, "Mode"=enum16{"Initialize", "Read", "Write"}."Read") -> ("Data Read (Samp-Ro, Ch-Col)"=w1656:sgl[][])  [unwired: 9 in]
        n559 = Index Array(array=w1656, index (col)=EOL_Analog_Input_Control."ATS" ("Analog Control")) -> (element=w1652:sgl[])  [unwired: 1 in]
        n560 = Array Max & Min(array=w1652) -> (max value=w1651:sgl)  [unwired: 3 out]
        n561 = Multiply(x=w1651, y=sgl 20.0) -> (x*y=w1645:sgl)
        n562 = Subtract(x=w1645, y=w1647) -> (x-y=w1648:dbl)
        n563 = Select(t=w1648, s=w1646, f=w1645) -> (s? t:f=w1644:dbl)
        n564 = Replace Array Subset(array=w1661, new element=w1644, index=3 ("数值")) -> (w1662:dbl[])
        n565 = Bundle By Name(cluster=w1660, "AP Test Data.Database AP Data"=w1662) -> (w1659:T1)
      }
      frame "AT Get Vent ATS data" {
        # "防夹力传感器"
        n566 = Unbundle By Name(w1679) -> ("AP Test Data.Database AP Data"=w1680:dbl[], "Station Index"=w1674:i32)  [unwired: 2 out]
        n567 = call "EOL All-Station AI Debug Buffer.vi"("station idx"=w1674, "Mode"=enum16{"Initialize", "Read", "Write"}."Read") -> ("Data Read (Samp-Ro, Ch-Col)"=w1675:sgl[][])  [unwired: 9 in]
        n568 = Index Array(array=w1675, index (col)=EOL_Analog_Input_Control."ATS" ("Analog Control")) -> (element=w1671:sgl[])  [unwired: 1 in]
        n569 = Array Max & Min(array=w1671) -> (max value=w1670:sgl)  [unwired: 3 out]
        n570 = Multiply(x=w1670, y=sgl 20.0) -> (x*y=w1664:sgl)
        n571 = Subtract(x=w1664, y=w1666) -> (x-y=w1667:dbl)
        n572 = Select(t=w1667, s=w1665, f=w1664) -> (s? t:f=w1663:dbl)
        n573 = Replace Array Subset(array=w1680, new element=w1663, index=7 ("索引")) -> (w1681:dbl[])
        n574 = Bundle By Name(cluster=w1679, "AP Test Data.Database AP Data"=w1681) -> (w1678:T1)
      }
      frame "ATV Check Force Sensor at Home" {
        n575 = Unbundle By Name(w1684) -> ("Config Info"=w1685:T34)
        n576 = Unbundle By Name(w1684) -> ("Sequence State"=w1687:T24, "Store Data.Error Table"=w1694:string[][], "D in map.Abort Test"=w1696:T17)
        n577 = call "Config Info Get.vi"("Config Info"=w1685) -> ("PLC Comms"=w1683:T56)  [unwired: 7 in, 3 out]
        n578 = Unbundle By Name(w1683) -> ("PLC boolean read Tags.AT VentPMACatHome"=w1682:T40)
        n579 = call "wait for plc bit.vi"("error in"=w1692, "tag"=w1682, "Abort Test"=w1696) -> ("error out"=w1691:errorcluster, "final values"=w1690:bool)  [unwired: 7 in]
        n580 = case shown="假" w1690 {
          tunnel: w1694 -> [w1700 w1701]
          tunnel: [w1699 w1701] -> w1695
          frame False {
            n581 = call "EOL Error Table.vi"("Error Description"="-", "Error No."=u16 180 ("read tags"), "Error Table In"=w1700) -> ("Error Table Out"=w1699:string[][])  [unwired: 7 in, 1 out]
          }
          frame True {
          }
        }
        n582 = call "pass fail action decision.vi"("Pass?"=w1690, "Sequence State in"=w1687, "event queue in"=w1689) -> ("Sequence State out"=w1686:T24, "Event queue out"=w1688:string[])  [unwired: 7 in]
        n583 = Bundle By Name(cluster=w1684, "Sequence State"=w1686, "Store Data.Error Table"=w1695) -> (w1693:T1)
      }
      frame "ATV Retract Force Sensor" {
        n584 = Unbundle By Name(w1704) -> ("Config Info"=w1703:T34)
        n585 = call "Config Info Get.vi"("Config Info"=w1703) -> ("PLC Comms"=w1702:T56)  [unwired: 7 in, 3 out]
        n586 = Unbundle By Name(w1702) -> ("PLC bool write Tags.AT VentPMACExtended"=w1706:T40, "PLC bool write Tags.AT VentPMACHome"=w1705:T40)
        n587 = flat-sequence {
          tunnel: w1706 -> [w1708]
          tunnel: w1705 -> [w1711]
          frame #0 {
            n588 = call "plc write bool.vi"("value"=FALSE, "addr,tag"=w1708) -> ()  [unwired: 9 in, 1 out]
          }
          frame #1 {
            n589 = call "plc write bool.vi"("value"=TRUE, "addr,tag"=w1711) -> ()  [unwired: 9 in, 1 out]
          }
        }
      }
      frame "ATV Set Force Sensor" {
        n590 = Unbundle By Name(w1714) -> ("Config Info"=w1713:T34)
        n591 = call "Config Info Get.vi"("Config Info"=w1713) -> ("PLC Comms"=w1712:T56)  [unwired: 7 in, 3 out]
        n592 = Unbundle By Name(w1712) -> ("PLC bool write Tags.AT VentPMACExtended"=w1716:T40, "PLC bool write Tags.AT VentPMACHome"=w1715:T40)
        n593 = flat-sequence {
          tunnel: w1715 -> [w1718]
          tunnel: w1716 -> [w1721]
          frame #0 {
            n594 = call "plc write bool.vi"("value"=FALSE, "addr,tag"=w1718) -> ()  [unwired: 9 in, 1 out]
          }
          frame #1 {
            n595 = call "plc write bool.vi"("value"=TRUE, "addr,tag"=w1721) -> ()  [unwired: 9 in, 1 out]
          }
        }
      }
      frame "ATV check Force Sensor Extended" {
        n596 = Unbundle By Name(w1725) -> ("Config Info"=w1724:T34)
        n597 = Unbundle By Name(w1725) -> ("Store Data.Error Table"=w1734:string[][], "D in map.Abort Test"=w1737:T17, "Sequence State"=w1727:T24)
        n598 = call "Config Info Get.vi"("Config Info"=w1724) -> ("PLC Comms"=w1723:T56)  [unwired: 7 in, 3 out]
        n599 = Unbundle By Name(w1723) -> ("PLC boolean read Tags.AT VentPMACisExtend"=w1722:T40)
        n600 = call "wait for plc bit.vi"("error in"=w1735, "tag"=w1722, "Abort Test"=w1737) -> ("error out"=w1732:errorcluster, "final values"=w1730:bool)  [unwired: 7 in]
        n601 = case shown="假" w1730 {
          tunnel: w1734 -> [w1743 w1745]
          tunnel: [w1740 w1745] -> w1733
          tunnel: w1732 -> [w1739 w1744]
          tunnel: [w1738 w1744] -> w1731
          frame False {
            n602 = call "EOL Error Table.vi"("Error Description"="-", "error in"=w1739, "Error No."=u16 179 ("read tags"), "Error Table In"=w1743) -> ("error out"=w1738:errorcluster, "Error Table Out"=w1740:string[][])  [unwired: 6 in]
          }
          frame True {
          }
        }
        n603 = call "pass fail action decision.vi"("Pass?"=w1730, "Sequence State in"=w1727, "event queue in"=w1729) -> ("Sequence State out"=w1726:T24, "Event queue out"=w1728:string[])  [unwired: 7 in]
        n604 = Bundle By Name(cluster=w1725, "Store Data.Error Table"=w1733, "Sequence State"=w1726) -> (w1736:T1)
      }
      frame "--------Sequence--------" {
      }
      frame "Check Sequence" {
        n605 = Unbundle By Name(w1756) -> ("Sequence State.Active Step"=w1758:u8, "Sequence State.Seqence"=w1759:T25[], "Sequence State.Pass?"=w1751:bool, "Sequence State.Red-Rabbit Mode"=w1750:bool)
        n606 = Array Size(array=w1759) -> (size(s)=w1760:i32)
        n607 = Increment(x=w1758) -> (x+1=w1754:u8)
        n608 = Compound Arithmetic op=AND(invert w1751, invert w1750) -> (w1749:bool)
        n609 = Greater Or Equal?(x=w1754, y=w1760) -> (x >= y?=w1752:bool)
        n610 = Or(x=w1752, y=w1749) -> (x .or. y?=w1753:bool)
        n611 = case shown="真" w1753 {
          tunnel: [string[] ["Execute Step"] ("event queue out") string[] ["Sequence Complete"] ("event queue out")] -> w1757
          frame False {
          }
          frame True {
          }
        }
        n612 = Bundle By Name(cluster=w1756, "Sequence State.Active Step"=w1754) -> (w1755:T1)
      }
      frame "Execute Step" {
        w1770 = All_Motions."Idle"  # Motion Data.Current Motion
        n613 = Unbundle By Name(w1775) -> ("Station Index"=w1766:i32, "ctl refs.all station status"=w1777:refnum<vi>, "misc station config.Station Name"=w1780:string, "Sequence State.Seqence"=w1787:T25[], "Sequence State.Active Step"=w1785:u8, "Station Index"=w1773:i32, "misc status.PS Voltage"=w1769:dbl, "misc status.Part Setup.Motor Type"=w1768:T30)  [unwired: 2 out]
        n614 = case shown="\"Smart Motor\", 默认" w1768 {
          tunnel: [string[] ["Init Motion", "Set Power Supply", "NVH Test Needed?", "Set Switch Output", "Check Switch Signals", "Check Initial Motion", "Get Data"] ("event queue out") string[] ["Init Motion", "BMW Init Motion", "Set Power Supply", "NVH Test Needed?", "Set Switch Output", "Check Initial Motion", "BMW Check Hall Movement", "BMW Get Data", "BMW Check Motion Stop"] ("event queue out")] -> w1767
          frame "Smart Motor", Default {
          }
          frame "Sensor Motor" {
          }
        }
        n615 = Index Array(array=w1787, index=w1785) -> (element=w1786:T25)
        n616 = property class="Clust (严格)"(reference=w1777) -> (reference out=w1764:refnum<vi>, error out=w1778:errorcluster, "Value"=w1779:T52)  [unwired: 1 in]
        n617 = Unbundle By Name(w1786) -> ("Name"=w1776:string, "data string"=w1784:string, "Description"=w1781:string)
        n618 = Bundle By Name(cluster=w1779, "Current Step Br"=w1776) -> (w1763:T52)
        n619 = property class="Clust (严格)"(reference=w1764, error in=w1778, "Value"=w1763) -> ()  [unwired: 2 out]
        n620 = Bundle By Name(cluster=w1775, "Motion Status.Motion"=w1770, "manual control(direct)"=FALSE ("goto motion?")) -> (w1774:T1)
        n621 = case shown="\"Glass Teach\", \"Sunshade Teach\", \"Sunshade Teach 2\"" w1776 {
          selector: w1776 -> [w1791 _ w1810 _ _ _ _ _ _ _ _ _ _ _ _ _ _ _ _ w1967 _ _ _ _ _ _ w2023 w2047 _ _ _ _ _ _ _ _ _ _ _ _ _ _ _ _ w2221]
          tunnel: w1784 -> [w1794 w1805 w1815 w1819 w1830 w1841 w1850 w1857 w1868 w1877 w1886 w1895 w1904 w1909 w1922 w1930 w1940 w1947 w1958 w1966 w1980 w1985 w1992 w2001 w2006 w2013 w2028 w2049 w2085 w2090 w2097 w2106 w2111 w2118 w2139 w2147 w2157 w2164 w2171 w2178 w2183 w2192 w2201 w2210 w2222]
          tunnel: w1774 -> [w1799 w1807 w1818 w1826 w1835 w1844 w1853 w1862 w1871 w1880 w1889 w1898 w1907 w1916 w1925 w1934 w1943 w1952 w1961 w1969 w1979 w1987 w1994 w2000 w2008 w2015 w2024 w2051 w2084 w2092 w2099 w2105 w2113 w2120 w2143 w2150 w2156 w2163 w2170 w2177 w2187 w2196 w2205 w2214 w2223]
          tunnel: [w1800 w1801 w1817 w1824 w1833 w1842 w1851 w1860 w1869 w1878 w1887 w1896 w1905 w1914 w1923 w1932 w1941 w1950 w1959 w1968 w1975 w1982 w1989 w1996 w2003 w2010 w2017 w2050 w2080 w2087 w2094 w2101 w2108 w2115 w2122 w2151 w2152 w2159 w2166 w2173 w2186 w2195 w2204 w2213 w2216] -> w1783
          tunnel: [string[] ["Check Position Software", "Check Sequence"] string[] ["Delay", "Check Sequence"] w1811 w1821 w1831 w1839 w1848 w1858 w1866 w1875 w1884 w1892 w1901 w1910 w1919 w1929 w1937 w1946 w1955 w1964 w1977 w1983 w1990 w1998 w2004 w2011 w2018 w2046 w2082 w2088 w2095 w2103 w2109 w2116 string[] ["Init Motion", "Set Power Supply", "NVH Test Needed?", "Set Switch Output", "Send Go To Position Message", "Check Enter AP Message Mode", "Check Hall position for go to position", "Check Sequence"] ("event queue out") string[] ["Set Power Supply", "Check Sequence"] w2154 w2161 w2168 w2175 string[] ["Init Motion", "Direct control set switch output", "DirectControl"] ("event queue out") string[] ["Init Motion", "Direct control set switch output", "DirectControl"] ("event queue out") string[] ["Init Motion", "Direct control set switch output", "DirectControl"] ("event queue out") string[] ["Init Motion", "Direct control set switch output", "DirectControl"] ("event queue out") w2220] -> w1782
          tunnel: w1781 -> [_ w1804 _ _ _ _ _ _ _ _ _ _ _ _ _ _ _ _ _ _ _ _ _ _ _ _ _ w2048 _ _ _ _ _ _ _ _ _ _ _ _ w2184 w2193 w2202 w2211 w2218]
          tunnel: w1767 -> [_ _ _ w1823 w1832 w1840 w1849 w1859 w1867 w1876 w1885 w1894 w1903 w1911 w1921 w1931 w1939 w1949 w1957 w1964 w1977 w1983 w1990 w1998 w2004 w2011 w2018 _ w2082 w2088 w2095 w2103 w2109 w2116 _ _ w2154 w2161 w2168 w2175 _ _ _ _ _]
          tunnel: w1780 -> [_ _ _ _ _ _ _ _ _ _ _ _ _ _ _ _ _ _ _ _ _ _ _ _ _ _ _ _ _ _ _ _ _ _ _ _ _ _ _ _ _ _ _ _ _]
          tunnel: w1773 -> [_ _ _ _ _ _ _ _ _ _ _ _ _ _ _ _ _ _ _ _ _ _ _ _ _ _ w2025 _ _ _ _ _ _ _ _ _ _ _ _ _ _ _ _ _ _]
          tunnel: w1772 -> [w1793 w1802 w1816 w1822 w1829 w1838 w1847 w1856 w1865 w1874 w1883 w1893 w1902 w1913 w1920 w1928 w1938 w1948 w1956 w1965 w1976 w1984 w1991 w1997 w2005 w2012 w2019 w2053 w2081 w2089 w2096 w2102 w2110 w2117 w2138 w2145 w2153 w2160 w2167 w2174 w2188 w2197 w2206 w2215 w2217]
          tunnel: [w1793 w1802 w1816 w1820 w1828 w1837 w1846 w1855 w1864 w1873 w1882 w1891 w1900 w1912 w1918 w1927 w1936 w1945 w1954 w1965 w1976 w1984 w1991 w1997 w2005 w2012 w2019 w2053 w2081 w2089 w2096 w2102 w2110 w2117 w2132 w2144 w2153 w2160 w2167 w2174 w2188 w2197 w2206 w2215 w2217] -> w1771
          tunnel: w1769 -> [_ _ _ _ _ _ _ _ _ _ _ _ _ _ _ _ _ _ _ _ _ _ _ _ _ _ _ _ _ _ _ _ _ _ w2126 _ _ _ _ _ _ _ _ _ _]
          tunnel: w1768 -> [_ _ _ _ _ _ _ _ _ _ _ _ _ _ _ _ _ _ _ _ _ _ _ _ _ _ _ _ _ _ _ _ _ _ _ _ _ _ _ _ _ _ _ _ _]
          tunnel: w1766 -> [_ _ _ _ _ _ _ _ _ _ _ _ _ _ _ _ _ _ _ _ _ _ _ _ _ _ _ _ _ _ _ _ _ _ _ _ _ _ _ _ _ _ _ _ _]
          tunnel: w1764 -> [_ _ _ _ _ _ _ _ _ _ _ _ _ _ _ _ _ _ _ _ _ _ _ _ _ _ _ w2045 _ _ _ _ _ _ _ _ _ _ _ _ _ _ _ _ _]
          tunnel: w1763 -> [_ _ _ _ _ _ _ _ _ _ _ _ _ _ _ _ _ _ _ _ _ _ _ _ _ _ _ w2044 _ _ _ _ _ _ _ _ _ _ _ _ _ _ _ _ _]
          frame "Check Position Software Glass", "Check Position Software Sunshade" {
            n622 = Scan From String(format string="%x", input string=w1794, default 1=u8 0 ("Hex Number")) -> (output 1=w1795:u8)  [unwired: 2 in, 3 out]
            n623 = Equal?(x=w1791, y="Check Position Software Glass") -> (x = y?=w1790:bool)
            n624 = Bundle By Name(cluster=w1799, "Motion Status.Motor Position Hex"=w1795, "misc status.Serial Port Configured?"=w1790) -> (w1800:T1)
          }
          frame "Delay In Seconds" {
            n625 = Tick Count (ms)() -> (millisecond timer value=w1803:u32)
            n626 = Bundle By Name(cluster=w1807, "Sequence State.Step Data String"=w1805, "Sequence State.Step Description"=w1804, "misc status.delay start time (ticks)"=w1803) -> (w1801:T1)
          }
          frame "Enter AP Message Mode Glass", "Enter AP Message Mode Sunshade" {
            n627 = Scan From String(input string=w1815, default 1=17x_AP_Data_Type."91/61" ("AP Data Type")) -> (output 1=w1813:T13)  [unwired: 3 in, 3 out]
            n628 = Equal?(x=w1810, y="Enter AP Message Mode Glass") -> (x = y?=w1809:bool)
            n629 = Bundle By Name(cluster=w1818, "misc status.AP Data Type"=w1813, "misc status.Serial Port Configured?"=w1809) -> (w1817:T1)
            n630 = Build Array (concatenate)(w1810, string[] ["Check Sequence"]) -> (w1811:string[])
          }
          frame "Express Glass Slide Close" {
            n631 = call "Expr_Event Select.vi"("data string"=w1819, "错误输入（无错误）"=w1822, "event queue in"=w1823) -> ("错误输出"=w1820:errorcluster, "event queue out"=w1821:string[])  [unwired: 7 in]
            n632 = Bundle By Name(cluster=w1826, "Motion Status.Motion"=All_Motions."Express Glass Slide Close" ("Current Motion"), "Sequence State.Step Data String"=w1819, "misc status.Serial Port Configured?"=TRUE ("Glass Motor?")) -> (w1824:T1)
          }
          frame "Express Glass Slide Close Sunshade Close" {
            n633 = call "Expr_Event Select.vi"("data string"=w1830, "错误输入（无错误）"=w1829, "event queue in"=w1832) -> ("错误输出"=w1828:errorcluster, "event queue out"=w1831:string[])  [unwired: 7 in]
            n634 = Bundle By Name(cluster=w1835, "Motion Status.Motion"=All_Motions."Express Glass Slide Close Sunshade Close" ("Current Motion"), "Sequence State.Step Data String"=w1830, "misc status.Serial Port Configured?"=TRUE ("Glass Motor?")) -> (w1833:T1)
          }
          frame "Express Glass Slide Close Sunshade Open" {
            n635 = call "Expr_Event Select.vi"("data string"=w1841, "错误输入（无错误）"=w1838, "event queue in"=w1840) -> ("错误输出"=w1837:errorcluster, "event queue out"=w1839:string[])  [unwired: 7 in]
            n636 = Bundle By Name(cluster=w1844, "Motion Status.Motion"=All_Motions."Express Glass Slide Close Sunshade Open" ("Current Motion"), "Sequence State.Step Data String"=w1841, "misc status.Serial Port Configured?"=TRUE ("Glass Motor?")) -> (w1842:T1)
          }
          frame "Express Glass Slide Open" {
            n637 = call "Expr_Event Select.vi"("data string"=w1850, "错误输入（无错误）"=w1847, "event queue in"=w1849) -> ("错误输出"=w1846:errorcluster, "event queue out"=w1848:string[])  [unwired: 7 in]
            n638 = Bundle By Name(cluster=w1853, "Motion Status.Motion"=All_Motions."Express Glass Slide Open" ("Current Motion"), "Sequence State.Step Data String"=w1850, "misc status.Serial Port Configured?"=TRUE ("Glass Motor?")) -> (w1851:T1)
          }
          frame "Express Glass Slide Open Sunshade Close" {
            n639 = call "Expr_Event Select.vi"("data string"=w1857, "错误输入（无错误）"=w1856, "event queue in"=w1859) -> ("错误输出"=w1855:errorcluster, "event queue out"=w1858:string[])  [unwired: 7 in]
            n640 = Bundle By Name(cluster=w1862, "Motion Status.Motion"=All_Motions."Express Glass Slide Open Sunshade Close" ("Current Motion"), "Sequence State.Step Data String"=w1857, "misc status.Serial Port Configured?"=TRUE ("Glass Motor?")) -> (w1860:T1)
          }
          frame "Express Glass Slide Open Sunshade Open" {
            n641 = call "Expr_Event Select.vi"("data string"=w1868, "错误输入（无错误）"=w1865, "event queue in"=w1867) -> ("错误输出"=w1864:errorcluster, "event queue out"=w1866:string[])  [unwired: 7 in]
            n642 = Bundle By Name(cluster=w1871, "Motion Status.Motion"=All_Motions."Express Glass Slide Open Sunshade Open" ("Current Motion"), "Sequence State.Step Data String"=w1868, "misc status.Serial Port Configured?"=TRUE ("Glass Motor?")) -> (w1869:T1)
          }
          frame "Express Glass Vent Close" {
            n643 = call "Expr_Event Select.vi"("data string"=w1877, "错误输入（无错误）"=w1874, "event queue in"=w1876) -> ("错误输出"=w1873:errorcluster, "event queue out"=w1875:string[])  [unwired: 7 in]
            n644 = Bundle By Name(cluster=w1880, "Motion Status.Motion"=All_Motions."Express Glass Vent Close" ("Current Motion"), "Sequence State.Step Data String"=w1877, "misc status.Serial Port Configured?"=TRUE ("Glass Motor?")) -> (w1878:T1)
          }
          frame "Express Glass Vent Close Sunshade Close" {
            n645 = call "Expr_Event Select.vi"("data string"=w1886, "错误输入（无错误）"=w1883, "event queue in"=w1885) -> ("错误输出"=w1882:errorcluster, "event queue out"=w1884:string[])  [unwired: 7 in]
            n646 = Bundle By Name(cluster=w1889, "Motion Status.Motion"=All_Motions."Express Glass Vent Close Sunshade Close" ("Current Motion"), "Sequence State.Step Data String"=w1886, "misc status.Serial Port Configured?"=TRUE ("Glass Motor?")) -> (w1887:T1)
          }
          frame "Express Glass Vent Close Sunshade Open" {
            n647 = call "Expr_Event Select.vi"("data string"=w1895, "错误输入（无错误）"=w1893, "event queue in"=w1894) -> ("错误输出"=w1891:errorcluster, "event queue out"=w1892:string[])  [unwired: 7 in]
            n648 = Bundle By Name(cluster=w1898, "Motion Status.Motion"=All_Motions."Express Glass Vent Close Sunshade Open" ("Current Motion"), "Sequence State.Step Data String"=w1895, "misc status.Serial Port Configured?"=TRUE ("Glass Motor?")) -> (w1896:T1)
          }
          frame "Express Glass Vent Open" {
            n649 = call "Expr_Event Select.vi"("data string"=w1904, "错误输入（无错误）"=w1902, "event queue in"=w1903) -> ("错误输出"=w1900:errorcluster, "event queue out"=w1901:string[])  [unwired: 7 in]
            n650 = Bundle By Name(cluster=w1907, "Motion Status.Motion"=All_Motions."Express Glass Vent Open" ("Current Motion"), "Sequence State.Step Data String"=w1904, "misc status.Serial Port Configured?"=TRUE ("Glass Motor?")) -> (w1905:T1)
          }
          frame "Express Sunshade Close" {
            n651 = call "Expr_Event Select.vi"("data string"=w1909, "错误输入（无错误）"=w1913, "event queue in"=w1911) -> ("错误输出"=w1912:errorcluster, "event queue out"=w1910:string[])  [unwired: 7 in]
            n652 = Bundle By Name(cluster=w1916, "Motion Status.Motion"=All_Motions."Express Sunshade Close" ("Current Motion"), "Sequence State.Step Data String"=w1909, "misc status.Serial Port Configured?"=FALSE ("Glass Motor?")) -> (w1914:T1)
          }
          frame "Express Sunshade Close 2" {
            n653 = call "Expr_Event Select.vi"("data string"=w1922, "错误输入（无错误）"=w1920, "event queue in"=w1921) -> ("错误输出"=w1918:errorcluster, "event queue out"=w1919:string[])  [unwired: 7 in]
            n654 = Bundle By Name(cluster=w1925, "Motion Status.Motion"=All_Motions."Express Sunshade Close 2" ("Current Motion"), "Sequence State.Step Data String"=w1922, "misc status.Serial Port Configured?"=FALSE ("Glass Motor?")) -> (w1923:T1)
          }
          frame "Express Sunshade Open" {
            n655 = call "Expr_Event Select.vi"("data string"=w1930, "错误输入（无错误）"=w1928, "event queue in"=w1931) -> ("错误输出"=w1927:errorcluster, "event queue out"=w1929:string[])  [unwired: 7 in]
            n656 = Bundle By Name(cluster=w1934, "Motion Status.Motion"=All_Motions."Express Sunshade Open" ("Current Motion"), "Sequence State.Step Data String"=w1930, "misc status.Serial Port Configured?"=FALSE ("Glass Motor?")) -> (w1932:T1)
          }
          frame "Express Sunshade Open 2" {
            n657 = call "Expr_Event Select.vi"("data string"=w1940, "错误输入（无错误）"=w1938, "event queue in"=w1939) -> ("错误输出"=w1936:errorcluster, "event queue out"=w1937:string[])  [unwired: 7 in]
            n658 = Bundle By Name(cluster=w1943, "Motion Status.Motion"=All_Motions."Express Sunshade Open 2" ("Current Motion"), "Sequence State.Step Data String"=w1940, "misc status.Serial Port Configured?"=FALSE ("Glass Motor?")) -> (w1941:T1)
          }
          frame "Express Vent Open Sunshade Close" {
            n659 = call "Expr_Event Select.vi"("data string"=w1947, "错误输入（无错误）"=w1948, "event queue in"=w1949) -> ("错误输出"=w1945:errorcluster, "event queue out"=w1946:string[])  [unwired: 7 in]
            n660 = Bundle By Name(cluster=w1952, "Motion Status.Motion"=All_Motions."Express Glass Vent Open Sunshade Close" ("Current Motion"), "Sequence State.Step Data String"=w1947, "misc status.Serial Port Configured?"=TRUE ("Glass Motor?")) -> (w1950:T1)
          }
          frame "Express Vent Open Sunshade Open" {
            n661 = call "Expr_Event Select.vi"("data string"=w1958, "错误输入（无错误）"=w1956, "event queue in"=w1957) -> ("错误输出"=w1954:errorcluster, "event queue out"=w1955:string[])  [unwired: 7 in]
            n662 = Bundle By Name(cluster=w1961, "Motion Status.Motion"=All_Motions."Express Glass Vent Open Sunshade Open" ("Current Motion"), "Sequence State.Step Data String"=w1958, "misc status.Serial Port Configured?"=TRUE ("Glass Motor?")) -> (w1959:T1)
          }
          frame "Glass Goto Position", "Sunshade Goto Position" {
            (unwired) TRUE ("goto motion?")
            # "for BMW, still use glass/ss open/close motions because\nin the 'set switch output' code we need the proper relays set,\nwhereas we dont care with smart motors becuase no switches\nwill be set anyway."
            n663 = case shown="\"Glass Goto Position\"" w1967 {
              tunnel: [All_Motions."Goto Position Sunshade" ("Current Motion") All_Motions."Goto Position Glass" ("Current Motion")] -> w1963
              tunnel: [FALSE TRUE] -> w1970
              frame "Sunshade Goto Position", Default {
              }
              frame "Glass Goto Position" {
              }
            }
            n664 = Bundle By Name(cluster=w1969, "Motion Status.Motion"=w1963, "Sequence State.Step Data String"=w1966, "misc status.Serial Port Configured?"=w1970) -> (w1968:T1)
          }
          frame "Glass Slide Close" {
            n665 = Bundle By Name(cluster=w1979, "Motion Status.Motion"=All_Motions."Glass Slide Close" ("Current Motion"), "Sequence State.Step Data String"=w1980, "misc status.Serial Port Configured?"=TRUE ("Glass Motor?")) -> (w1975:T1)
          }
          frame "Glass Slide Close Sunshade Close" {
            n666 = Bundle By Name(cluster=w1987, "Motion Status.Motion"=All_Motions."Glass Slide Close Sunshade Close" ("Current Motion"), "Sequence State.Step Data String"=w1985, "misc status.Serial Port Configured?"=TRUE ("Glass Motor?")) -> (w1982:T1)
          }
          frame "Glass Slide Close Sunshade Open" {
            n667 = Bundle By Name(cluster=w1994, "Motion Status.Motion"=All_Motions."Glass Slide Close Sunshade Open" ("Current Motion"), "Sequence State.Step Data String"=w1992, "misc status.Serial Port Configured?"=TRUE ("Glass Motor?")) -> (w1989:T1)
          }
          frame "Glass Slide Open" {
            n668 = Bundle By Name(cluster=w2000, "Motion Status.Motion"=All_Motions."Glass Slide Open" ("Current Motion"), "Sequence State.Step Data String"=w2001, "misc status.Serial Port Configured?"=TRUE ("Glass Motor?")) -> (w1996:T1)
          }
          frame "Glass Slide Open Sunshade Close" {
            n669 = Bundle By Name(cluster=w2008, "Motion Status.Motion"=All_Motions."Glass Slide Open Sunshade Close" ("Current Motion"), "Sequence State.Step Data String"=w2006, "misc status.Serial Port Configured?"=TRUE ("Glass Motor?")) -> (w2003:T1)
          }
          frame "Glass Slide Open Sunshade Open" {
            n670 = Bundle By Name(cluster=w2015, "Motion Status.Motion"=All_Motions."Glass Slide Open Sunshade Open" ("Current Motion"), "Sequence State.Step Data String"=w2013, "misc status.Serial Port Configured?"=TRUE ("Glass Motor?")) -> (w2010:T1)
          }
          frame "Glass Teach", "Sunshade Teach", "Sunshade Teach 2" {
            n671 = Multiply(x=w2025, y=2) -> (x*y=w2022:i32)
            n672 = case shown="\"Glass Teach\", 默认" w2023 {
              tunnel: [w2033 w2036 w2040] -> _
              tunnel: w2022 -> [w2033 w2037 w2041]
              tunnel: [All_Motions."Glass Teach" ("Current Motion") All_Motions."Sunshade Teach" ("Current Motion") All_Motions."Sunshade Teach 2" ("Current Motion")] -> w2021
              tunnel: [TRUE ("Glass Motor?") FALSE ("Glass Motor?") FALSE ("Glass Motor?")] -> w2020
              frame "Glass Teach", Default {
              }
              frame "Sunshade Teach" {
                n673 = Increment(x=w2037) -> (x+1=w2036:i32)
              }
              frame "Sunshade Teach 2" {
                n674 = Increment(x=w2041) -> (x+1=w2040:i32)
              }
            }
            n675 = Scan From String(format string="%0.2f", input string=w2028) -> (output 1=w2027:dbl)  [unwired: 3 in, 3 out]
            n676 = Bundle By Name(cluster=w2024, "Motion Status.Motion"=w2021, "misc status.PS Voltage"=w2027, "Sequence State.Step Data String"="", "misc status.Serial Port Configured?"=w2020) -> (w2017:T1)
          }
          frame "Send LIN Message for inalfa SCU" {
            n677 = Match Pattern(string=w2048, regular expression=", ") -> (before substring=w2042:string)  [unwired: 1 in, 3 out]
            n678 = Bundle By Name(cluster=w2044, "Current Step Br"=w2042) -> (w2043:T52)
            n679 = case shown="默认" w2042 {
              tunnel: w2051 -> [w2060 w2067 w2073 w2079]
              tunnel: [w2059 w2066 w2072 w2078] -> w2050
              tunnel: w2049 -> [w2058 w2065 w2071 w2077]
              tunnel: w2048 -> [w2057 w2064 w2070 w2076]
              tunnel: w2047 -> [w2056 _ _ _]
              tunnel: [w2054 string[] ["Init Motion", "Set Power Supply", "Send LIN Message for inalfa SCU", "Check Initial Motion", "Get Data"] ("event queue out") string[] ["Init Motion", "Set Power Supply", "NVH Test Needed?", "Send LIN Message for inalfa SCU", "Check Initial Motion", "Get Data"] ("event queue out") string[] ["Init Motion", "Set Power Supply", "NVH Test Needed?", "Send LIN Message for inalfa SCU", "Check Initial Motion", "Get Data"] ("event queue out")] -> w2046
              frame Default {
                n680 = Bundle By Name(cluster=w2060, "Sequence State.Step Data String"=w2058, "Sequence State.Step Description"=w2057) -> (w2059:T1)
                n681 = Build Array(w2056, "Check Sequence" ("element")) -> (w2054:string[])
              }
              frame "Inalfa SCU Teach" {
                (unwired) string[] ["Init Motion", "Set Power Supply", "Check Initial Position", "NVH Test Needed?", "Check Enter AP Message Mode", "Send LIN Message for inalfa SCU", "Check Switch Signals", "Check Initial Motion", "Get Data"] ("event queue out")
                n682 = Bundle By Name(cluster=w2067, "Motion Status.Motion"=All_Motions."Glass Teach", "Sequence State.Step Data String"=w2065, "Sequence State.Step Description"=w2064, "misc status.Serial Port Configured?"=TRUE) -> (w2066:T1)
              }
              frame "Go to position glass" {
                (unwired) string[] ["Init Motion", "Set Power Supply", "Check Initial Position", "NVH Test Needed?", "Check Enter AP Message Mode", "Send LIN Message for inalfa SCU", "Check Switch Signals", "Check Initial Motion", "Get Data"] ("event queue out")
                n683 = Bundle By Name(cluster=w2073, "Motion Status.Motion"=All_Motions."Goto Position Glass", "Sequence State.Step Data String"=w2071, "Sequence State.Step Description"=w2070) -> (w2072:T1)
              }
              frame "Go to position sunshade" {
                (unwired) string[] ["Init Motion", "Set Power Supply", "Check Initial Position", "NVH Test Needed?", "Check Enter AP Message Mode", "Send LIN Message for inalfa SCU", "Check Switch Signals", "Check Initial Motion", "Get Data"] ("event queue out")
                n684 = Bundle By Name(cluster=w2079, "Motion Status.Motion"=All_Motions."Goto Position Sunshade", "Sequence State.Step Data String"=w2077, "Sequence State.Step Description"=w2076) -> (w2078:T1)
              }
            }
            n685 = property class="Clust (严格)"(reference=w2045, "Value"=w2043) -> ()  [unwired: 1 in, 2 out]
          }
          frame "Glass Vent Close" {
            n686 = Bundle By Name(cluster=w2084, "Motion Status.Motion"=All_Motions."Glass Vent Close" ("Current Motion"), "Sequence State.Step Data String"=w2085, "misc status.Serial Port Configured?"=TRUE ("Glass Motor?")) -> (w2080:T1)
          }
          frame "Glass Vent Close Sunshade Close" {
            n687 = Bundle By Name(cluster=w2092, "Motion Status.Motion"=All_Motions."Glass Vent Close Sunshade Close" ("Current Motion"), "Sequence State.Step Data String"=w2090, "misc status.Serial Port Configured?"=TRUE ("Glass Motor?")) -> (w2087:T1)
          }
          frame "Glass Vent Close Sunshade Open" {
            n688 = Bundle By Name(cluster=w2099, "Motion Status.Motion"=All_Motions."Glass Vent Close Sunshade Open" ("Current Motion"), "Sequence State.Step Data String"=w2097, "misc status.Serial Port Configured?"=TRUE ("Glass Motor?")) -> (w2094:T1)
          }
          frame "Glass Vent Open" {
            n689 = Bundle By Name(cluster=w2105, "Motion Status.Motion"=All_Motions."Glass Vent Open" ("Current Motion"), "Sequence State.Step Data String"=w2106, "misc status.Serial Port Configured?"=TRUE ("Glass Motor?")) -> (w2101:T1)
          }
          frame "Glass Vent Open Sunshade Close" {
            n690 = Bundle By Name(cluster=w2113, "Motion Status.Motion"=All_Motions."Glass Vent Open Sunshade Close" ("Current Motion"), "Sequence State.Step Data String"=w2111, "misc status.Serial Port Configured?"=TRUE ("Glass Motor?")) -> (w2108:T1)
          }
          frame "Glass Vent Open Sunshade Open" {
            n691 = Bundle By Name(cluster=w2120, "Motion Status.Motion"=All_Motions."Glass Vent Open Sunshade Open" ("Current Motion"), "Sequence State.Step Data String"=w2118, "misc status.Serial Port Configured?"=TRUE ("Glass Motor?")) -> (w2115:T1)
          }
          frame "Go To Position" {
            # "this is only here for reverse compatibility - the user should\nuse the full blown 'glass goto postion' and 'sunshade goto position'\nsteps becuase those have many more options."
            n692 = Unflatten From String(type=T50 {"AP Data Type"=enum."91/61", "Glass Motor?"=FALSE, "Collect AP Data?"=FALSE, "Go To Position"=10, "Rear Rollo?"=FALSE} ("Goto Position Control"), binary string=w2139, error in (no error)=w2138) -> (value=w2136:T50, error out=w2133:errorcluster)  [unwired: 2 in, 1 out]
            n693 = Unbundle By Name(w2136) -> ("AP Data Type"=w2129:T13, "Glass Motor?"=w2135:bool, "Collect AP Data?"=w2128:bool, "Go To Position"=w2127:u16, "Rear Rollo?"=w2124:bool)
            n694 = Bundle By Name(cluster=T12 {"Power Supply Voltage"=13.0, "Min Avg Current"=0.0, "Max Avg Current"=0.0, "Min Run Time"=0.0, "Max Run Time"=0.0, "Min Speed"=0.0, "Max Speed"=0.0, "AP Data % of Threshold"=0.0, "Travel Distance"=0.0, "AP Data Type"=enum."91/61", "Check Current"=FALSE, "Check Run Time"=FALSE, "Check Speed"=FALSE, "Express Motion?"=FALSE, "Check Sound Test"=FALSE, "Check Position?"=FALSE, "Collect AP Data"=FALSE, "Inital Position"=0, "End Position"=0, "Goto Posiition"=0, "Max max Current"=0.0, "Min max Current"=0.0, "Check max Current"=FALSE, "Check Sound"=FALSE, "Min Sound (dB)"=0.0, "Max Sound (dB)"=0.0, "SW Mode"=enum."Hard Switch", "LIN Msg"={"ID"=0, "Msg"=[], "LDF"="EX1H"}} ("Motion Data Cluster"), "AP Data Type"=w2129, "Collect AP Data"=w2128, "Goto Posiition"=w2127, "Power Supply Voltage"=w2126) -> (w2131:T12)
            n695 = Select(t=All_Motions."Goto Position Glass" ("Current Motion"), s=w2135, f=All_Motions."Goto Position Sunshade" ("Current Motion")) -> (s? t:f=w2140:T3)
            n696 = Tick Count (ms)() -> (millisecond timer value=w2123:u32)
            n697 = Flatten To String(anything=w2131, error in (no error)=w2133) -> (data string=w2130:string, error out=w2132:errorcluster)  [unwired: 2 in, 1 out]
            n698 = Bundle By Name(cluster=w2143, "misc status.delay start time (ticks)"=w2123, "Motion Status.Motion"=w2140, "Sequence State.Step Data String"=w2130, "misc status.Serial Port Configured?"=w2135, "misc status.Real Rollo?"=w2124) -> (w2122:T1)
          }
          frame "Set Power Supply" {
            n699 = Scan From String(format string="%0.2f", input string=w2147, error in=w2145) -> (error out=w2144:errorcluster, output 1=w2146:dbl)  [unwired: 2 in, 2 out]
            n700 = Bundle By Name(cluster=w2150, "misc status.PS Voltage"=w2146) -> (w2151:T1)
          }
          frame "Sunshade Close" {
            n701 = Bundle By Name(cluster=w2156, "Motion Status.Motion"=All_Motions."Sunshade Close" ("Current Motion"), "Sequence State.Step Data String"=w2157, "misc status.Serial Port Configured?"=FALSE ("Glass Motor?")) -> (w2152:T1)
          }
          frame "Sunshade Close 2" {
            n702 = Bundle By Name(cluster=w2163, "Motion Status.Motion"=All_Motions."Sunshade Close 2" ("Current Motion"), "Sequence State.Step Data String"=w2164, "misc status.Serial Port Configured?"=FALSE ("Glass Motor?")) -> (w2159:T1)
          }
          frame "Sunshade Open" {
            n703 = Bundle By Name(cluster=w2170, "Motion Status.Motion"=All_Motions."Sunshade Open" ("Current Motion"), "Sequence State.Step Data String"=w2171, "misc status.Serial Port Configured?"=FALSE ("Glass Motor?")) -> (w2166:T1)
          }
          frame "Sunshade Open 2" {
            n704 = Bundle By Name(cluster=w2177, "Motion Status.Motion"=All_Motions."Sunshade Open 2" ("Current Motion"), "Sequence State.Step Data String"=w2178, "misc status.Serial Port Configured?"=FALSE ("Glass Motor?")) -> (w2173:T1)
          }
          frame "Sunshade DirectControl Teach" {
            w2180 = FALSE ("misc status.Serial Port Configured?")
            n705 = Bundle By Name(cluster=w2187, "Motion Status.Motion"=All_Motions."Sunshade Teach", "Sequence State.Step Data String"=w2183, "Sequence State.Step Description"=w2184, "misc status.Serial Port Configured?"=w2180, "Direct Control Info.TeachEvent"=w2180, "Direct Control Info.Derect control"=TRUE) -> (w2186:T1)
          }
          frame "Sunshade DirectControl FullOpen" {
            w2189 = FALSE ("misc status.Serial Port Configured?")
            n706 = Bundle By Name(cluster=w2196, "Motion Status.Motion"=All_Motions."Express Sunshade Open", "Sequence State.Step Data String"=w2192, "Sequence State.Step Description"=w2193, "misc status.Serial Port Configured?"=w2189, "Direct Control Info.TeachEvent"=w2189, "Direct Control Info.Derect control"=TRUE) -> (w2195:T1)
          }
          frame "Sunshade DirectControl FullClose" {
            w2198 = FALSE ("misc status.Serial Port Configured?")
            n707 = Bundle By Name(cluster=w2205, "Motion Status.Motion"=All_Motions."Express Sunshade Close", "Sequence State.Step Data String"=w2201, "Sequence State.Step Description"=w2202, "misc status.Serial Port Configured?"=w2198, "Direct Control Info.TeachEvent"=w2198, "Direct Control Info.Derect control"=TRUE) -> (w2204:T1)
          }
          frame "Sunshade DirectControl GotoPosition" {
            w2207 = FALSE ("misc status.Serial Port Configured?")
            n708 = Bundle By Name(cluster=w2214, "Motion Status.Motion"=All_Motions."Goto Position Sunshade", "Sequence State.Step Data String"=w2210, "Sequence State.Step Description"=w2211, "misc status.Serial Port Configured?"=w2207, "Direct Control Info.TeachEvent"=w2207, "Direct Control Info.Derect control"=TRUE) -> (w2213:T1)
          }
          frame Default {
            n709 = Bundle By Name(cluster=w2223, "Sequence State.Step Data String"=w2222, "Sequence State.Step Description"=w2218) -> (w2216:T1)
            n710 = Build Array(w2221, "Check Sequence") -> (w2220:string[])
          }
        }
      }
      frame "Get Sequences" {
        n711 = Unbundle By Name(w2227) -> ("misc status.Part Setup.Part Type"=w2224:string, "misc station config.Station Name"=w2248:string, "Sequence State"=w2233:T24, "Store Data.Error Table"=w2250:string[][], "paths.Base Path"=w2241:path)
        n712 = call "get path to lvdt presets.vi"("product"=w2224, "paths.Base Path"=w2241) -> ("path"=w2246:path)  [unwired: 9 in]
        n713 = call <vilib>:"Check if File or Folder Exists.vi"("error in (no error)"=w2244, "path"=w2246) -> ("error out"=w2243:errorcluster, "file or folder exists?"=w2242:bool, "dup path"=w2245:path)  [unwired: 7 in]
        n714 = disable-structure shown="禁用" {
          disable-tunnel: [w2261 _] -> w2228
          disable-tunnel: [w2260 _] -> w2247
          disable-tunnel: w2245 -> [w2259 _]
          disable-tunnel: w2243 -> [w2258 _]
          disable-tunnel: w2242 -> [w2257 _]
          disable-tunnel: w2224 -> [w2256 _]
          frame Disabled {
            n715 = case shown="真" w2257 {
              tunnel: w2259 -> [_ w2270]
              tunnel: w2256 -> [_ w2269]
              tunnel: w2258 -> [w2262 w2268]
              tunnel: [w2262 w2267] -> w2261
              tunnel: [_ w2266] -> w2260
              frame False {
              }
              frame True {
                n716 = call <vilib>:"Open Config Data.vi"("error in (no error)"=w2268, "configuration file path"=w2270) -> ("error out"=w2273:errorcluster, "refnum"=w2274:T68)  [unwired: 7 in, 1 out]
                n717 = call-poly <vilib>:"Read Key.vi"("section"="LVDT's Preset Data", "error in (no error)"=w2273, "key"=w2269, "refnum"=w2274) -> ("error out"=w2265:errorcluster, "value"=w2271:string, "refnum out"=w2263:T68)  [unwired: 4 in, 1 out]
                n718 = call <vilib>:"Close Config Data.vi"("error in (no error)"=w2265, "refnum"=w2263) -> ("error out"=w2264:errorcluster)  [unwired: 8 in, 1 out]
                n719 = Unflatten From String(type=T22[] [{"Upper Limit"=1.0, "Lower Limit"=-1.0, "LVDT Name"="LVDT 1", "Check"=FALSE}, {"Upper Limit"=1.0, "Lower Limit"=-1.0, "LVDT Name"="LVDT 2", "Check"=FALSE}, {"Upper Limit"=1.0, "Lower Limit"=-1.0, "LVDT Name"="LVDT 3", "Check"=FALSE}, {"Upper Limit"=1.0, "Lower Limit"=-1.0, "LVDT Name"="LVDT 4", "Check"=FALSE}, {"Upper Limit"=1.0, "Lower Limit"=-1.0, "LVDT Name"="LVDT 5", "Check"=FALSE}, {"Upper Limit"=1.0, "Lower Limit"=-1.0, "LVDT Name"="LVDT 6", "Check"=FALSE}, {"Upper Limit"=1.0, "Lower Limit"=-1.0, "LVDT Name"="LVDT 7", "Check"=FALSE}, {"Upper Limit"=1.0, "Lower Limit"=-1.0, "LVDT Name"="LVDT 8", "Check"=FALSE}, {"Upper Limit"=1.0, "Lower Limit"=-1.0, "LVDT Name"="LVDT 9", "Check"=FALSE}, {"Upper Limit"=1.0, "Lower Limit"=-1.0, "LVDT Name"="LVDT 10", "Check"=FALSE}, {"Upper Limit"=1.0, "Lower Limit"=-1.0, "LVDT Name"="LVDT 11", "Check"=FALSE}, {"Upper Limit"=1.0, "Lower Limit"=-1.0, "LVDT Name"="LVDT 12", "Check"=FALSE}, {"Upper Limit"=1.0, "Lower Limit"=-1.0, "LVDT Name"="LVDT 13", "Check"=FALSE}, {"Upper Limit"=1.0, "Lower Limit"=-1.0, "LVDT Name"="LVDT 14", "Check"=FALSE}] ("WK LVDT's Limit Array"), binary string=w2271, error in (no error)=w2264) -> (value=w2266:T22[], error out=w2267:errorcluster)  [unwired: 2 in, 1 out]
              }
            }
          }
          frame Enabled {
          }
        }
        n720 = call <vilib>:"Clear Errors.vi"("error in (no error)"=w2228) -> ("error out"=w2229:errorcluster)  [unwired: 5 in, 1 out]
        n721 = call "Get Part Information.vi"("Error"=w2229, "station name"=w2248, "Part Type"=w2224) -> ("Error Out"=w2225:errorcluster, "Part Setup"=w2252:T26, "Switch Value Configuration"=w2254:T4[], "Switch Configuration"=w2255:T2[], "Motor Drift Compensation"=w2226:i32[], "Seqence Info"=w2230:T25[], "Hall Positions"=w2240:i32[], "enable ps rem sense"=w2239:bool, "lvdt precision"=w2238:T23)
        n722 = Unbundle By Name(w2225) -> ("source"=w2251:string, "status"=w2235:bool)
        n723 = case shown="真" w2235 {
          tunnel: w2251 -> [_ w2277]
          tunnel: w2250 -> [w2276 w2280]
          tunnel: [w2276 w2279] -> w2249
          frame False {
          }
          frame True {
            n724 = call "EOL Error Table.vi"("Error Description"=w2277, "Error No."=u16 134, "Error Table In"=w2280) -> ("Error Table Out"=w2279:string[][])  [unwired: 7 in, 1 out]
          }
        }
        n725 = Not(x=w2235) -> (.not. x?=w2237:bool)
        n726 = call "pass fail action decision.vi"("Pass?"=w2237, "Sequence State in"=w2233, "event queue in"=w2236) -> ("Sequence State out"=w2232:T24, "Event queue out"=w2234:string[])  [unwired: 7 in]
        n727 = Bundle By Name(cluster=w2232, "Seqence"=w2230) -> (w2231:T24)
        n728 = Bundle By Name(cluster=w2227, "Switch Output Array"=w2255, "Switch Value Configuration"=w2254, "misc status.Part Setup"=w2252, "Sequence State"=w2231, "Store Data.Error Table"=w2249, "LVDT Status.LVDT's stored config"=w2247, "Direct Control Info.Hall Positions"=w2240, "Direct Control Info.Drift offsets"=w2226, "Motion Status.remote sense enabled"=w2239, "LVDT Status.lvdt precision"=w2238) -> (w2253:T1)
      }
      frame "Sequence Complete" {
        # "add this event \"reset switch outputs\" when the test abort"
        n729 = Unbundle By Name(w2297) -> ("ctl refs.all station status"=w2302:refnum<vi>, "NVH Operator?"=w2282:bool, "NVH Configuration.NVH Station?"=w2283:bool, "Sequence State.Pass?"=w2292:bool, "NVH Pass?"=w2291:bool, "Operator Pass?"=w2290:bool, "Store Data.Error Table"=w2288:string[][])  [unwired: 1 out]
        n730 = call "check NVH error.vi"("Error Table In"=w2288) -> ("NVH Error?"=w2284:bool, "have errror?"=w2287:bool)  [unwired: 9 in]
        n731 = Build Array(w2283, w2282, w2287, w2284) -> (w2285:bool[])
        n732 = Boolean Array To Number(Boolean array=w2285) -> (number=w2286:u32)
        n733 = case shown="0, 默认" w2286 {
          tunnel: [string[] ["Close Comm Port", "Turn Power Off", "Reset Switch Outputs", "Write Test Complete to PLC", "Update Error Table", "NVH End of Test IRQ", "Print 2D Barcode", "Write Errors to File", "Save Data", "Check Input"] ("event queue out") string[] ["write NVH result"] ("event queue out")] -> w2295
          tunnel: [FALSE ("NVH Operator?") FALSE ("NVH Operator?")] -> w2294
          tunnel: w2292 -> [w2314 w2324]
          tunnel: [w2310 w2325] -> w2293
          tunnel: w2291 -> [w2316 _]
          tunnel: w2290 -> [w2313 _]
          tunnel: [w2315 w2324] -> w2289
          tunnel: w2283 -> [w2312 _]
          tunnel: w2287 -> [w2311 _]
          tunnel: w2284 -> [w2309 w2326]
          frame 0, Default {
            n734 = case shown="假" w2312 {
              tunnel: w2316 -> [_ w2323]
              tunnel: w2313 -> [_ w2322]
              tunnel: [w2319 w2321] -> w2315
              tunnel: w2314 -> [w2319 _]
              tunnel: w2311 -> [_ w2320]
              frame False {
              }
              frame True {
                n735 = Compound Arithmetic op=AND(w2323, w2322, invert w2320) -> (w2321:bool)
              }
            }
            n736 = Not(x=w2309) -> (.not. x?=w2310:bool)
          }
          frame 3, 15 {
            n737 = Not(x=w2326) -> (.not. x?=w2325:bool)
          }
        }
        n738 = property class="Clust (严格)"(reference=w2302, error in=w2281) -> (reference out=w2306:refnum<vi>, error out=w2303:errorcluster, "Value"=w2304:T52)
        n739 = Get Date/Time String(date format (0)=enum16{"short", "long", "abbreviated"}."short") -> (date string=w2301:string, time string=w2300:string)  [unwired: 2 in]
        n740 = Bundle By Name(cluster=w2304, "Date"=w2301, "Time"=w2300) -> (w2305:T52)
        n741 = Bundle By Name(cluster=w2297, "Application Status"="Sequence Complete", "Sequence State.Testing?"=FALSE ("Cycling?"), "NVH Operator?"=w2294, "NVH Pass?"=w2293, "Sequence State.Pass?"=w2289) -> (w2308:T1)
        n742 = property class="Clust (严格)"(reference=w2306, error in=w2303, "Value"=w2305) -> (error out=w2296:errorcluster)  [unwired: 1 out]
      }
      frame "--------Manual--------" {
      }
      frame "Manual Control" {
        n743 = Unbundle By Name(w2334) -> ("Config Info"=w2335:T34)
        n744 = Unbundle By Name(w2334) -> ("Station Index"=w2337:i32, "ctl refs.exit program"=w2336:refnum<vi>)
        n745 = call "Config Info Get.vi"("Config Info"=w2335) -> ("PLC Comms"=w2333:T56)  [unwired: 7 in, 3 out]
        n746 = Unbundle By Name(w2333) -> ("PLC string read Tags.Model Type"=w2332:T40)
        n747 = case shown="默认" w2337 {
          selector: w2337 -> [w2342 _]
          tunnel: w2334 -> [w2343 w2356]
          tunnel: [w2343 w2355] -> w2338
          tunnel: w2332 -> [w2340 _]
          tunnel: w2336 -> [w2341 _]
          frame 10 {
            n748 = stacked-sequence {
              seq-local: ["VI路径" _ _] -> [_ _ w2352]
              tunnel: w2342 -> [_ w2350 _]
              tunnel: w2341 -> [_ w2349 _]
              tunnel: w2340 -> [_ w2348 _]
              frame #0 {
                w2345 = TRUE
                n749 = Open VI Reference(vi path="VI路径") -> (vi reference=w2346:refnum<vi>)  [unwired: 5 in, 1 out]
                n750 = property class="VI"(reference=w2346, "Exec.ShowFPOnCall"=w2345, "Exec.CloseFPAfterCall"=w2345) -> ()  [unwired: 1 in, 2 out]
              }
              frame #1 {
                n751 = call "plc read string.vi"("addr,tag"=w2348) -> ("Data"=w2347:string)  [unwired: 9 in, 1 out]
                n752 = call "MotorDirectControl.vi"("station index"=w2350, "Exit Refnum"=w2349, "PatrType"=w2347, "test mode"=TRUE) -> ()  [unwired: 12 in, 4 out]
              }
              frame #2 {
                w2353 = FALSE
                n753 = Open VI Reference(vi path=w2352) -> (vi reference=w2354:refnum<vi>)  [unwired: 5 in, 1 out]
                n754 = property class="VI"(reference=w2354, "Exec.ShowFPOnCall"=w2353, "Exec.CloseFPAfterCall"=w2353) -> ()  [unwired: 1 in, 2 out]
              }
            }
          }
          frame Default {
            n755 = call "EOL Manual Controls.vi"("main thread cluster"=w2356) -> ("main thread cluster out"=w2355:T1)  [unwired: 10 in]
          }
        }
      }
      frame "Manual control operator action" {
        n756 = Unbundle By Name(w2360) -> ("Config Info"=w2361:T34)
        n757 = Unbundle By Name(w2360) -> ("NVH Motion Steps"=w2376:string[], "ctl refs.all station status"=w2377:refnum<vi>, "D in map.Abort Test"=w2375:T17, "Station Index"=w2370:i32, "Direct Control Info.Hall Positions"=w2369:i32[], "Direct Control Info.teach pass"=w2366:bool, "Store Data.Error Table"=w2365:string[][])
        n758 = call "Config Info Get.vi"("Config Info"=w2361) -> ("PLC Comms"=w2359:T56)  [unwired: 7 in, 3 out]
        n759 = Unbundle By Name(w2359) -> ("PLC boolean read Tags"=w2358:T57, "PLC boolean read Tags.NVH Operator Check"=w2357:T40)
        n760 = property class="Clust (严格)"(reference=w2377) -> (reference out=w2381:refnum<vi>, error out=w2378:errorcluster, "Value"=w2379:T52)  [unwired: 1 in]
        n761 = call "plc write bool.vi"("value"=TRUE, "addr,tag"=w2357) -> ("error out"=w2364:errorcluster)  [unwired: 9 in]
        n762 = call "Manual control operator action.vi"("error in"=w2364, "Abort Test"=w2375, "Motion Steps in"=w2376, "input cluster"=w2358) -> ("error out"=w2362:errorcluster, "Step"=w2373:string, "data string"=w2367:string, "Motion Steps out"=w2368:string[])  [unwired: 4 in]
        n763 = case shown="真" w2366 {
          tunnel: w2360 -> [w2387 w2403]
          tunnel: w2373 -> [_ w2402]
          tunnel: [w2386 w2401] -> w2372
          tunnel: [string[] ["Check Sequence"] w2400] -> w2371
          tunnel: w2370 -> [_ w2399]
          tunnel: w2369 -> [_ w2398]
          tunnel: w2368 -> [_ w2393]
          tunnel: w2367 -> [_ w2395]
          tunnel: w2365 -> [w2388 _]
          tunnel: w2362 -> [_ _]
          tunnel: w2358 -> [_ w2392]
          frame False {
            n764 = call "EOL Error Table.vi"("Error Description"="You need to be teach First", "Error No."=u16 212, "Error Table In"=w2388) -> ("Error Table Out"=w2383:string[][])  [unwired: 7 in, 1 out]
            n765 = Bundle By Name(cluster=w2387, "Store Data.Error Table"=w2383, "Sequence State.Pass?"=FALSE) -> (w2386:T1)
          }
          frame True {
            w2394 = TRUE ("Sequence State.Testing?")
            n766 = Unbundle By Name(w2392) -> ("NVH Operator Express Rollo Open01"=w2391:T40, "NVH Operator Express Rollo Close01"=w2390:T40)
            n767 = Bundle By Name(cluster=w2403, "Motion Status.Motion"=All_Motions."Idle", "Sequence State.Testing?"=w2394, "NVH Motion Steps"=w2393, "manual control(direct)"=w2394) -> (w2396:T1)
            n768 = case shown="\"FullOpen\"" w2402 {
              tunnel: w2396 -> [w2408 w2416 w2427 w2440 w2444]
              tunnel: [w2404 w2415 w2426 w2439 w2444] -> w2401
              tunnel: w2395 -> [w2407 w2412 w2423 w2437 _]
              tunnel: [w2405 string[] ["Init Motion", "Direct control set switch output", "DirectControl"] ("event queue out") string[] ["Init Motion", "Direct control set switch output", "DirectControl"] ("event queue out") string[] ["Init Motion", "Direct control set switch output", "DirectControl"] ("event queue out") w2443] -> w2400
              tunnel: w2399 -> [_ _ _ _ _]
              tunnel: w2398 -> [_ w2409 w2420 w2434 _]
              tunnel: w2393 -> [_ _ _ _ w2443]
              tunnel: w2391 -> [_ _ w2418 w2431 _]
              tunnel: w2390 -> [_ _ w2417 w2432 _]
              frame Default {
                n769 = Bundle By Name(cluster=w2408, "Sequence State.Step Data String"=w2407) -> (w2404:T1)
                n770 = Build Array("Manual control operator action" ("element")) -> (w2405:string[])
              }
              frame "Teach" {
                w2410 = FALSE ("misc status.Serial Port Configured?")
                n771 = Bundle By Name(cluster=w2416, "Motion Status.Motion"=All_Motions."Sunshade Teach", "Sequence State.Step Data String"=w2412, "misc status.Serial Port Configured?"=w2410, "Direct Control Info.TeachEvent"=w2410, "Direct Control Info.Derect control"=TRUE, "Direct Control Info.set position"=w2409) -> (w2415:T1)
              }
              frame "FullOpen" {
                w2421 = FALSE ("misc status.Serial Port Configured?")
                n772 = call "ManualControlExitCheck.vi"("Stop Switch"=w2417, "Action Switch"=w2418) -> ("manual"=w2419:bool)  [unwired: 9 in]
                n773 = case shown="真" w2419 {
                  tunnel: [All_Motions."Express Sunshade Open" ("Motion Status.Motion") All_Motions."Sunshade Open" ("Motion Status.Motion")] -> w2425
                  frame False {
                  }
                  frame True {
                  }
                }
                n774 = Bundle By Name(cluster=w2427, "Motion Status.Motion"=w2425, "Sequence State.Step Data String"=w2423, "misc status.Serial Port Configured?"=w2421, "Direct Control Info.TeachEvent"=w2421, "Direct Control Info.Derect control"=TRUE, "Direct Control Info.set position"=w2420) -> (w2426:T1)
              }
              frame "FullClose" {
                w2435 = FALSE ("misc status.Serial Port Configured?")
                n775 = call "ManualControlExitCheck.vi"("Stop Switch"=w2431, "Action Switch"=w2432) -> ("manual"=w2430:bool)  [unwired: 9 in]
                n776 = case shown="真" w2430 {
                  tunnel: [All_Motions."Express Sunshade Close" ("Motion Status.Motion") All_Motions."Sunshade Close" ("Motion Status.Motion")] -> w2433
                  frame False {
                  }
                  frame True {
                  }
                }
                n777 = Bundle By Name(cluster=w2440, "Motion Status.Motion"=w2433, "Sequence State.Step Data String"=w2437, "misc status.Serial Port Configured?"=w2435, "Direct Control Info.TeachEvent"=w2435, "Direct Control Info.Derect control"=TRUE, "Direct Control Info.set position"=w2434) -> (w2439:T1)
              }
              frame "Reset Switch Outputs" {
              }
            }
          }
        }
        n778 = Bundle By Name(cluster=w2379, "Current Step Br"=w2373) -> (w2380:T52)
        n779 = property class="Clust (严格)"(reference=w2381, error in=w2378, "Value"=w2380) -> ()  [unwired: 2 out]
      }
      frame "direct manual action" {
        w2450 = TRUE ("Sequence State.Testing?")
        n780 = Unbundle By Name(w2448) -> ("Config Info"=w2449:T34)
        n781 = Unbundle By Name(w2448) -> ("NVH Motion Steps"=w2462:string[], "ctl refs.all station status"=w2463:refnum<vi>, "D in map.Abort Test"=w2461:T17)
        n782 = call "Config Info Get.vi"("Config Info"=w2449) -> ("PLC Comms"=w2447:T56)  [unwired: 7 in, 3 out]
        n783 = Unbundle By Name(w2447) -> ("PLC boolean read Tags"=w2445:T57, "PLC boolean read Tags.NVH Operator Check"=w2446:T40)
        n784 = call "plc write bool.vi"("value"=TRUE, "addr,tag"=w2446) -> ("error out"=w2454:errorcluster)  [unwired: 9 in]
        n785 = property class="Clust (严格)"(reference=w2463) -> (reference out=w2467:refnum<vi>, error out=w2464:errorcluster, "Value"=w2465:T52)  [unwired: 1 in]
        n786 = call "Manual control operator action.vi"("error in"=w2454, "Abort Test"=w2461, "Motion Steps in"=w2462, "input cluster"=w2445) -> ("Step"=w2459:string, "data string"=w2455:string, "Motion Steps out"=w2456:string[])  [unwired: 4 in, 1 out]
        n787 = Bundle By Name(cluster=w2465, "Current Step Br"=w2459) -> (w2466:T52)
        n788 = property class="Clust (严格)"(reference=w2467, error in=w2464, "Value"=w2466) -> ()  [unwired: 2 out]
        n789 = Bundle By Name(cluster=w2448, "Motion Status.Motion"=All_Motions."Idle", "Sequence State.Testing?"=w2450, "NVH Motion Steps"=w2456, "manual control(direct)"=w2450) -> (w2451:T1)
        n790 = case shown="\"FullOpen\"" w2459 {
          tunnel: w2451 -> [w2472 w2479 w2486 w2488]
          tunnel: [w2468 w2478 w2485 w2488] -> w2458
          tunnel: w2455 -> [w2471 w2476 w2483 _]
          tunnel: [w2469 string[] ["Init Motion", "Direct control set switch output", "DirectControl"] ("event queue out") string[] ["Init Motion", "Direct control set switch output", "DirectControl"] ("event queue out") w2487] -> w2457
          tunnel: w2456 -> [_ _ _ w2487]
          frame Default {
            n791 = Build Array("direct manual action" ("element")) -> (w2469:string[])
            n792 = Bundle By Name(cluster=w2472, "Sequence State.Step Data String"=w2471) -> (w2468:T1)
          }
          frame "FullOpen" {
            w2474 = FALSE ("misc status.Serial Port Configured?")
            n793 = Bundle By Name(cluster=w2479, "Motion Status.Motion"=All_Motions."Sunshade Open", "Sequence State.Step Data String"=w2476, "misc status.Serial Port Configured?"=w2474, "Direct Control Info.TeachEvent"=w2474, "Direct Control Info.Derect control"=TRUE) -> (w2478:T1)
          }
          frame "FullClose" {
            w2481 = FALSE ("misc status.Serial Port Configured?")
            n794 = Bundle By Name(cluster=w2486, "Motion Status.Motion"=All_Motions."Sunshade Close", "Sequence State.Step Data String"=w2483, "misc status.Serial Port Configured?"=w2481, "Direct Control Info.TeachEvent"=w2481, "Direct Control Info.Derect control"=TRUE) -> (w2485:T1)
          }
          frame "Reset Switch Outputs" {
          }
        }
      }
      frame "--------NVH--------" {
      }
      frame "NVH Check Echo" {
        n795 = Unbundle By Name(w2499) -> ("misc status.Part Setup.NVH Part Number"=w2494:u16, "Store Data.Error Table"=w2501:string[][], "NVH Configuration"=w2495:T6)
        n796 = call "EOL NVH Inputs Controls Buffer 2.0.vi"("NVH Configuration"=w2495) -> ("NVH_PartNumber_Echo"=w2493:u16)  [unwired: 6 in, 4 out]
        n797 = Equal?(x=w2494, y=w2493) -> (x = y?=w2492:bool)
        n798 = case shown="假" w2492 {
          tunnel: [string[] ["NVH Restart IRQ"] ("event queue out") w2510] -> w2502
          tunnel: [w2504 w2509] -> w2500
          tunnel: w2501 -> [w2505 w2508]
          tunnel: w2495 -> [_ w2507]
          frame False {
            n799 = call "EOL Error Table.vi"("Error No."=u16 33, "Error Table In"=w2505) -> ("Error Table Out"=w2504:string[][])  [unwired: 8 in, 1 out]
          }
          frame True {
            n800 = while {
              tunnel: [w2520] -> w2511
              tunnel: w2507 -> [w2518]
              i -> [w2526]
              stop <- w2522 stop-if-true
              w2521 = T61[] [enum."Online"] items=["Online", "Pass", "Fail", "Testing", "Ready for Model", "Error Bit 1", "Error Bit 2", "Error Bit 3", "Failure Bit 1", "Failure Bit 2", "Failure Bit 3", "Failure Bit 4", "Echo Bit 1", "Echo Bit 2", "Echo Bit 3", "Echo Bit 4", "Serial Number Read Ok", "Ready for Serrial Number"] ("Digital Inputs Array")
              # "This should be ready for serial number"
              n801 = Wait (ms)(milliseconds to wait=u32 100) -> ()  [unwired: 1 out]
              n802 = call "EOL NVH Inputs Controls Buffer 2.0.vi"("NVH Configuration"=w2518, "NVHK Inputs Control"=w2521, "Mode"=NVH_Mode_Control_2.0."Read") -> ("NVH Single Input"=w2520:bool)  [unwired: 4 in, 4 out]
              n803 = Greater Or Equal?(x=w2526, y=10) -> (x >= y?=w2523:bool)
              n804 = Or(x=w2520, y=w2523) -> (x .or. y?=w2522:bool)
            }
            n805 = case shown="真" w2511 {
              tunnel: [string[] ["NVH Restart IRQ"] ("event queue out") string[] ["NVH Send Serial Number"] ("event queue out")] -> w2510
              tunnel: [w2512 w2516] -> w2509
              tunnel: w2508 -> [w2514 w2516]
              frame False {
                n806 = call "EOL Error Table.vi"("Error No."=u16 32, "Error Table In"=w2514) -> ("Error Table Out"=w2512:string[][])  [unwired: 8 in, 1 out]
              }
              frame True {
              }
            }
          }
        }
        n807 = Bundle By Name(cluster=w2499, "Store Data.Error Table"=w2500) -> (w2496:T1)
        n808 = call "Insert Multiple Events.vi"("Events to Insert"=w2502, "Event queue in"=w2498) -> ("Event queue out"=w2497:string[])  [unwired: 2 in, 3 out]
      }
      frame "NVH Check Error" {
        w2542 = T61[] [enum."Pass", enum."Fail"] items=["Online", "Pass", "Fail", "Testing", "Ready for Model", "Error Bit 1", "Error Bit 2", "Error Bit 3", "Failure Bit 1", "Failure Bit 2", "Failure Bit 3", "Failure Bit 4", "Echo Bit 1", "Echo Bit 2", "Echo Bit 3", "Echo Bit 4", "Serial Number Read Ok", "Ready for Serrial Number"] ("Digital Inputs Array")
        # "1) Reset the Stop Bit\n2) Check if there is an failure. If there are then \n     report the failure\n3) Check if there are any errors with the system (This needs to be added in later"
        n809 = Unbundle By Name(w2548) -> ("Motion Status.Motion"=w2550:T3, "Store Data.Error Table"=w2552:string[][], "Sequence State"=w2534:T24, "Store Data.Motion Data Array"=w2529:T11[], "NVH Configuration"=w2546:T6)
        n810 = Array Size(array=w2529) -> (size(s)=w2532:i32)
        n811 = Decrement(x=w2532) -> (x-1=w2531:i32)
        n812 = Index Array(array=w2529, index=w2531) -> (element=w2530:T11)
        n813 = Unbundle By Name(w2530) -> ("Motion Data Limits.Check Sound Test"=w2528:bool)
        n814 = Format Into String(initial string=" - ", w2550) -> (resulting string=w2543:string)  [unwired: 2 in, 1 out]
        n815 = call "EOL NVH Inputs Controls Buffer 2.0.vi"("NVH Configuration"=w2546, "NVHK Inputs Control"=w2542) -> ("Error out"=w2538:string[][], "NVH Inputs Out"=w2545:bool[])  [unwired: 5 in, 3 out]
        n816 = Boolean Array To Number(Boolean array=w2545) -> (number=w2544:u32)
        n817 = stacked-sequence {
          tunnel: w2552 -> [_ w2563]
          tunnel: w2544 -> [_ w2562]
          tunnel: [_ w2561] -> w2551
          tunnel: [_ w2560] -> w2537
          tunnel: w2543 -> [_ w2559]
          tunnel: w2528 -> [_ w2558]
          tunnel: w2538 -> [_ w2557]
          tunnel: w2546 -> [w2553 _]
          frame #0 {
            w2555 = T69[] [enum."Stop Test"] items=["Restart IRQ", "Abort Test IRQ", "Read Model", "Start Test", "Stop Test", "End of Test IRQ", "Test Bit 1", "Test Bit 2", "Test Bit 3", "Test Bit 4", "Model Bit 1", "Model Bit 2", "Model Bit 3", "Model Bit 4", "Manual Restart IRQ"] ("B&K Outputs Control")
            n818 = call "EOL NVH Outputs Controls Buffer 2.0.vi"("Mode"=NVH_Mode_Control_2.0."Write", "NVH Outputs Control"=w2555, "NVH Configuration"=w2553, "NVH Outputs"=bool[] [FALSE]) -> ()  [unwired: 6 in, 6 out]
          }
          frame #1 {
            n819 = case shown="2" w2562 {
              tunnel: w2563 -> [w2565 w2569]
              tunnel: [w2565 w2568] -> w2561
              tunnel: [TRUE w2567] -> w2560
              tunnel: w2559 -> [_ _]
              tunnel: w2558 -> [_ w2572]
              tunnel: w2557 -> [_ w2566]
              frame 0, Default {
              }
              frame 2 {
                n820 = Select(t=FALSE ("Pass/Fail"), s=w2572, f=TRUE) -> (s? t:f=w2567:bool)
                n821 = Build Array (concatenate)(w2569, w2566) -> (w2568:string[][])
              }
            }
          }
        }
        n822 = call "pass fail action decision.vi"("fail behavior"=failure_behaviors."stop at next 'check sequence' if not rabbit", "Pass?"=w2537, "Sequence State in"=w2534, "event queue in"=w2536) -> ("Sequence State out"=w2533:T24, "Event queue out"=w2535:string[])  [unwired: 6 in]
        n823 = Select(t=Pass_Fail_Control."Pass" ("Position Test"), s=w2537, f=Pass_Fail_Control."Fail" ("Position Test")) -> (s? t:f=w2549:T21)
        n824 = Bundle By Name(cluster=w2548, "Sequence State"=w2533, "Store Data.Error Table"=w2551, "Motion Status.Noise Test"=w2549) -> (w2547:T1)
      }
      frame "NVH Check Ready for Model" {
        n825 = Unbundle By Name(w2578) -> ("Store Data.Error Table"=w2581:string[][], "NVH Configuration"=w2574:T6)
        n826 = while {
          tunnel: [w2592] -> w2573
          tunnel: w2574 -> [w2588]
          i -> [w2596]
          stop <- w2593 stop-if-true
          (unwired) 50 ("100MS IERATIONS FOR READY FOR MODEL")
          w2591 = T61[] [enum."Online", enum."Ready for Model"] items=["Online", "Pass", "Fail", "Testing", "Ready for Model", "Error Bit 1", "Error Bit 2", "Error Bit 3", "Failure Bit 1", "Failure Bit 2", "Failure Bit 3", "Failure Bit 4", "Echo Bit 1", "Echo Bit 2", "Echo Bit 3", "Echo Bit 4", "Serial Number Read Ok", "Ready for Serrial Number"] ("Digital Inputs Array")
          n827 = Wait (ms)(milliseconds to wait=u32 100) -> ()  [unwired: 1 out]
          n828 = call "EOL NVH Inputs Controls Buffer 2.0.vi"("NVH Configuration"=w2588, "NVHK Inputs Control"=w2591, "Mode"=NVH_Mode_Control_2.0."Read") -> ("NVH Inputs Out"=w2590:bool[])  [unwired: 4 in, 4 out]
          n829 = Greater Or Equal?(x=w2596, y=30 ("100MS IERATIONS FOR READY FOR MODEL")) -> (x >= y?=w2594:bool)
          n830 = And Array Elements(Boolean array=w2590) -> (logical AND=w2592:bool)
          n831 = Or(x=w2592, y=w2594) -> (x .or. y?=w2593:bool)
        }
        n832 = case shown="真" w2573 {
          tunnel: [string[] ["NVH Restart IRQ"] ("event queue out") string[] ["NVH Send Model Bits"] ("event queue out")] -> w2579
          tunnel: w2581 -> [w2584 w2586]
          tunnel: [w2582 w2586] -> w2580
          frame False {
            n833 = call "EOL Error Table.vi"("Error No."=u16 35, "Error Table In"=w2584) -> ("Error Table Out"=w2582:string[][])  [unwired: 8 in, 1 out]
          }
          frame True {
          }
        }
        n834 = Bundle By Name(cluster=w2578, "Store Data.Error Table"=w2580) -> (w2577:T1)
        n835 = call "Insert Multiple Events.vi"("Events to Insert"=w2579, "Event queue in"=w2576) -> ("Event queue out"=w2575:string[])  [unwired: 2 in, 3 out]
      }
      frame "NVH End of Test IRQ" {
        n836 = Unbundle By Name(w2602) -> ("Sequence State.NVH Status.NVH Test Running?"=w2605:bool, "NVH Configuration.NVH Station?"=w2599:bool, "NVH Configuration"=w2598:T6)
        n837 = Compound Arithmetic op=AND(w2605, w2599) -> (w2604:bool)
        n838 = case shown="真" w2604 {
          tunnel: w2598 -> [_ w2606]
          frame False {
          }
          frame True {
            n839 = stacked-sequence "This Sequence is to send the End of Test IRQ" {
              tunnel: w2606 -> [w2607 w2610 w2614 w2624]
              frame #0 {
                n840 = call "EOL NVH Outputs Controls Buffer 2.0.vi"("Mode"=NVH_Mode_Control_2.0."Write String", "NVH Configuration"=w2607, "Serial Number In"="") -> ()  [unwired: 7 in, 6 out]
              }
              frame #1 {
                w2612 = T69[] [enum."End of Test IRQ"] items=["Restart IRQ", "Abort Test IRQ", "Read Model", "Start Test", "Stop Test", "End of Test IRQ", "Test Bit 1", "Test Bit 2", "Test Bit 3", "Test Bit 4", "Model Bit 1", "Model Bit 2", "Model Bit 3", "Model Bit 4", "Manual Restart IRQ"] ("B&K Outputs Control")
                n841 = call "EOL NVH Outputs Controls Buffer 2.0.vi"("Mode"=NVH_Mode_Control_2.0."Write", "NVH Outputs Control"=w2612, "NVH Configuration"=w2610, "NVH Outputs"=bool[] [TRUE]) -> ()  [unwired: 6 in, 6 out]
              }
              frame #2 {
                n842 = while {
                  tunnel: [w2616] -> _
                  tunnel: w2614 -> [w2615]
                  i -> [w2622]
                  stop <- w2619 stop-if-true
                  w2618 = T61[] [enum."Online"] items=["Online", "Pass", "Fail", "Testing", "Ready for Model", "Error Bit 1", "Error Bit 2", "Error Bit 3", "Failure Bit 1", "Failure Bit 2", "Failure Bit 3", "Failure Bit 4", "Echo Bit 1", "Echo Bit 2", "Echo Bit 3", "Echo Bit 4", "Serial Number Read Ok", "Ready for Serrial Number"] ("Digital Inputs Array")
                  n843 = Wait (ms)(milliseconds to wait=u32 100) -> ()  [unwired: 1 out]
                  n844 = Greater Or Equal?(x=w2622, y=100 ("100MS IERATIONS FOR READY FOR MODEL")) -> (x >= y?=w2620:bool)
                  n845 = call "EOL NVH Inputs Controls Buffer 2.0.vi"("NVH Configuration"=w2615, "NVHK Inputs Control"=w2618, "Mode"=NVH_Mode_Control_2.0."Read") -> ("NVH Single Input"=w2616:bool)  [unwired: 4 in, 4 out]
                  n846 = Or(x=w2616, y=w2620) -> (x .or. y?=w2619:bool)
                }
              }
              frame #3 {
                w2626 = T69[] [enum."End of Test IRQ"] items=["Restart IRQ", "Abort Test IRQ", "Read Model", "Start Test", "Stop Test", "End of Test IRQ", "Test Bit 1", "Test Bit 2", "Test Bit 3", "Test Bit 4", "Model Bit 1", "Model Bit 2", "Model Bit 3", "Model Bit 4", "Manual Restart IRQ"] ("B&K Outputs Control")
                n847 = call "EOL NVH Outputs Controls Buffer 2.0.vi"("Mode"=NVH_Mode_Control_2.0."Write", "NVH Outputs Control"=w2626, "NVH Configuration"=w2624, "NVH Outputs"=bool[] [FALSE]) -> ()  [unwired: 6 in, 6 out]
              }
            }
          }
        }
        n848 = Bundle By Name(cluster=w2602, "Sequence State.NVH Status.NVH Test Running?"=FALSE ("B&K Test Aborted?")) -> (w2601:T1)
      }
      frame "NVH Restart IRQ" {
        w2636 = T69[] [enum."Restart IRQ", enum."Abort Test IRQ", enum."Read Model", enum."Start Test", enum."Stop Test", enum."End of Test IRQ", enum."Test Bit 1", enum."Test Bit 2", enum."Test Bit 3", enum."Test Bit 4"] items=["Restart IRQ", "Abort Test IRQ", "Read Model", "Start Test", "Stop Test", "End of Test IRQ", "Test Bit 1", "Test Bit 2", "Test Bit 3", "Test Bit 4", "Model Bit 1", "Model Bit 2", "Model Bit 3", "Model Bit 4", "Manual Restart IRQ"] ("B&K Outputs Control")
        # "WE ARE SETTING MODEL BITS AND READY FOR MODEL AND THEN IRQ IS HAPPENING, SO NVH\nGOES BACK TO WIATING For READY FOR MODEL WHILE WE MOVE ON TO SENDING SERIAL NUMBER"
        # "IF THESE ARE STILL TRUE AFTER SENDING IRQ, WE HAVE RACE CONDITION.\nonline\nready for module\n\nWE NEED AN ACK THAT IRQ WAS RECEIVED."
        # "eol sends restart\nnvh restarting to be ready for model, but not ready when eol checks,\n   so eol sets restart bit agian, but at this time, nvh has just finished being\n    ready for model  (so it is waiting for model info, and not checking restart irq)"
        # "Check whether the Restart IRQ\nCounter is exceeded if not try\none more time to check the\nNVH System"
        n849 = Unbundle By Name(w2643) -> ("Sequence State.NVH Status.Restart IRQ Counter"=w2645:u8, "Sequence State"=w2644:T24, "NVH Configuration"=w2642:T6)
        n850 = Array Size(array=w2636) -> (size(s)=w2635:i32)
        n851 = Initialize Array(FALSE, w2635) -> (w2633:bool[])
        n852 = Greater Or Equal?(x=w2645, y=u8 2) -> (x >= y?=w2640:bool)
        n853 = Increment(x=w2645) -> (x+1=w2628:u8)
        n854 = call "EOL NVH Outputs Controls Buffer 2.0.vi"("Mode"=NVH_Mode_Control_2.0."Write", "NVH Outputs Control"=w2636, "NVH Configuration"=w2642, "NVH Outputs"=w2633) -> ("Serial Number Out"=w2638:string)  [unwired: 6 in, 5 out]
        n855 = case shown="假" w2640 {
          tunnel: w2644 -> [w2650 w2664]
          tunnel: [w2650 w2663] -> w2639
          tunnel: w2638 -> [_ _]
          tunnel: w2642 -> [w2649 _]
          tunnel: w2632 -> [w2647 w2662]
          tunnel: [w2646 w2661] -> w2631
          frame False {
            n856 = stacked-sequence "This Sequence is to send the Restart IRQ" {
              tunnel: w2649 -> [w2651 _ w2656 _]
              frame #0 {
                w2653 = T69[] [enum."Restart IRQ"] items=["Restart IRQ", "Abort Test IRQ", "Read Model", "Start Test", "Stop Test", "End of Test IRQ", "Test Bit 1", "Test Bit 2", "Test Bit 3", "Test Bit 4", "Model Bit 1", "Model Bit 2", "Model Bit 3", "Model Bit 4", "Manual Restart IRQ"] ("B&K Outputs Control")
                n857 = call "EOL NVH Outputs Controls Buffer 2.0.vi"("Mode"=NVH_Mode_Control_2.0."Write", "NVH Outputs Control"=w2653, "NVH Configuration"=w2651, "NVH Outputs"=bool[] [TRUE]) -> ()  [unwired: 6 in, 6 out]
              }
              frame #1 {
                n858 = Wait (ms)(milliseconds to wait=u32 300 ("milliseconds to wait IRQ")) -> ()  [unwired: 1 out]
              }
              frame #2 {
                w2658 = T69[] [enum."Restart IRQ"] items=["Restart IRQ", "Abort Test IRQ", "Read Model", "Start Test", "Stop Test", "End of Test IRQ", "Test Bit 1", "Test Bit 2", "Test Bit 3", "Test Bit 4", "Model Bit 1", "Model Bit 2", "Model Bit 3", "Model Bit 4", "Manual Restart IRQ"] ("B&K Outputs Control")
                n859 = call "EOL NVH Outputs Controls Buffer 2.0.vi"("Mode"=NVH_Mode_Control_2.0."Write", "NVH Outputs Control"=w2658, "NVH Configuration"=w2656, "NVH Outputs"=bool[] [FALSE]) -> ()  [unwired: 6 in, 6 out]
              }
              frame #3 {
                # "***temporarily added delay until\nwe decide on an ack"
                n860 = Wait (ms)(milliseconds to wait=u32 500) -> ()  [unwired: 1 out]
              }
            }
            n861 = call "Insert Multiple Events.vi"("Events to Insert"=string[] ["NVH Check Ready for Model"] ("event queue out"), "Event queue in"=w2647) -> ("Event queue out"=w2646:string[])  [unwired: 2 in, 3 out]
          }
          frame True {
            n862 = call "pass fail action decision.vi"("Pass?"=FALSE ("Pass/Fail"), "Sequence State in"=w2664, "event queue in"=w2662) -> ("Sequence State out"=w2663:T24, "Event queue out"=w2661:string[])  [unwired: 7 in]
          }
        }
        n863 = Bundle By Name(cluster=w2643, "Sequence State"=w2639) -> (w2630:T1)
        n864 = Bundle By Name(cluster=w2630, "Sequence State.NVH Status.Restart IRQ Counter"=w2628) -> (w2629:T1)
      }
      frame "NVH Send Model Bits" {
        # "1) Send the model information\n2) Wait untill it is read\n3) Send the bit to read the model information\n4) Wait until the model read bit is read"
        n865 = Unbundle By Name(w2672) -> ("Store Data.Error Table"=w2673:string[][], "misc status.Part Setup.NVH Part Number"=w2674:u16, "NVH Configuration"=w2668:T6)
        n866 = stacked-sequence {
          tunnel: w2674 -> [w2676 _ _ _ _ _]
          tunnel: w2673 -> [_ _ _ _ w2691 _]
          tunnel: [_ _ _ _ w2690 _] -> w2667
          tunnel: [_ _ _ _ w2689 _] -> w2666
          tunnel: w2668 -> [w2675 _ w2682 _ w2687 w2707]
          frame #0 {
            w2679 = T69[] [enum."Model Bit 1", enum."Model Bit 2", enum."Model Bit 3", enum."Model Bit 4"] items=["Restart IRQ", "Abort Test IRQ", "Read Model", "Start Test", "Stop Test", "End of Test IRQ", "Test Bit 1", "Test Bit 2", "Test Bit 3", "Test Bit 4", "Model Bit 1", "Model Bit 2", "Model Bit 3", "Model Bit 4", "Manual Restart IRQ"] ("B&K Outputs Control")
            n867 = Number To Boolean Array(number=w2676) -> (Boolean array=w2678:bool[])
            n868 = call "EOL NVH Outputs Controls Buffer 2.0.vi"("Mode"=NVH_Mode_Control_2.0."Write", "Part Number"=w2676, "NVH Outputs Control"=w2679, "NVH Configuration"=w2675, "NVH Outputs"=w2678) -> ()  [unwired: 5 in, 6 out]
            n869 = call "EOL NVH Outputs Controls Buffer 2.0.vi"("Mode"=NVH_Mode_Control_2.0."Write Part Number", "Part Number"=w2676, "NVH Configuration"=w2675) -> ()  [unwired: 7 in, 6 out]
          }
          frame #1 {
            n870 = Wait (ms)(milliseconds to wait=u32 100) -> ()  [unwired: 1 out]
          }
          frame #2 {
            w2684 = T69[] [enum."Read Model"] items=["Restart IRQ", "Abort Test IRQ", "Read Model", "Start Test", "Stop Test", "End of Test IRQ", "Test Bit 1", "Test Bit 2", "Test Bit 3", "Test Bit 4", "Model Bit 1", "Model Bit 2", "Model Bit 3", "Model Bit 4", "Manual Restart IRQ"] ("B&K Outputs Control")
            n871 = call "EOL NVH Outputs Controls Buffer 2.0.vi"("Mode"=NVH_Mode_Control_2.0."Write", "NVH Outputs Control"=w2684, "NVH Configuration"=w2682, "NVH Outputs"=bool[] [TRUE]) -> ()  [unwired: 6 in, 6 out]
          }
          frame #3 {
            n872 = Wait (ms)(milliseconds to wait=u32 600 ("READ MODEL BIT DELAY")) -> ()  [unwired: 1 out]
          }
          frame #4 {
            # "This loop is stopped when online bit is high. Online bit is\nhigh when the NVH system is done reading the model \ninformation."
            n873 = while {
              tunnel: [w2700] -> w2688
              tunnel: w2687 -> [w2698]
              i -> [w2705]
              stop <- w2702 stop-if-true
              w2706 = T61[] [enum."Online"] items=["Online", "Pass", "Fail", "Testing", "Ready for Model", "Error Bit 1", "Error Bit 2", "Error Bit 3", "Failure Bit 1", "Failure Bit 2", "Failure Bit 3", "Failure Bit 4", "Echo Bit 1", "Echo Bit 2", "Echo Bit 3", "Echo Bit 4", "Serial Number Read Ok", "Ready for Serrial Number"] ("Digital Inputs Array")
              n874 = Wait (ms)(milliseconds to wait=u32 500 ("READ MODEL BIT DELAY")) -> ()  [unwired: 1 out]
              n875 = Greater?(x=w2705, y=50) -> (0:w2701:bool)
              n876 = call "EOL NVH Inputs Controls Buffer 2.0.vi"("NVH Configuration"=w2698, "NVHK Inputs Control"=w2706, "Mode"=NVH_Mode_Control_2.0."Read") -> ("NVH Single Input"=w2700:bool)  [unwired: 4 in, 4 out]
              n877 = Or(x=w2700, y=w2701) -> (x .or. y?=w2702:bool)
            }
            n878 = case shown="假" w2688 {
              tunnel: [string[] ["NVH Restart IRQ"] ("event queue out") string[] ["NVH Check Echo"] ("event queue out")] -> w2689
              tunnel: w2691 -> [w2694 w2697]
              tunnel: [w2692 w2697] -> w2690
              frame False {
                n879 = call "EOL Error Table.vi"("Error No."=u16 36, "Error Table In"=w2694) -> ("Error Table Out"=w2692:string[][])  [unwired: 8 in, 1 out]
              }
              frame True {
              }
            }
          }
          frame #5 {
            w2709 = T69[] [enum."Read Model"] items=["Restart IRQ", "Abort Test IRQ", "Read Model", "Start Test", "Stop Test", "End of Test IRQ", "Test Bit 1", "Test Bit 2", "Test Bit 3", "Test Bit 4", "Model Bit 1", "Model Bit 2", "Model Bit 3", "Model Bit 4", "Manual Restart IRQ"] ("B&K Outputs Control")
            n880 = call "EOL NVH Outputs Controls Buffer 2.0.vi"("Mode"=NVH_Mode_Control_2.0."Write", "NVH Outputs Control"=w2709, "NVH Configuration"=w2707, "NVH Outputs"=bool[] [FALSE]) -> ()  [unwired: 6 in, 6 out]
          }
        }
        n881 = Bundle By Name(cluster=w2672, "Store Data.Error Table"=w2667) -> (w2669:T1)
        n882 = call "Insert Multiple Events.vi"("Events to Insert"=w2666, "Event queue in"=w2671) -> ("Event queue out"=w2670:string[])  [unwired: 2 in, 3 out]
      }
      frame "NVH Send Serial Number" {
        # "1) Write the string\n2) Check the Acknowledge for serial number read. If it is ok go to\n    next step to read the echo else go to restart the NVH System."
        n883 = Unbundle By Name(w2716) -> ("Store Data.Error Table"=w2719:string[][], "Store Data.Module Info.Serial Number"=w2720:string, "NVH Configuration"=w2714:T6)
        n884 = while {
          tunnel: w2720 -> [w2734]
          tunnel: [w2728] -> w2711
          tunnel: w2714 -> [w2727]
          i -> [w2732]
          stop <- w2729 stop-if-true
          n885 = stacked-sequence {
            tunnel: w2734 -> [w2736 _ _]
            tunnel: [_ w2739 _] -> w2731
            tunnel: [_ w2739 _] -> w2728
            tunnel: w2727 -> [w2735 w2738 w2749]
            frame #0 {
              n886 = call "EOL NVH Outputs Controls Buffer 2.0.vi"("Mode"=NVH_Mode_Control_2.0."Write String", "NVH Configuration"=w2735, "Serial Number In"=w2736) -> ()  [unwired: 7 in, 6 out]
            }
            frame #1 {
              n887 = while {
                tunnel: [w2742] -> w2739
                tunnel: w2738 -> [w2740]
                i -> [w2746]
                stop <- w2745 stop-if-true
                w2743 = T61[] [enum."Serial Number Read Ok"] items=["Online", "Pass", "Fail", "Testing", "Ready for Model", "Error Bit 1", "Error Bit 2", "Error Bit 3", "Failure Bit 1", "Failure Bit 2", "Failure Bit 3", "Failure Bit 4", "Echo Bit 1", "Echo Bit 2", "Echo Bit 3", "Echo Bit 4", "Serial Number Read Ok", "Ready for Serrial Number"] ("Digital Inputs Array")
                n888 = Wait (ms)(milliseconds to wait=100) -> ()  [unwired: 1 out]
                n889 = Greater Or Equal?(x=w2746, y=50) -> (x >= y?=w2747:bool)
                n890 = call "EOL NVH Inputs Controls Buffer 2.0.vi"("NVH Configuration"=w2740, "NVHK Inputs Control"=w2743, "Mode"=NVH_Mode_Control_2.0."Read") -> ("NVH Single Input"=w2742:bool)  [unwired: 4 in, 4 out]
                n891 = Or(x=w2742, y=w2747) -> (x .or. y?=w2745:bool)
              }
            }
            frame #2 {
              n892 = call "EOL NVH Outputs Controls Buffer 2.0.vi"("Mode"=NVH_Mode_Control_2.0."Write String", "NVH Configuration"=w2749, "Serial Number In"="") -> ()  [unwired: 7 in, 6 out]
            }
          }
          n893 = Greater Or Equal?(x=w2732, y=5) -> (x >= y?=w2730:bool)
          n894 = Or(x=w2731, y=w2730) -> (x .or. y?=w2729:bool)
        }
        n895 = case shown="假" w2711 {
          tunnel: [string[] ["NVH Restart IRQ"] ("event queue out") string[] [] ("event queue out")] -> w2712
          tunnel: w2719 -> [w2723 w2726]
          tunnel: [w2722 w2726] -> w2713
          frame False {
            n896 = call "EOL Error Table.vi"("Error No."=u16 37, "Error Table In"=w2723) -> ("Error Table Out"=w2722:string[][])  [unwired: 8 in, 1 out]
          }
          frame True {
          }
        }
        n897 = Bundle By Name(cluster=w2716, "Store Data.Error Table"=w2713) -> (w2715:T1)
        n898 = call "Insert Multiple Events.vi"("Events to Insert"=w2712, "Event queue in"=w2717) -> ("Event queue out"=w2718:string[])  [unwired: 2 in, 3 out]
      }
      frame "NVH Start Test" {
        n899 = Unbundle By Name(w2756) -> ("Sequence State"=w2760:T24, "Store Data.Error Table"=w2761:string[][], "Motion Status.Motion"=w2762:T3, "NVH Configuration.NVH Station?"=w2755:bool, "NVH Configuration"=w2754:T6)
        n900 = case shown="真" w2755 {
          tunnel: w2762 -> [_ w2774]
          tunnel: [w2763 w2773] -> w2752
          tunnel: w2761 -> [w2764 w2772]
          tunnel: w2760 -> [w2765 w2771]
          tunnel: [w2765 w2770] -> w2759
          tunnel: [w2764 w2769] -> w2758
          tunnel: w2754 -> [_ w2767]
          tunnel: w2753 -> [w2763 w2766]
          frame False {
          }
          frame True {
            # "1) Send the start test bit\n3) Check whether the \"Testing\" bit is high.\n    Check untill it is true or timer expires.\n4) Rest the start test bit"
            n901 = stacked-sequence {
              tunnel: w2774 -> [w2792 _ _]
              tunnel: [_ _ w2810] -> w2768
              tunnel: w2767 -> [w2790 w2805 w2809]
              frame #0 {
                w2794 = T69[] [enum."Test Bit 1", enum."Test Bit 2", enum."Test Bit 3", enum."Test Bit 4"] items=["Restart IRQ", "Abort Test IRQ", "Read Model", "Start Test", "Stop Test", "End of Test IRQ", "Test Bit 1", "Test Bit 2", "Test Bit 3", "Test Bit 4", "Model Bit 1", "Model Bit 2", "Model Bit 3", "Model Bit 4", "Manual Restart IRQ"] ("B&K Outputs Control")
                n902 = case shown="\"Idle\", 默认" w2792 {
                  tunnel: [u16 1 u16 2 u16 3 u16 4 u16 5 u16 6 u16 0 u16 7 u16 8] -> w2791
                  frame "Glass Slide Open", "Express Glass Slide Open" {
                  }
                  frame "Glass Slide Close", "Express Glass Slide Close" {
                  }
                  frame "Glass Vent Open", "Express Glass Vent Open" {
                  }
                  frame "Glass Vent Close", "Express Glass Vent Close" {
                  }
                  frame "Sunshade Open", "Express Sunshade Open" {
                  }
                  frame "Sunshade Close", "Express Sunshade Close" {
                  }
                  frame "Idle", Default {
                  }
                  frame "Sunshade Open 2", "Express Sunshade Open 2" {
                  }
                  frame "Sunshade Close 2", "Express Sunshade Close 2" {
                  }
                }
                n903 = Number To Boolean Array(number=w2791) -> (Boolean array=w2793:bool[])
                n904 = call "EOL NVH Outputs Controls Buffer 2.0.vi"("Mode"=NVH_Mode_Control_2.0."Write", "Motion Number"=w2791, "NVH Outputs Control"=w2794, "NVH Configuration"=w2790, "NVH Outputs"=w2793) -> ()  [unwired: 5 in, 6 out]
              }
              frame #1 {
                w2807 = T69[] [enum."Start Test", enum."Stop Test"] items=["Restart IRQ", "Abort Test IRQ", "Read Model", "Start Test", "Stop Test", "End of Test IRQ", "Test Bit 1", "Test Bit 2", "Test Bit 3", "Test Bit 4", "Model Bit 1", "Model Bit 2", "Model Bit 3", "Model Bit 4", "Manual Restart IRQ"] ("B&K Outputs Control")
                n905 = call "EOL NVH Outputs Controls Buffer 2.0.vi"("Mode"=NVH_Mode_Control_2.0."Write", "NVH Outputs Control"=w2807, "NVH Configuration"=w2805, "NVH Outputs"=bool[] [TRUE, FALSE]) -> ()  [unwired: 6 in, 6 out]
              }
              frame #2 {
                n906 = while {
                  tunnel: [w2813] -> w2810
                  tunnel: w2809 -> [w2811]
                  i -> [w2819]
                  stop <- w2816 stop-if-true
                  w2814 = T61[] [enum."Testing"] items=["Online", "Pass", "Fail", "Testing", "Ready for Model", "Error Bit 1", "Error Bit 2", "Error Bit 3", "Failure Bit 1", "Failure Bit 2", "Failure Bit 3", "Failure Bit 4", "Echo Bit 1", "Echo Bit 2", "Echo Bit 3", "Echo Bit 4", "Serial Number Read Ok", "Ready for Serrial Number"] ("Digital Inputs Array")
                  # "Check if testing=1, look for this condition\nuntill it is true or 10 seconds expire."
                  n907 = Wait (ms)(milliseconds to wait=u32 100) -> ()  [unwired: 1 out]
                  n908 = Greater Or Equal?(x=w2819, y=100) -> (x >= y?=w2817:bool)
                  n909 = call "EOL NVH Inputs Controls Buffer 2.0.vi"("NVH Configuration"=w2811, "NVHK Inputs Control"=w2814, "Mode"=NVH_Mode_Control_2.0."Read") -> ("NVH Single Input"=w2813:bool)  [unwired: 4 in, 4 out]
                  n910 = Or(x=w2813, y=w2817) -> (x .or. y?=w2816:bool)
                }
              }
            }
            n911 = case shown="真" w2768 {
              tunnel: [w2778 w2783] -> w2773
              tunnel: w2772 -> [w2782 w2788]
              tunnel: w2771 -> [w2777 w2789]
              tunnel: [w2776 w2789] -> w2770
              tunnel: [w2781 w2788] -> w2769
              tunnel: w2767 -> [_ w2784]
              tunnel: w2766 -> [w2779 w2783]
              frame False {
                n912 = call "EOL Error Table.vi"("Error No."=u16 38, "Error Table In"=w2782) -> ("Error Table Out"=w2781:string[][])  [unwired: 8 in, 1 out]
                n913 = call "pass fail action decision.vi"("Pass?"=FALSE, "Sequence State in"=w2777, "event queue in"=w2779) -> ("Sequence State out"=w2776:T24, "Event queue out"=w2778:string[])  [unwired: 7 in]
              }
              frame True {
                w2786 = T69[] [enum."Start Test"] items=["Restart IRQ", "Abort Test IRQ", "Read Model", "Start Test", "Stop Test", "End of Test IRQ", "Test Bit 1", "Test Bit 2", "Test Bit 3", "Test Bit 4", "Model Bit 1", "Model Bit 2", "Model Bit 3", "Model Bit 4", "Manual Restart IRQ"] ("B&K Outputs Control")
                n914 = call "EOL NVH Outputs Controls Buffer 2.0.vi"("Mode"=NVH_Mode_Control_2.0."Write", "NVH Outputs Control"=w2786, "NVH Configuration"=w2784, "NVH Outputs"=bool[] [FALSE]) -> ()  [unwired: 6 in, 6 out]
              }
            }
          }
        }
        n915 = Bundle By Name(cluster=w2756, "Sequence State"=w2759, "Store Data.Error Table"=w2758) -> (w2757:T1)
      }
      frame "NVH Stop Test" {
        # "1) Send Stop Test bit only when the NVH system is running\n2) Send the stop test bit\n3) Wait for 300msecs\n4) Check whether the \"Testing\" bit is low.   Check untill it is false or timer expires.\n5) ResEt the stop test bit"
        n916 = Unbundle By Name(w2830) -> ("Sequence State"=w2835:T24, "Store Data.Error Table"=w2836:string[][], "Sequence State.NVH Status.NVH Test Running?"=w2832:bool, "NVH Configuration.NVH Station?"=w2828:bool, "NVH Configuration"=w2827:T6, "Store Data.Motion Data Array"=w2822:T11[])
        n917 = Array Size(array=w2822) -> (size(s)=w2824:i32)
        n918 = Decrement(x=w2824) -> (x-1=w2823:i32)
        n919 = Index Array(array=w2822, index=w2823) -> (element=w2821:T11)
        n920 = Unbundle By Name(w2821) -> ("Motion Data Limits.Check Sound Test"=w2820:bool)
        n921 = Compound Arithmetic op=AND(w2832, w2820, w2828) -> (w2831:bool)
        n922 = case shown="真" w2831 {
          tunnel: w2836 -> [w2838 w2847]
          tunnel: w2835 -> [w2839 w2846]
          tunnel: [w2839 w2845] -> w2834
          tunnel: [w2838 w2844] -> w2833
          tunnel: w2827 -> [_ w2843]
          tunnel: w2826 -> [w2837 w2842]
          tunnel: [w2837 w2841] -> w2825
          frame False {
          }
          frame True {
            n923 = stacked-sequence {
              tunnel: [_ _ w2869 _] -> w2848
              tunnel: w2843 -> [w2863 _ w2868 w2879]
              frame #0 {
                w2865 = T69[] [enum."Stop Test", enum."Start Test"] items=["Restart IRQ", "Abort Test IRQ", "Read Model", "Start Test", "Stop Test", "End of Test IRQ", "Test Bit 1", "Test Bit 2", "Test Bit 3", "Test Bit 4", "Model Bit 1", "Model Bit 2", "Model Bit 3", "Model Bit 4", "Manual Restart IRQ"] ("B&K Outputs Control")
                n924 = call "EOL NVH Outputs Controls Buffer 2.0.vi"("Mode"=NVH_Mode_Control_2.0."Write", "NVH Outputs Control"=w2865, "NVH Configuration"=w2863, "NVH Outputs"=bool[] [TRUE, FALSE]) -> ()  [unwired: 6 in, 6 out]
              }
              frame #1 {
                n925 = Wait (ms)(milliseconds to wait=u32 100 ("START TEST STEP B&K")) -> ()  [unwired: 1 out]
              }
              frame #2 {
                n926 = while {
                  tunnel: [w2872] -> w2869
                  tunnel: w2868 -> [w2870]
                  i -> [w2878]
                  stop <- w2875 stop-if-true
                  w2873 = T61[] [enum."Testing"] items=["Online", "Pass", "Fail", "Testing", "Ready for Model", "Error Bit 1", "Error Bit 2", "Error Bit 3", "Failure Bit 1", "Failure Bit 2", "Failure Bit 3", "Failure Bit 4", "Echo Bit 1", "Echo Bit 2", "Echo Bit 3", "Echo Bit 4", "Serial Number Read Ok", "Ready for Serrial Number"] ("Digital Inputs Array")
                  # "Check if testing=0, look for this condition\nuntill it is true or 15 seconds expire."
                  n927 = Greater Or Equal?(x=w2878, y=150) -> (x >= y?=w2876:bool)
                  n928 = call "EOL NVH Inputs Controls Buffer 2.0.vi"("NVH Configuration"=w2870, "NVHK Inputs Control"=w2873, "Mode"=NVH_Mode_Control_2.0."Read") -> ("NVH Single Input"=w2872:bool)  [unwired: 4 in, 4 out]
                  n929 = Compound Arithmetic op=OR(invert w2872, w2876) -> (w2875:bool)
                  n930 = Wait (ms)(milliseconds to wait=u32 100) -> ()  [unwired: 1 out]
                }
              }
              frame #3 {
                w2881 = T69[] [enum."Stop Test"] items=["Restart IRQ", "Abort Test IRQ", "Read Model", "Start Test", "Stop Test", "End of Test IRQ", "Test Bit 1", "Test Bit 2", "Test Bit 3", "Test Bit 4", "Model Bit 1", "Model Bit 2", "Model Bit 3", "Model Bit 4", "Manual Restart IRQ"] ("B&K Outputs Control")
                n931 = call "EOL NVH Outputs Controls Buffer 2.0.vi"("Mode"=NVH_Mode_Control_2.0."Write", "NVH Outputs Control"=w2881, "NVH Configuration"=w2879, "NVH Outputs"=bool[] [FALSE]) -> ()  [unwired: 6 in, 6 out]
              }
            }
            n932 = case shown="假" w2848 {
              tunnel: w2847 -> [w2852 w2862]
              tunnel: w2846 -> [w2853 w2856]
              tunnel: [w2853 w2855] -> w2845
              tunnel: [w2852 w2861] -> w2844
              tunnel: w2842 -> [w2851 w2858]
              tunnel: [w2850 w2857] -> w2841
              tunnel: failure_behaviors."stop at next 'check sequence' if not rabbit" ("fail behavior") -> [_ w2854]
              frame False {
                n933 = call "Insert Multiple Events.vi"("Events to Insert"=string[] ["NVH Check Error"] ("event queue out"), "Event queue in"=w2851) -> ("Event queue out"=w2850:string[])  [unwired: 2 in, 3 out]
              }
              frame True {
                n934 = call "EOL Error Table.vi"("Error No."=u16 39, "Error Table In"=w2862) -> ("Error Table Out"=w2861:string[][])  [unwired: 8 in, 1 out]
                n935 = call "pass fail action decision.vi"("fail behavior"=w2854, "Pass?"=FALSE, "Sequence State in"=w2856, "event queue in"=w2858) -> ("Sequence State out"=w2855:T24, "Event queue out"=w2857:string[])  [unwired: 6 in]
              }
            }
          }
        }
        n936 = Bundle By Name(cluster=w2830, "Sequence State"=w2834, "Store Data.Error Table"=w2833) -> (w2829:T1)
      }
      frame "NVH Test Needed?" {
        n937 = Unbundle By Name(w2899) -> ("Sequence State"=w2893:T24, "Store Data.Error Table"=w2894:string[][], "Sequence State.NVH Status.NVH Test Running?"=w2895:bool, "Store Data.Motion Data Array"=w2884:T11[], "NVH Configuration.NVH Station?"=w2889:bool, "NVH Configuration"=w2888:T6)
        n938 = Array Size(array=w2884) -> (size(s)=w2887:i32)
        n939 = Decrement(x=w2887) -> (x-1=w2886:i32)
        n940 = Index Array(array=w2884, index=w2886) -> (element=w2885:T11)
        n941 = Unbundle By Name(w2885) -> ("Motion Data Limits.Check Sound Test"=w2883:bool)
        n942 = Compound Arithmetic op=AND(w2895, w2883, w2889) -> (w2890:bool)
        n943 = case shown="真" w2890 {
          tunnel: w2894 -> [w2902 w2909]
          tunnel: [w2902 w2908] -> w2891
          tunnel: w2893 -> [w2901 w2906]
          tunnel: [w2901 w2907] -> w2892
          tunnel: w2888 -> [_ w2905]
          tunnel: w2897 -> [w2900 w2904]
          tunnel: [w2900 w2903] -> w2896
          frame False {
          }
          frame True {
            n944 = while {
              tunnel: [w2927] -> w2910
              tunnel: w2905 -> [w2925]
              i -> [w2936]
              stop <- w2933 stop-if-true
              w2931 = T61[] [enum."Online", enum."Testing"] items=["Online", "Pass", "Fail", "Testing", "Ready for Model", "Error Bit 1", "Error Bit 2", "Error Bit 3", "Failure Bit 1", "Failure Bit 2", "Failure Bit 3", "Failure Bit 4", "Echo Bit 1", "Echo Bit 2", "Echo Bit 3", "Echo Bit 4", "Serial Number Read Ok", "Ready for Serrial Number"] ("Digital Inputs Array")
              # "Check if online=1 & testing=0, look for this condition\nuntill it is true or 3 iterations."
              n945 = Greater Or Equal?(x=w2936, y=30) -> (x >= y?=w2934:bool)
              n946 = Wait (ms)(milliseconds to wait=u32 100) -> ()  [unwired: 1 out]
              n947 = call "EOL NVH Inputs Controls Buffer 2.0.vi"("NVH Configuration"=w2925, "NVHK Inputs Control"=w2931, "Mode"=NVH_Mode_Control_2.0."Read") -> ("NVH Inputs Out"=w2928:bool[])  [unwired: 4 in, 4 out]
              n948 = Index Array(array=w2928) -> (element #1=w2930:bool, element #2=w2929:bool)  [unwired: 2 in]
              n949 = Compound Arithmetic op=AND(w2930, invert w2929) -> (w2927:bool)
              n950 = Or(x=w2927, y=w2934) -> (x .or. y?=w2933:bool)
            }
            n951 = case shown="真" w2910 {
              tunnel: w2909 -> [w2918 w2923]
              tunnel: [w2917 w2923] -> w2908
              tunnel: [w2913 w2924] -> w2907
              tunnel: w2906 -> [w2914 w2924]
              tunnel: w2904 -> [w2912 w2922]
              tunnel: [w2911 w2919] -> w2903
              frame False {
                n952 = call "EOL Error Table.vi"("Error No."=u16 40, "Error Table In"=w2918) -> ("Error Table Out"=w2917:string[][])  [unwired: 8 in, 1 out]
                n953 = call "pass fail action decision.vi"("Pass?"=FALSE, "Sequence State in"=w2914, "event queue in"=w2912) -> ("Sequence State out"=w2913:T24, "Event queue out"=w2911:string[])  [unwired: 7 in]
              }
              frame True {
                n954 = call "Insert Multiple Events.vi"("Insert all? (T)"=TRUE, "Events to Insert"=string[] ["NVH Start Test"] ("event queue out"), "Event queue in"=w2922) -> ("Event queue out"=w2919:string[])  [unwired: 1 in, 3 out]
              }
            }
          }
        }
        n955 = Bundle By Name(cluster=w2899, "Sequence State"=w2892, "Store Data.Error Table"=w2891) -> (w2898:T1)
      }
      frame "check NVH Operator result" {
        n956 = Unbundle By Name(w2939) -> ("Config Info"=w2940:T34)
        n957 = Unbundle By Name(w2939) -> ("Second Check?"=w2938:bool)
        n958 = call "Config Info Get.vi"("Config Info"=w2940) -> ("PLC Comms"=w2937:T56)  [unwired: 7 in, 3 out]
        n959 = Unbundle By Name(w2937) -> ("PLC boolean read Tags"=w2955:T57, "PLC bool write Tags"=w2945:T58)
        n960 = Unbundle By Name(w2955) -> ("NVH Operator Pass"=w2954:T40, "NVH Operator Fail"=w2953:T40)
        n961 = Unbundle By Name(w2945) -> ("NVH Operator Pass"=w2944:T40, "NVH Operator Fail"=w2943:T40)
        n962 = Build Array(w2954, w2953) -> (w2952:T40[])
        n963 = Build Array(w2944, w2943) -> (w2942:T40[])
        n964 = for {
          tunnel: w2952 -> [w2971] mode=indexing
          tunnel: [w2970] -> w2951 mode=indexing
          n965 = call "plc read bool.vi"("addr,tag"=w2971) -> ("value"=w2970:bool)  [unwired: 9 in, 1 out]
        }
        n966 = Boolean Array To Number(Boolean array=w2951) -> (number=w2950:u32)
        n967 = case shown="0, 默认" w2950 {
          tunnel: [string[] ["check NVH Operator result"] ("Event queue out") string[] ["Sequence Complete"] ("Event queue out") w2967] -> w2948
          tunnel: [TRUE ("value") TRUE ("value") FALSE ("value")] -> w2947
          tunnel: [bool[] [FALSE, FALSE] bool[] [TRUE, FALSE] bool[] [FALSE, TRUE]] -> w2941
          tunnel: w2938 -> [_ _ w2964]
          frame 0, Default {
          }
          frame 1 {
          }
          frame 2 {
            n968 = case shown="真" w2964 {
              tunnel: [string[] ["Choose Noise Source"] ("Event queue out") string[] ["wait for operator action"] ("Event queue out")] -> w2967
              frame True {
              }
              frame False {
              }
            }
          }
        }
        n969 = for {
          tunnel: w2942 -> [w2957] mode=indexing
          tunnel: w2941 -> [w2956] mode=indexing
          n970 = call "plc write bool.vi"("value"=w2956, "addr,tag"=w2957) -> ()  [unwired: 9 in, 1 out]
        }
        n971 = Bundle By Name(cluster=w2939, "Operator Pass?"=w2947) -> (w2946:T1)
      }
      frame "write NVH result" {
        n972 = Unbundle By Name(w2975) -> ("Config Info"=w2976:T34)
        n973 = Unbundle By Name(w2975) -> ("NVH Pass?"=w2979:bool)
        n974 = call "Config Info Get.vi"("Config Info"=w2976) -> ("PLC Comms"=w2974:T56)  [unwired: 7 in, 3 out]
        n975 = Unbundle By Name(w2974) -> ("PLC bool write Tags"=w2973:T58)
        n976 = Unbundle By Name(w2973) -> ("NVH Pass"=w2978:T40, "NVH Fail"=w2983:T40)
        n977 = Not(x=w2979) -> (.not. x?=w2981:bool)
        n978 = Build Array(w2979, w2981) -> (w2980:bool[])
        n979 = Build Array(w2978, w2983) -> (w2982:T40[])
        n980 = for {
          tunnel: w2982 -> [w2986] mode=indexing
          tunnel: w2980 -> [w2985] mode=indexing
          tunnel: [w2984] -> w2972
          n981 = call "plc write bool.vi"("value"=w2985, "addr,tag"=w2986) -> ("error out"=w2984:errorcluster)  [unwired: 9 in]
        }
      }
      frame "--------Switch--------" {
      }
      frame "Set Digital Output" {
        n982 = Unbundle By Name(w3005) -> ("Sequence State"=w2992:T24, "Sequence State.Step Data String"=w3003:string, "Sequence State.Step Description"=w2999:string, "DO Task"=w2990:refnum<k21>, "Store Data.Error Table"=w3002:string[][])
        n983 = call "State Set Digital Output.vi"("Sys Error In"=w2997, "task/channels in"=w2990, "Step Description"=w2999, "Step Data String"=w3003) -> ("Sys Error Out"=w2996:errorcluster, "Error No."=w3001:u16, "Error String"=w2998:string, "Pass?"=w2994:bool)  [unwired: 4 in]
        n984 = case shown="假" w2994 {
          tunnel: w3002 -> [w3009 w3010]
          tunnel: [w3008 w3010] -> w3000
          tunnel: w2998 -> [w3007 _]
          tunnel: w3001 -> [w3006 _]
          frame False {
            n985 = call "EOL Error Table.vi"("Error Description"=w3007, "Error No."=w3006, "Error Table In"=w3009) -> ("Error Table Out"=w3008:string[][])  [unwired: 7 in, 1 out]
          }
          frame True {
          }
        }
        n986 = call "pass fail action decision.vi"("Pass?"=w2994, "Sequence State in"=w2992, "event queue in"=w2995) -> ("Sequence State out"=w2991:T24, "Event queue out"=w2993:string[])  [unwired: 7 in]
        n987 = Bundle By Name(cluster=w3005, "Sequence State"=w2991, "Store Data.Error Table"=w3000) -> (w3004:T1)
      }
      frame "Reset Switch Outputs" {
        n988 = Unbundle By Name(w3033) -> ("ctl refs.Waveform Graph"=w3040:refnum<vi>, "Store Data.Module Info.Serial Number"=w3047:string, "Motion Status.Analog Data"=w3044:sgl[][], "Motion Status.Motion"=w3036:T3, "misc status.Part Setup.Motor Type"=w3037:T30)  [unwired: 1 out]
        n989 = Unbundle By Name(w3033) -> ("DO Task"=w3032:refnum<k21>)
        n990 = Format Into String(w3036) -> (resulting string=w3042:string)  [unwired: 3 in, 1 out]
        n991 = Build Array(EOL_Global_Digital_Output_Control."Switch 1" ("Global DO Ch"), EOL_Global_Digital_Output_Control."Switch 2" ("Global DO Ch"), EOL_Global_Digital_Output_Control."Switch 3" ("Global DO Ch"), EOL_Global_Digital_Output_Control."Switch 4" ("Global DO Ch"), EOL_Global_Digital_Output_Control."Switch 5" ("Global DO Ch"), EOL_Global_Digital_Output_Control."Switch 6" ("Global DO Ch"), EOL_Global_Digital_Output_Control."Glass Analog Switch 1" ("Global DO Ch"), EOL_Global_Digital_Output_Control."Glass Analog Switch 2" ("Global DO Ch"), EOL_Global_Digital_Output_Control."Glass Analog Switch 3" ("Global DO Ch"), EOL_Global_Digital_Output_Control."Glass Analog Switch 4" ("Global DO Ch"), EOL_Global_Digital_Output_Control."Sunshade Analog Switch 1" ("Global DO Ch"), EOL_Global_Digital_Output_Control."Sunshade Analog Switch 2" ("Global DO Ch"), EOL_Global_Digital_Output_Control."Sunshade Analog Switch 3" ("Global DO Ch"), EOL_Global_Digital_Output_Control."Sunshade Analog Switch 4" ("Global DO Ch"), EOL_Global_Digital_Output_Control."Glass Motor Relay 1" ("Global DO Ch"), EOL_Global_Digital_Output_Control."Glass Motor Relay 2" ("Global DO Ch"), EOL_Global_Digital_Output_Control."Sunshade Motor Relay 1" ("Global DO Ch"), EOL_Global_Digital_Output_Control."Sunshade Motor Relay 2" ("Global DO Ch")) -> (w3013:T43[])
        n992 = call "select current channel.vi"("Current Motion"=w3036, "Motor Type"=w3037) -> ("Analog channel"=w3038:T37)  [unwired: 9 in]
        n993 = Concatenate Strings(w3047, "_" ("string"), w3042) -> (w3043:string)
        n994 = Index Array(array=w3044, index (col)=w3038) -> (element=w3039:sgl[])  [unwired: 1 in]
        n995 = for {
          tunnel: FALSE -> [w3051]
          tunnel: w3013 -> [w3052] mode=indexing
          tunnel: [w3050] -> w3011 mode=indexing
          n996 = Bundle By Name(cluster=T44 {"Status"=FALSE, "Global DO Ch"=enum."Battery"} ("Cluster"), "Global DO Ch"=w3052, "Status"=w3051) -> (w3050:T44)
        }
        n997 = property on="Property Node" class="WFGraph (严格)"(reference=w3040, "Legend Visible"=TRUE ("Legend:Visible"), "Plot.Plot Name"=w3043, "Value"=w3039) -> ()  [unwired: 1 in, 2 out]
        n998 = call "EOL Digital Outputs v3.vi"("task/channels in"=w3032, "Error In"=w3046, "DO Status"=w3011, "Mode"=T45."Write") -> ("Error Out"=w3045:errorcluster)  [unwired: 6 in, 1 out]
      }
      frame "Set RSLinx Tag Boolean" {
        n999 = Unbundle By Name(w3060) -> ("Sequence State"=w3054:T24, "Sequence State.Step Data String"=w3066:string, "Sequence State.Step Description"=w3062:string, "Store Data.Error Table"=w3065:string[][])
        n1000 = call "State Set RSLinx Tag Boolean.vi"("Sys Error In"=w3059, "Main State Cluster"=w3060, "Step Description"=w3062, "Step Data String"=w3066) -> ("Sys Error Out"=w3058:errorcluster, "Error No."=w3064:u8, "Error String"=w3061:string, "Pass?"=w3056:bool)  [unwired: 4 in]
        n1001 = case shown="假" w3056 {
          tunnel: w3065 -> [w3071 w3072]
          tunnel: [w3068 w3072] -> w3063
          tunnel: w3061 -> [w3069 _]
          tunnel: w3064 -> [w3070 _]
          frame False {
            n1002 = call "EOL Error Table.vi"("Error Description"=w3069, "Error No."=w3070, "Error Table In"=w3071) -> ("Error Table Out"=w3068:string[][])  [unwired: 7 in, 1 out]
          }
          frame True {
          }
        }
        n1003 = call "pass fail action decision.vi"("Pass?"=w3056, "Sequence State in"=w3054, "event queue in"=w3057) -> ("Sequence State out"=w3053:T24, "Event queue out"=w3055:string[])  [unwired: 7 in]
        n1004 = Bundle By Name(cluster=w3060, "Sequence State"=w3053, "Store Data.Error Table"=w3063) -> (w3067:T1)
      }
      frame "Set RSLinx Tag String" {
        n1005 = Unbundle By Name(w3080) -> ("Sequence State"=w3074:T24, "Sequence State.Step Data String"=w3086:string, "Sequence State.Step Description"=w3082:string, "Store Data.Error Table"=w3085:string[][])
        n1006 = call "State Set RSLinx Tag String.vi"("Sys Error In"=w3079, "Main State Cluster"=w3080, "Step Description"=w3082, "Step Data String"=w3086) -> ("Sys Error Out"=w3078:errorcluster, "Error No."=w3084:u8, "Error String"=w3081:string, "Pass?"=w3075:bool)  [unwired: 4 in]
        n1007 = case shown="假" w3075 {
          tunnel: w3085 -> [w3091 w3092]
          tunnel: [w3088 w3092] -> w3083
          tunnel: w3081 -> [w3090 _]
          tunnel: w3084 -> [w3089 _]
          frame False {
            n1008 = call "EOL Error Table.vi"("Error Description"=w3090, "Error No."=w3089, "Error Table In"=w3091) -> ("Error Table Out"=w3088:string[][])  [unwired: 7 in, 1 out]
          }
          frame True {
          }
        }
        n1009 = call "pass fail action decision.vi"("Pass?"=w3075, "Sequence State in"=w3074, "event queue in"=w3077) -> ("Sequence State out"=w3073:T24, "Event queue out"=w3076:string[])  [unwired: 7 in]
        n1010 = Bundle By Name(cluster=w3080, "Sequence State"=w3073, "Store Data.Error Table"=w3083) -> (w3087:T1)
      }
      frame "Set Switch Output" {
        n1011 = Unbundle By Name(w3094) -> ("Store Data.Motion Data Array"=w3106:T11[], "Switch Output Array"=w3108:T2[], "Motion Status.Motion"=w3101:T3, "DO Task"=w3093:refnum<k21>, "Station Index"=w3097:i32, "Motion Status.Analog Data"=w3100:sgl[][], "Motion Status.Current Data Index"=w3099:i32)
        n1012 = Array Size(array=w3106) -> (size(s)=w3105:i32)
        n1013 = Decrement(x=w3105) -> (x-1=w3104:i32)
        n1014 = Index Array(array=w3106, index=w3104) -> (element=w3103:T11)
        n1015 = Unbundle By Name(w3103) -> ("Motion Data Limits.Express Motion?"=w3102:bool)
        n1016 = call "EOL Audit Set Switch Output.vi"("Current Data Index In"=w3099, "Station Index"=w3097, "Current Data In"=w3100, "Express Motion?"=w3102, "Error In"=w3095, "task/channels in"=w3093, "Current Motion"=w3101, "Switch Output Array"=w3108) -> ("Error Out"=w3107:errorcluster, "Current Data Index Out"=w3098:i32, "Current Data Out"=w3096:sgl[][])  [unwired: 1 in]
        n1017 = Tick Count (ms)() -> (millisecond timer value=w3110:u32)
        n1018 = Bundle By Name(cluster=w3094, "Motion Status.Motion Stop Timer"=w3110, "Motion Status.Analog Data"=w3096, "Motion Status.Current Data Index"=w3098) -> (w3109:T1)
      }
      frame "Turn Power Off" {
        n1019 = Unbundle By Name(w3116) -> ("DO Task"=w3115:refnum<k21>, "misc status.Part Setup.RAP Signal"=w3114:T29)
        n1020 = case shown="\"Low\"" w3114 {
          tunnel: w3115 -> [w3120 w3131 _]
          tunnel: [w3119 w3130 w3140] -> w3113
          tunnel: w3112 -> [w3118 w3129 w3140]
          frame "High", Default {
            n1021 = Bundle By Name(cluster=T44 {"Status"=FALSE, "Global DO Ch"=enum."Battery"} ("Cluster"), "Status"=FALSE, "Global DO Ch"=EOL_Global_Digital_Output_Control."Battery") -> (w3124:T44)
            n1022 = Bundle By Name(cluster=w3124, "Global DO Ch"=EOL_Global_Digital_Output_Control."IGN High") -> (w3122:T44)
            n1023 = Build Array(w3124, w3122) -> (w3121:T44[])
            n1024 = call "EOL Digital Outputs v3.vi"("task/channels in"=w3120, "Error In"=w3118, "DO Status"=w3121, "Mode"=T45."Write") -> ("Error Out"=w3119:errorcluster)  [unwired: 6 in, 1 out]
          }
          frame "Low" {
            n1025 = Bundle By Name(cluster=T44 {"Status"=FALSE, "Global DO Ch"=enum."Battery"} ("Cluster"), "Status"=FALSE, "Global DO Ch"=EOL_Global_Digital_Output_Control."Battery") -> (w3135:T44)
            n1026 = Bundle By Name(cluster=w3135, "Global DO Ch"=EOL_Global_Digital_Output_Control."IGN Low") -> (w3133:T44)
            n1027 = Build Array(w3135, w3133) -> (w3132:T44[])
            n1028 = call "EOL Digital Outputs v3.vi"("task/channels in"=w3131, "Error In"=w3129, "DO Status"=w3132, "Mode"=T45."Write") -> ("Error Out"=w3130:errorcluster)  [unwired: 6 in, 1 out]
          }
          frame "None" {
          }
        }
      }
      frame "Turn Power On" {
        # "50ms delay for enabling sense relay"
        n1029 = Unbundle By Name(w3145) -> ("DO Task"=w3144:refnum<k21>, "misc status.Part Setup.RAP Signal"=w3143:T29)
        n1030 = case shown="\"High\", 默认" w3143 {
          tunnel: w3144 -> [w3150 w3167 _]
          tunnel: w3142 -> [w3148 w3165 w3181]
          tunnel: [w3147 w3164 w3181] -> w3141
          frame "High", Default {
            n1031 = Bundle By Name(cluster=T44 {"Status"=FALSE, "Global DO Ch"=enum."Battery"} ("Cluster"), "Status"=TRUE, "Global DO Ch"=EOL_Global_Digital_Output_Control."Battery") -> (w3152:T44)
            n1032 = Bundle By Name(cluster=w3152, "Global DO Ch"=EOL_Global_Digital_Output_Control."IGN High") -> (w3151:T44)
            n1033 = Build Array(w3152, w3151) -> (w3155:T44[])
            n1034 = flat-sequence {
              tunnel: w3155 -> [w3161]
              tunnel: w3150 -> [w3160]
              tunnel: w3148 -> [w3159]
              tunnel: [w3158] -> w3147
              frame #0 {
                n1035 = Wait (ms)(milliseconds to wait=u32 50 ("等待时间（毫秒）")) -> ()  [unwired: 1 out]
              }
              frame #1 {
                n1036 = call "EOL Digital Outputs v3.vi"("task/channels in"=w3160, "Error In"=w3159, "DO Status"=w3161, "Mode"=T45."Write") -> ("Error Out"=w3158:errorcluster)  [unwired: 6 in, 1 out]
              }
              frame #2 {
                n1037 = Wait (ms)(milliseconds to wait=u32 50 ("等待时间（毫秒）")) -> ()  [unwired: 1 out]
              }
            }
          }
          frame "Low" {
            n1038 = Bundle By Name(cluster=T44 {"Status"=FALSE, "Global DO Ch"=enum."Battery"} ("Cluster"), "Status"=TRUE, "Global DO Ch"=EOL_Global_Digital_Output_Control."Battery") -> (w3169:T44)
            n1039 = Bundle By Name(cluster=w3169, "Global DO Ch"=EOL_Global_Digital_Output_Control."IGN Low") -> (w3168:T44)
            n1040 = Build Array(w3169, w3168) -> (w3172:T44[])
            n1041 = flat-sequence {
              tunnel: w3172 -> [w3178]
              tunnel: w3167 -> [w3177]
              tunnel: w3165 -> [w3176]
              tunnel: [w3175] -> w3164
              frame #0 {
                n1042 = Wait (ms)(milliseconds to wait=u32 50 ("等待时间（毫秒）")) -> ()  [unwired: 1 out]
              }
              frame #1 {
                n1043 = call "EOL Digital Outputs v3.vi"("task/channels in"=w3177, "Error In"=w3176, "DO Status"=w3178, "Mode"=T45."Write") -> ("Error Out"=w3175:errorcluster)  [unwired: 6 in, 1 out]
              }
              frame #2 {
                n1044 = Wait (ms)(milliseconds to wait=u32 50 ("等待时间（毫秒）")) -> ()  [unwired: 1 out]
              }
            }
          }
          frame "None" {
          }
        }
      }
      frame "Turn RAP Off", "Turn RAP On" {
        n1045 = Unbundle By Name(w3186) -> ("DO Task"=w3185:refnum<k21>, "misc status.Part Setup.RAP Signal"=w3184:T29)
        n1046 = case shown="\"High\", 默认" w3184 {
          tunnel: w3187 -> [w3195 w3206 _]
          tunnel: w3185 -> [w3192 w3203 _]
          tunnel: w3183 -> [w3190 w3201 w3211]
          tunnel: [w3189 w3200 w3211] -> w3182
          frame "High", Default {
            n1047 = Equal?(x="Turn RAP On", y=w3195) -> (x = y?=w3193:bool)
            n1048 = Bundle By Name(cluster=T44 {"Status"=FALSE, "Global DO Ch"=enum."Battery"} ("Cluster"), "Status"=w3193, "Global DO Ch"=EOL_Global_Digital_Output_Control."IGN High") -> (w3197:T44)
            n1049 = Build Array(w3197) -> (w3196:T44[])
            n1050 = call "EOL Digital Outputs v3.vi"("task/channels in"=w3192, "Error In"=w3190, "DO Status"=w3196, "Mode"=T45."Write") -> ("Error Out"=w3189:errorcluster)  [unwired: 6 in, 1 out]
          }
          frame "Low" {
            n1051 = Equal?(x="Turn RAP On", y=w3206) -> (x = y?=w3204:bool)
            n1052 = Bundle By Name(cluster=T44 {"Status"=FALSE, "Global DO Ch"=enum."Battery"} ("Cluster"), "Status"=w3204, "Global DO Ch"=EOL_Global_Digital_Output_Control."IGN Low") -> (w3208:T44)
            n1053 = Build Array(w3208) -> (w3207:T44[])
            n1054 = call "EOL Digital Outputs v3.vi"("task/channels in"=w3203, "Error In"=w3201, "DO Status"=w3207, "Mode"=T45."Write") -> ("Error Out"=w3200:errorcluster)  [unwired: 6 in, 1 out]
          }
          frame "None" {
          }
        }
      }
      frame "--------Others--------" {
      }
      frame "Sunshade Servo Close", "Sunshade Servo Open" {
        n1055 = Unbundle By Name(w3231) -> ("Sequence State"=w3217:T24, "ctl refs.Sunshade Servo Data Close"=w3229:refnum<vi>, "ctl refs.Sunshade Servo Data Open"=w3228:refnum<vi>)
        n1056 = case shown="\"Sunshade Servo Open\", 默认" w3224 {
          tunnel: [w3244 w3246] -> w3230
          tunnel: w3229 -> [_ w3246]
          tunnel: w3228 -> [w3244 _]
          tunnel: [w3243 w3245] -> w3227
          frame "Sunshade Servo Open", Default {
            w3243 = FALSE  # Sunshade Close Test?
          }
          frame "Sunshade Servo Close" {
            w3245 = TRUE  # Sunshade Close Test?
          }
        }
        n1057 = call "EOL Sunshade Servo Test.vi"("scaling factor"=20.0, "input cluster"=w3231, "Sunshade Close Test?"=w3227) -> ("Error Table Out"=w3232:string[][], "Sunshade Raw Data"=w3221:dbl[], "Sunshade Calculated Data"=w3223:dbl[], "Pass? Out"=w3220:bool, "ss servo limits"=w3222:T14)  [unwired: 4 in]
        n1058 = property class="WFGraph (严格)"(reference=w3230, "Value"=w3221) -> ()  [unwired: 1 in, 2 out]
        n1059 = call "pass fail action decision.vi"("Pass?"=w3220, "Sequence State in"=w3217, "event queue in"=w3219) -> ("Sequence State out"=w3216:T24, "Event queue out"=w3218:string[])  [unwired: 7 in]
        n1060 = Bundle By Name(cluster=w3231, "Sequence State"=w3216, "Store Data.Error Table"=w3232) -> (w3226:T1)
        n1061 = case shown="\"Sunshade Servo Open\", 默认" w3224 {
          tunnel: w3226 -> [w3237 w3242]
          tunnel: [w3236 w3241] -> w3225
          tunnel: w3223 -> [w3235 w3240]
          tunnel: w3222 -> [w3234 w3239]
          tunnel: w3221 -> [w3233 w3238]
          frame "Sunshade Servo Close" {
            n1062 = Bundle By Name(cluster=w3237, "Store Data.Sunshade Close Data"=w3235, "Store Data.Sun Shade Close Force Limits"=w3234, "Store Data.Sunsahde Close Raw Data"=w3233) -> (w3236:T1)
          }
          frame "Sunshade Servo Open", Default {
            n1063 = Bundle By Name(cluster=w3242, "Store Data.Sunshade Open Data"=w3240, "Store Data.Sun Shade Open Force Limits"=w3239, "Store Data.Sunshade Open Raw Data"=w3238) -> (w3241:T1)
          }
        }
      }
      frame "Turn LIN Power Restart" {
        w3248 = EOL_Global_Digital_Output_Control."Battery" ("Global DO Ch")
        # "50ms delay for enabling sense relay"
        n1064 = Unbundle By Name(w3249) -> ("DO Task"=w3247:refnum<k21>)
        n1065 = Bundle By Name(cluster=T44 {"Status"=FALSE, "Global DO Ch"=enum."Battery"} ("Cluster"), "Status"=TRUE, "Global DO Ch"=w3248) -> (w3254:T44)
        n1066 = Bundle By Name(cluster=T44 {"Status"=FALSE, "Global DO Ch"=enum."Battery"} ("Cluster"), "Status"=FALSE, "Global DO Ch"=w3248) -> (w3257:T44)
        n1067 = Build Array(w3254) -> (w3250:T44[])
        n1068 = Build Array(w3257) -> (w3251:T44[])
        n1069 = stacked-sequence {
          tunnel: w3251 -> [_ w3261 _ _ _]
          tunnel: w3250 -> [_ _ _ w3265 _]
          tunnel: w3247 -> [_ w3260 _ w3264 _]
          frame #0 {
            n1070 = Wait (ms)(milliseconds to wait=u32 700) -> ()  [unwired: 1 out]
          }
          frame #1 {
            n1071 = call "EOL Digital Outputs v3.vi"("task/channels in"=w3260, "DO Status"=w3261, "Mode"=T45."Write") -> ()  [unwired: 7 in, 2 out]
          }
          frame #2 {
            n1072 = Wait (ms)(milliseconds to wait=u32 1500) -> ()  [unwired: 1 out]
          }
          frame #3 {
            n1073 = call "EOL Digital Outputs v3.vi"("task/channels in"=w3264, "DO Status"=w3265, "Mode"=T45."Write") -> ()  [unwired: 7 in, 2 out]
          }
          frame #4 {
            n1074 = Wait (ms)(milliseconds to wait=u32 700) -> ()  [unwired: 1 out]
          }
        }
      }
      frame "Update Error Table" {
        n1075 = Unbundle By Name(w3280) -> ("Sequence State.Pass?"=w3286:bool, "Store Data.Error Table"=w3273:string[][], "Sequence State.Cycle Start Time"=w3285:u32, "ctl refs.all station status"=w3274:refnum<vi>)
        n1076 = Tick Count (ms)() -> (millisecond timer value=w3284:u32)
        n1077 = Subtract(x=w3284, y=w3285) -> (x-y=w3283:u32)
        n1078 = Divide(x=w3283, y=u32 1000) -> (x/y=w3271:dbl)
        n1079 = Format Into String(format string="%0.2f", error in=w3269, w3271) -> (resulting string=w3270:string, error out=w3268:errorcluster)  [unwired: 1 in]
        n1080 = property class="Clust (严格)"(reference=w3274) -> (reference out=w3278:refnum<vi>, error out=w3275:errorcluster, "Value"=w3276:T52)  [unwired: 1 in]
        n1081 = Select(t=u32 6618880 ("Pass/Fail AU"), s=w3286, f=u32 16711680 ("Pass/Fail AU")) -> (s? t:f=w3272:u32)
        n1082 = Bundle By Name(cluster=w3276, "Error Table Br"=w3273, "Pass / Fail"=w3272, "Cycle Time Br"=w3271) -> (w3277:T52)
        n1083 = Bundle By Name(cluster=w3280, "Store Data.Cycle Time"=w3270) -> (w3279:T1)
        n1084 = property class="Clust (严格)"(reference=w3278, error in=w3275, "Value"=w3277) -> ()  [unwired: 2 out]
      }
      frame "Write Errors to File" {
        n1085 = Unbundle By Name(w3294) -> ("paths.Store errors log path"=w3292:path, "Store Data.Module Info.Serial Number"=w3295:string, "Store Data.Error Table"=w3296:string[][], "misc station config.Station Name"=w3293:string)
        n1086 = call "Upload Errors To File.vi"("Station"=w3293, "error in"=w3291, "Error Table"=w3296, "Serial Number"=w3295, "Path"=w3292) -> ("error out"=w3290:errorcluster)  [unwired: 6 in]
      }
      frame "Write Test Complete to PLC" {
        n1087 = Unbundle By Name(w3302) -> ("ctl refs.all station status"=w3317:refnum<vi>, "Sequence State.Red-Rabbit Mode"=w3305:bool, "misc station config.is audit station?"=w3306:bool, "Sequence State.route-to-repair mode"=w3310:bool, "Sequence State.Pass?"=w3326:bool, "D in map.Abort Test"=w3328:T17, "ctl refs.Abort Test"=w3313:refnum<vi>)  [unwired: 1 out]
        n1088 = Unbundle By Name(w3302) -> ("Config Info"=w3303:T34)
        n1089 = call "Config Info Get.vi"("Config Info"=w3303) -> ("PLC Comms"=w3301:T56)  [unwired: 7 in, 3 out]
        n1090 = Unbundle By Name(w3301) -> ("PLC bool write Tags.Test Started"=w3300:T40, "PLC bool write Tags.Test Complete Pass"=w3299:T40, "PLC bool write Tags.Test Complete Fail"=w3298:T40)
        n1091 = Compound Arithmetic op=AND(invert w3310, w3326) -> (w3308:bool)
        n1092 = Compound Arithmetic op=AND(invert w3306, w3305) -> (w3307:bool)
        n1093 = Or(x=w3307, y=w3308) -> (x .or. y?=w3309:bool)
        n1094 = Not(x=w3309) -> (.not. x?=w3324:bool)
        n1095 = Build Array(w3300, w3299, w3298) -> (w3321:T40[])
        n1096 = Build Array(w3328) -> (w3327:T17[])
        n1097 = Build Array(w3299, w3298) -> (w3325:T40[])
        n1098 = Build Array(w3309, w3324) -> (w3323:bool[])
        n1099 = property class="Clust (严格)"(reference=w3317, error in=w3311) -> (reference out=w3316:refnum<vi>, error out=w3314:errorcluster, "Value"=w3315:T52)
        n1100 = Bundle By Name(cluster=w3315, "Application Status"="Wait For PLC Abort Signal" ("t")) -> (w3312:T52)
        n1101 = property class="Clust (严格)"(reference=w3316, error in=w3314, "Value"=w3312) -> (error out=w3304:errorcluster)  [unwired: 1 out]
        n1102 = for {
          shift-right: [w3339] -> w3322
          shift-left: w3304 -> [w3338]
          tunnel: w3325 -> [w3337] mode=indexing
          tunnel: w3323 -> [w3336] mode=indexing
          n1103 = call "plc write bool.vi"("error in"=w3338, "value"=w3336, "addr,tag"=w3337) -> ("error out"=w3339:errorcluster)  [unwired: 8 in]
          n1104 = Wait Until Next ms Multiple(millisecond multiple=u32 300 ("milliseconds to wait")) -> ()  [unwired: 1 out]
        }
        n1105 = while {
          tunnel: w3327 -> [w3346]
          shift-right: [w3342] -> w3320
          shift-left: w3322 -> [w3345]
          tunnel: w3313 -> [w3343]
          stop <- w3348 stop-if-true
          n1106 = property on="Property Node" class="Bool (严格)"(reference=w3343, error in=w3345) -> (error out=w3344:errorcluster, "Value"=w3341:bool)  [unwired: 1 out]
          n1107 = call "EOL Digital Inputs v2.vi"("Sys Error In"=w3344, "Digital Inputs Array"=w3346, "Mode"=enum16{"Init", "Read", "Read All", "Close"}."Read") -> ("Sys Error Out"=w3342:errorcluster, "Single Input"=w3340:bool)  [unwired: 6 in, 1 out]
          n1108 = Compound Arithmetic op=OR(w3341, w3340, w3342) -> (w3348:bool)
          n1109 = Wait (ms)(milliseconds to wait=u32 150) -> ()  [unwired: 1 out]
        }
        n1110 = for {
          shift-right: [w3334] -> w3319
          shift-left: w3320 -> [w3333]
          tunnel: w3321 -> [w3332] mode=indexing
          n1111 = call "plc write bool.vi"("error in"=w3333, "value"=FALSE, "addr,tag"=w3332) -> ("error out"=w3334:errorcluster)  [unwired: 8 in]
          n1112 = Wait Until Next ms Multiple(millisecond multiple=u32 5 ("milliseconds to wait")) -> ()  [unwired: 1 out]
        }
      }
      frame "error" {
        n1113 = Unbundle By Name(w3366) -> ("Sequence State"=w3360:T24, "Store Data.Error Table"=w3358:string[][], "paths.system error log path"=w3363:path, "misc station config.Station Name"=w3370:string)
        n1114 = Wait Until Next ms Multiple(millisecond multiple=u32 250) -> ()  [unwired: 1 out]
        n1115 = Concatenate Strings("Error in " ("string"), w3370, ", " ("string"), w3369) -> (w3364:string)
        n1116 = Unbundle By Name(w3354) -> ("source"=w3352:string)
        n1117 = Concatenate Strings(w3364, ", " ("string"), w3352) -> (w3355:string)
        n1118 = call "Log System Errors to File.vi"("error out"=w3354, "Comments"=w3355, "Path"=w3363) -> ("error out"=w3371:errorcluster)  [unwired: 8 out]
        n1119 = call "EOL Error Table.vi"("Error Description"=w3355, "Error No."=u16 174, "Error Table In"=w3358) -> ("Error Table Out"=w3359:string[][])  [unwired: 7 in, 1 out]
        n1120 = call "pass fail action decision.vi"("Pass?"=FALSE, "Sequence State in"=w3360, "event queue in"=w3356) -> ("Sequence State out"=w3361:T24, "Event queue out"=w3357:string[])  [unwired: 7 in]
        n1121 = Bundle By Name(cluster=w3366, "Sequence State"=w3361, "Store Data.Error Table"=w3359) -> (w3365:T1)
        n1122 = call <vilib>:"Clear Errors.vi"("error in (no error)"=w3371) -> ("error out"=w3362:errorcluster)  [unwired: 5 in, 1 out]
      }
      frame "toggle comms power" {
        w3374 = EOL_Global_Digital_Output_Control."Battery" ("Global DO Ch")
        w3383 = T44 {"Status"=FALSE, "Global DO Ch"=enum."Battery"} ("Cluster")
        n1123 = Unbundle By Name(w3377) -> ("DO Task"=w3373:refnum<k21>)
        n1124 = Bundle By Name(cluster=w3383, "Status"=TRUE, "Global DO Ch"=w3374) -> (w3380:T44)
        n1125 = Bundle By Name(cluster=w3383, "Status"=FALSE, "Global DO Ch"=w3374) -> (w3381:T44)
        n1126 = Build Array(w3380) -> (w3379:T44[])
        n1127 = Build Array(w3381) -> (w3378:T44[])
        n1128 = flat-sequence {
          tunnel: w3378 -> [w3388]
          tunnel: w3373 -> [w3387]
          tunnel: [w3387] -> w3375
          tunnel: [w3390] -> w3376
          tunnel: w3375 -> [w3390]
          tunnel: w3379 -> [w3393]
          tunnel: w3376 -> [w3392]
          frame #0 {
            n1129 = call "EOL Digital Outputs v3.vi"("task/channels in"=w3387, "DO Status"=w3388, "Mode"=T45."Write") -> ()  [unwired: 7 in, 2 out]
          }
          frame #1 {
            n1130 = Wait (ms)(milliseconds to wait=u32 2000) -> ()  [unwired: 1 out]
          }
          frame #2 {
            n1131 = call "EOL Digital Outputs v3.vi"("task/channels in"=w3392, "DO Status"=w3393, "Mode"=T45."Write") -> ()  [unwired: 7 in, 2 out]
          }
        }
      }
      frame "wait for operator action" {
        (unwired) FALSE ("goto motion?")
        n1132 = Unbundle By Name(w3398) -> ("Config Info"=w3399:T34)
        n1133 = Unbundle By Name(w3398) -> ("NVH Motion Steps"=w3401:string[], "misc status.Part Setup.Part Type"=w3403:string, "ctl refs.all station status"=w3414:refnum<vi>, "Station Index"=w3412:i32, "misc status.PS Voltage"=w3408:dbl, "misc status.Part Setup.Motor Type"=w3407:T30)
        n1134 = call "Config Info Get.vi"("Config Info"=w3399) -> ("PLC Comms"=w3397:T56)  [unwired: 7 in, 3 out]
        n1135 = Unbundle By Name(w3397) -> ("PLC boolean read Tags"=w3395:T57, "PLC bool write Tags"=w3396:T58)
        n1136 = case shown="\"Smart Motor\", 默认" w3407 {
          tunnel: [string[] ["Init Motion", "Set Power Supply", "Set Switch Output", "Check Switch Signals", "Get Data"] ("event queue out") string[] ["Init Motion", "BMW Init Motion", "Set Power Supply", "NVH Test Needed?", "Set Switch Output", "Check Initial Motion", "BMW Check Hall Movement", "BMW Get Data", "BMW Check Motion Stop"] ("event queue out")] -> w3419
          frame "Smart Motor", Default {
          }
          frame "Sensor Motor" {
          }
        }
        n1137 = call "check operator action.vi"("Motion Steps in"=w3401, "Part Type"=w3403, "input cluster"=w3395) -> ("Step"=w3402:string, "data string"=w3404:string, "Motion Steps out"=w3400:string[])  [unwired: 6 in]
        n1138 = property class="Clust (严格)"(reference=w3414) -> (reference out=w3418:refnum<vi>, error out=w3415:errorcluster, "Value"=w3416:T52)  [unwired: 1 in]
        n1139 = Bundle By Name(cluster=w3416, "Current Step Br"=w3402) -> (w3417:T52)
        n1140 = property class="Clust (严格)"(reference=w3418, error in=w3415, "Value"=w3417) -> ()  [unwired: 2 out]
        n1141 = Bundle By Name(cluster=w3398, "Motion Status.Motion"=All_Motions."Idle" ("Motion Data.Current Motion"), "Operator Action?"=TRUE, "NVH Motion Steps"=w3400) -> (w3413:T1)
        n1142 = case shown="\"Sunshade Open 2\"" w3402 {
          selector: w3402 -> [w3425 _ w3444 _ _ _ _ _ _ _ _ _ _ _ _ _ _ _ _ w3569 _ _ _ _ _ _ w3624 _ _ _ _ _ _ _ _ _ _ _ _ _ _]
          tunnel: w3404 -> [w3428 w3438 w3449 w3458 w3462 w3469 w3479 w3483 w3490 w3500 w3504 w3511 w3521 w3528 w3535 w3542 w3549 w3553 w3560 w3568 w3582 w3586 w3593 w3603 w3607 w3614 w3629 w3645 w3649 w3656 w3666 w3670 w3677 w3696 w3705 w3715 w3722 w3729 w3736 w3744 w3752]
          tunnel: w3413 -> [w3433 w3440 w3452 w3457 w3465 w3472 w3478 w3486 w3493 w3499 w3507 w3514 w3520 w3527 w3534 w3541 w3548 w3556 w3563 w3571 w3581 w3589 w3596 w3602 w3610 w3617 w3625 w3644 w3652 w3659 w3665 w3673 w3680 w3701 w3708 w3714 w3721 w3728 w3735 w3742 w3753]
          tunnel: [w3434 w3441 w3451 w3456 w3464 w3471 w3477 w3485 w3492 w3498 w3506 w3513 w3519 w3526 w3533 w3540 w3547 w3555 w3562 w3570 w3580 w3588 w3595 w3601 w3609 w3616 w3632 w3643 w3651 w3658 w3664 w3672 w3679 w3700 w3709 w3713 w3720 w3727 w3734 w3745 w3754] -> w3421
          tunnel: [string[] ["Check Position Software", "Check Sequence"] string[] ["Delay", "Check Sequence"] w3445 w3454 w3460 w3467 w3475 w3481 w3488 w3496 w3502 w3509 w3517 w3524 w3531 w3538 w3545 w3551 w3558 w3566 w3578 w3584 w3591 w3599 w3605 w3612 w3619 w3641 w3647 w3654 w3662 w3668 w3675 w3682 string[] ["Set Power Supply", "Check Sequence"] w3711 w3718 w3725 w3732 string[] ["check NVH Operator result"] ("event queue out") w3751] -> w3420
          tunnel: "" ("Description") -> [_ w3437 _ _ _ _ _ _ _ _ _ _ _ _ _ _ _ _ _ _ _ _ _ _ _ _ _ _ _ _ _ _ _ _ _ _ _ _ _ w3743 w3749]
          tunnel: w3419 -> [_ _ _ w3454 w3460 w3467 w3475 w3481 w3488 w3496 w3502 w3509 w3517 w3524 w3531 w3538 w3545 w3551 w3558 w3566 w3578 w3584 w3591 w3599 w3605 w3612 w3619 w3641 w3647 w3654 w3662 w3668 w3675 w3682 _ w3711 w3718 w3725 w3732 _ _]
          tunnel: w3412 -> [_ _ _ _ _ _ _ _ _ _ _ _ _ _ _ _ _ _ _ _ _ _ _ _ _ _ w3626 _ _ _ _ _ _ _ _ _ _ _ _ _ _]
          tunnel: w3411 -> [w3427 w3435 w3450 w3453 w3461 w3468 w3474 w3482 w3489 w3495 w3503 w3510 w3516 w3523 w3530 w3537 w3544 w3552 w3559 w3567 w3577 w3585 w3592 w3598 w3606 w3613 w3620 w3640 w3648 w3655 w3661 w3669 w3676 w3695 w3703 w3710 w3717 w3724 w3731 w3747 w3748]
          tunnel: [w3427 w3435 w3450 w3453 w3461 w3468 w3474 w3482 w3489 w3495 w3503 w3510 w3516 w3523 w3530 w3537 w3544 w3552 w3559 w3567 w3577 w3585 w3592 w3598 w3606 w3613 w3620 w3640 w3648 w3655 w3661 w3669 w3676 w3689 w3702 w3710 w3717 w3724 w3731 w3747 w3748] -> w3410
          tunnel: w3408 -> [_ _ _ _ _ _ _ _ _ _ _ _ _ _ _ _ _ _ _ _ _ _ _ _ _ _ _ _ _ _ _ _ _ w3683 _ _ _ _ _ _ _]
          tunnel: w3407 -> [_ _ _ _ _ _ _ _ _ _ _ _ _ _ _ _ _ _ _ _ _ _ _ _ _ _ _ _ _ _ _ _ _ _ _ _ _ _ _ _ _]
          tunnel: w3396 -> [_ _ _ _ _ _ _ _ _ _ _ _ _ _ _ _ _ _ _ _ _ _ _ _ _ _ _ _ _ _ _ _ _ _ _ _ _ _ _ w3741 _]
          frame "Check Position Software Glass", "Check Position Software Sunshade" {
            n1143 = Scan From String(format string="%x", input string=w3428, default 1=u8 0 ("Hex Number")) -> (output 1=w3429:u8)  [unwired: 2 in, 3 out]
            n1144 = Equal?(x=w3425, y="Check Position Software Glass") -> (x = y?=w3424:bool)
            n1145 = Bundle By Name(cluster=w3433, "Motion Status.Motor Position Hex"=w3429, "misc status.Serial Port Configured?"=w3424) -> (w3434:T1)
          }
          frame "Delay In Seconds" {
            n1146 = Tick Count (ms)() -> (millisecond timer value=w3436:u32)
            n1147 = Bundle By Name(cluster=w3440, "Sequence State.Step Data String"=w3438, "Sequence State.Step Description"=w3437, "misc status.delay start time (ticks)"=w3436) -> (w3441:T1)
          }
          frame "Enter AP Message Mode Glass", "Enter AP Message Mode Sunshade" {
            n1148 = Scan From String(input string=w3449, default 1=17x_AP_Data_Type."91/61" ("AP Data Type")) -> (output 1=w3447:T13)  [unwired: 3 in, 3 out]
            n1149 = Equal?(x=w3444, y="Enter AP Message Mode Glass") -> (x = y?=w3443:bool)
            n1150 = Bundle By Name(cluster=w3452, "misc status.AP Data Type"=w3447, "misc status.Serial Port Configured?"=w3443) -> (w3451:T1)
            n1151 = Build Array (concatenate)(w3444, string[] ["Check Sequence"]) -> (w3445:string[])
          }
          frame "Express Glass Slide Close" {
            n1152 = Bundle By Name(cluster=w3457, "Motion Status.Motion"=All_Motions."Express Glass Slide Close" ("Current Motion"), "Sequence State.Step Data String"=w3458, "misc status.Serial Port Configured?"=TRUE ("Glass Motor?")) -> (w3456:T1)
          }
          frame "Express Glass Slide Close Sunshade Close" {
            n1153 = Bundle By Name(cluster=w3465, "Motion Status.Motion"=All_Motions."Express Glass Slide Close Sunshade Close" ("Current Motion"), "Sequence State.Step Data String"=w3462, "misc status.Serial Port Configured?"=TRUE ("Glass Motor?")) -> (w3464:T1)
          }
          frame "Express Glass Slide Close Sunshade Open" {
            n1154 = Bundle By Name(cluster=w3472, "Motion Status.Motion"=All_Motions."Express Glass Slide Close Sunshade Open" ("Current Motion"), "Sequence State.Step Data String"=w3469, "misc status.Serial Port Configured?"=TRUE ("Glass Motor?")) -> (w3471:T1)
          }
          frame "Express Glass Slide Open" {
            n1155 = Bundle By Name(cluster=w3478, "Motion Status.Motion"=All_Motions."Express Glass Slide Open" ("Current Motion"), "Sequence State.Step Data String"=w3479, "misc status.Serial Port Configured?"=TRUE ("Glass Motor?")) -> (w3477:T1)
          }
          frame "Express Glass Slide Open Sunshade Close" {
            n1156 = Bundle By Name(cluster=w3486, "Motion Status.Motion"=All_Motions."Express Glass Slide Open Sunshade Close" ("Current Motion"), "Sequence State.Step Data String"=w3483, "misc status.Serial Port Configured?"=TRUE ("Glass Motor?")) -> (w3485:T1)
          }
          frame "Express Glass Slide Open Sunshade Open" {
            n1157 = Bundle By Name(cluster=w3493, "Motion Status.Motion"=All_Motions."Express Glass Slide Open Sunshade Open" ("Current Motion"), "Sequence State.Step Data String"=w3490, "misc status.Serial Port Configured?"=TRUE ("Glass Motor?")) -> (w3492:T1)
          }
          frame "Express Glass Vent Close" {
            n1158 = Bundle By Name(cluster=w3499, "Motion Status.Motion"=All_Motions."Express Glass Vent Close" ("Current Motion"), "Sequence State.Step Data String"=w3500, "misc status.Serial Port Configured?"=TRUE ("Glass Motor?")) -> (w3498:T1)
          }
          frame "Express Glass Vent Close Sunshade Close" {
            n1159 = Bundle By Name(cluster=w3507, "Motion Status.Motion"=All_Motions."Express Glass Vent Close Sunshade Close" ("Current Motion"), "Sequence State.Step Data String"=w3504, "misc status.Serial Port Configured?"=TRUE ("Glass Motor?")) -> (w3506:T1)
          }
          frame "Express Glass Vent Close Sunshade Open" {
            n1160 = Bundle By Name(cluster=w3514, "Motion Status.Motion"=All_Motions."Express Glass Vent Close Sunshade Open" ("Current Motion"), "Sequence State.Step Data String"=w3511, "misc status.Serial Port Configured?"=TRUE ("Glass Motor?")) -> (w3513:T1)
          }
          frame "Express Glass Vent Open" {
            n1161 = Bundle By Name(cluster=w3520, "Motion Status.Motion"=All_Motions."Express Glass Vent Open" ("Current Motion"), "Sequence State.Step Data String"=w3521, "misc status.Serial Port Configured?"=TRUE ("Glass Motor?")) -> (w3519:T1)
          }
          frame "Express Sunshade Close" {
            n1162 = Bundle By Name(cluster=w3527, "Motion Status.Motion"=All_Motions."Express Sunshade Close" ("Current Motion"), "Sequence State.Step Data String"=w3528, "misc status.Serial Port Configured?"=FALSE ("Glass Motor?")) -> (w3526:T1)
          }
          frame "Express Sunshade Close 2" {
            n1163 = Bundle By Name(cluster=w3534, "Motion Status.Motion"=All_Motions."Express Sunshade Close 2" ("Current Motion"), "Sequence State.Step Data String"=w3535, "misc status.Serial Port Configured?"=FALSE ("Glass Motor?")) -> (w3533:T1)
          }
          frame "Express Sunshade Open" {
            n1164 = Bundle By Name(cluster=w3541, "Motion Status.Motion"=All_Motions."Express Sunshade Open" ("Current Motion"), "Sequence State.Step Data String"=w3542, "misc status.Serial Port Configured?"=FALSE ("Glass Motor?")) -> (w3540:T1)
          }
          frame "Express Sunshade Open 2" {
            n1165 = Bundle By Name(cluster=w3548, "Motion Status.Motion"=All_Motions."Express Sunshade Open 2" ("Current Motion"), "Sequence State.Step Data String"=w3549, "misc status.Serial Port Configured?"=FALSE ("Glass Motor?")) -> (w3547:T1)
          }
          frame "Express Vent Open Sunshade Close" {
            n1166 = Bundle By Name(cluster=w3556, "Motion Status.Motion"=All_Motions."Express Glass Vent Open Sunshade Close" ("Current Motion"), "Sequence State.Step Data String"=w3553, "misc status.Serial Port Configured?"=TRUE ("Glass Motor?")) -> (w3555:T1)
          }
          frame "Express Vent Open Sunshade Open" {
            n1167 = Bundle By Name(cluster=w3563, "Motion Status.Motion"=All_Motions."Express Glass Vent Open Sunshade Open" ("Current Motion"), "Sequence State.Step Data String"=w3560, "misc status.Serial Port Configured?"=TRUE ("Glass Motor?")) -> (w3562:T1)
          }
          frame "Glass Goto Position", "Sunshade Goto Position" {
            (unwired) TRUE ("goto motion?")
            # "for BMW, still use glass/ss open/close motions because\nin the 'set switch output' code we need the proper relays set,\nwhereas we dont care with smart motors becuase no switches\nwill be set anyway."
            n1168 = case shown="\"Glass Goto Position\"" w3569 {
              tunnel: [All_Motions."Goto Position Sunshade" ("Current Motion") All_Motions."Goto Position Glass" ("Current Motion")] -> w3565
              tunnel: [FALSE TRUE] -> w3572
              frame "Sunshade Goto Position", Default {
              }
              frame "Glass Goto Position" {
              }
            }
            n1169 = Bundle By Name(cluster=w3571, "Motion Status.Motion"=w3565, "Sequence State.Step Data String"=w3568, "misc status.Serial Port Configured?"=w3572) -> (w3570:T1)
          }
          frame "Glass Slide Close" {
            n1170 = Bundle By Name(cluster=w3581, "Motion Status.Motion"=All_Motions."Glass Slide Close" ("Current Motion"), "Sequence State.Step Data String"=w3582, "misc status.Serial Port Configured?"=TRUE ("Glass Motor?")) -> (w3580:T1)
          }
          frame "Glass Slide Close Sunshade Close" {
            n1171 = Bundle By Name(cluster=w3589, "Motion Status.Motion"=All_Motions."Glass Slide Close Sunshade Close" ("Current Motion"), "Sequence State.Step Data String"=w3586, "misc status.Serial Port Configured?"=TRUE ("Glass Motor?")) -> (w3588:T1)
          }
          frame "Glass Slide Close Sunshade Open" {
            n1172 = Bundle By Name(cluster=w3596, "Motion Status.Motion"=All_Motions."Glass Slide Close Sunshade Open" ("Current Motion"), "Sequence State.Step Data String"=w3593, "misc status.Serial Port Configured?"=TRUE ("Glass Motor?")) -> (w3595:T1)
          }
          frame "Glass Slide Open" {
            n1173 = Bundle By Name(cluster=w3602, "Motion Status.Motion"=All_Motions."Glass Slide Open" ("Current Motion"), "Sequence State.Step Data String"=w3603, "misc status.Serial Port Configured?"=TRUE ("Glass Motor?")) -> (w3601:T1)
          }
          frame "Glass Slide Open Sunshade Close" {
            n1174 = Bundle By Name(cluster=w3610, "Motion Status.Motion"=All_Motions."Glass Slide Open Sunshade Close" ("Current Motion"), "Sequence State.Step Data String"=w3607, "misc status.Serial Port Configured?"=TRUE ("Glass Motor?")) -> (w3609:T1)
          }
          frame "Glass Slide Open Sunshade Open" {
            n1175 = Bundle By Name(cluster=w3617, "Motion Status.Motion"=All_Motions."Glass Slide Open Sunshade Open" ("Current Motion"), "Sequence State.Step Data String"=w3614, "misc status.Serial Port Configured?"=TRUE ("Glass Motor?")) -> (w3616:T1)
          }
          frame "Glass Teach", "Sunshade Teach" {
            (unwired) FALSE ("new element/subarray")
            n1176 = Multiply(x=w3626, y=2) -> (x*y=w3623:i32)
            n1177 = Scan From String(format string="%0.2f", input string=w3629) -> (output 1=w3628:dbl)  [unwired: 3 in, 3 out]
            n1178 = case shown="\"Sunshade Teach\"" w3624 {
              tunnel: [w3635 w3638] -> _
              tunnel: w3623 -> [w3635 w3639]
              tunnel: [All_Motions."Glass Teach" ("Current Motion") All_Motions."Sunshade Teach" ("Current Motion")] -> w3622
              tunnel: [TRUE ("Glass Motor?") FALSE ("Glass Motor?")] -> w3621
              frame "Glass Teach", Default {
              }
              frame "Sunshade Teach" {
                n1179 = Increment(x=w3639) -> (x+1=w3638:i32)
              }
            }
            n1180 = Bundle By Name(cluster=w3625, "Motion Status.Motion"=w3622, "misc status.PS Voltage"=w3628, "Sequence State.Step Data String"="", "misc status.Serial Port Configured?"=w3621) -> (w3632:T1)
          }
          frame "Glass Vent Close" {
            n1181 = Bundle By Name(cluster=w3644, "Motion Status.Motion"=All_Motions."Glass Vent Close" ("Current Motion"), "Sequence State.Step Data String"=w3645, "misc status.Serial Port Configured?"=TRUE ("Glass Motor?")) -> (w3643:T1)
          }
          frame "Glass Vent Close Sunshade Close" {
            n1182 = Bundle By Name(cluster=w3652, "Motion Status.Motion"=All_Motions."Glass Vent Close Sunshade Close" ("Current Motion"), "Sequence State.Step Data String"=w3649, "misc status.Serial Port Configured?"=TRUE ("Glass Motor?")) -> (w3651:T1)
          }
          frame "Glass Vent Close Sunshade Open" {
            n1183 = Bundle By Name(cluster=w3659, "Motion Status.Motion"=All_Motions."Glass Vent Close Sunshade Open" ("Current Motion"), "Sequence State.Step Data String"=w3656, "misc status.Serial Port Configured?"=TRUE ("Glass Motor?")) -> (w3658:T1)
          }
          frame "Glass Vent Open" {
            n1184 = Bundle By Name(cluster=w3665, "Motion Status.Motion"=All_Motions."Glass Vent Open" ("Current Motion"), "Sequence State.Step Data String"=w3666, "misc status.Serial Port Configured?"=TRUE ("Glass Motor?")) -> (w3664:T1)
          }
          frame "Glass Vent Open Sunshade Close" {
            n1185 = Bundle By Name(cluster=w3673, "Motion Status.Motion"=All_Motions."Glass Vent Open Sunshade Close" ("Current Motion"), "Sequence State.Step Data String"=w3670, "misc status.Serial Port Configured?"=TRUE ("Glass Motor?")) -> (w3672:T1)
          }
          frame "Glass Vent Open Sunshade Open" {
            n1186 = Bundle By Name(cluster=w3680, "Motion Status.Motion"=All_Motions."Glass Vent Open Sunshade Open" ("Current Motion"), "Sequence State.Step Data String"=w3677, "misc status.Serial Port Configured?"=TRUE ("Glass Motor?")) -> (w3679:T1)
          }
          frame "Go To Position" {
            # "this is only here for reverse compatibility - the user should\nuse the full blown 'glass goto postion' and 'sunshade goto position'\nsteps becuase those have many more options."
            n1187 = Unflatten From String(type=T50 {"AP Data Type"=enum."91/61", "Glass Motor?"=FALSE, "Collect AP Data?"=FALSE, "Go To Position"=10, "Rear Rollo?"=FALSE} ("Goto Position Control"), binary string=w3696, error in (no error)=w3695) -> (value=w3693:T50, error out=w3690:errorcluster)  [unwired: 2 in, 1 out]
            n1188 = Unbundle By Name(w3693) -> ("AP Data Type"=w3686:T13, "Glass Motor?"=w3692:bool, "Collect AP Data?"=w3685:bool, "Go To Position"=w3684:u16)
            n1189 = Select(t=All_Motions."Goto Position Glass" ("Current Motion"), s=w3692, f=All_Motions."Goto Position Sunshade" ("Current Motion")) -> (s? t:f=w3697:T3)
            n1190 = Bundle By Name(cluster=T12 {"Power Supply Voltage"=13.0, "Min Avg Current"=0.0, "Max Avg Current"=0.0, "Min Run Time"=0.0, "Max Run Time"=0.0, "Min Speed"=0.0, "Max Speed"=0.0, "AP Data % of Threshold"=0.0, "Travel Distance"=0.0, "AP Data Type"=enum."91/61", "Check Current"=FALSE, "Check Run Time"=FALSE, "Check Speed"=FALSE, "Express Motion?"=FALSE, "Check Sound Test"=FALSE, "Check Position?"=FALSE, "Collect AP Data"=FALSE, "Inital Position"=0, "End Position"=0, "Goto Posiition"=0, "Max max Current"=0.0, "Min max Current"=0.0, "Check max Current"=FALSE, "Check Sound"=FALSE, "Min Sound (dB)"=0.0, "Max Sound (dB)"=0.0, "SW Mode"=enum."Hard Switch", "LIN Msg"={"ID"=0, "Msg"=[], "LDF"="EX1H"}} ("Motion Data Cluster"), "AP Data Type"=w3686, "Collect AP Data"=w3685, "Goto Posiition"=w3684, "Power Supply Voltage"=w3683) -> (w3688:T12)
            n1191 = Flatten To String(anything=w3688, error in (no error)=w3690) -> (data string=w3687:string, error out=w3689:errorcluster)  [unwired: 2 in, 1 out]
            n1192 = Bundle By Name(cluster=w3701, "Motion Status.Motion"=w3697, "Sequence State.Step Data String"=w3687, "misc status.Serial Port Configured?"=w3692) -> (w3700:T1)
          }
          frame "Set Power Supply" {
            n1193 = Scan From String(format string="%0.2f", input string=w3705, error in=w3703) -> (error out=w3702:errorcluster, output 1=w3704:dbl)  [unwired: 2 in, 2 out]
            n1194 = Bundle By Name(cluster=w3708, "misc status.PS Voltage"=w3704) -> (w3709:T1)
          }
          frame "Sunshade Close" {
            n1195 = Bundle By Name(cluster=w3714, "Motion Status.Motion"=All_Motions."Sunshade Close" ("Current Motion"), "Sequence State.Step Data String"=w3715, "misc status.Serial Port Configured?"=FALSE ("Glass Motor?")) -> (w3713:T1)
          }
          frame "Sunshade Close 2" {
            n1196 = Bundle By Name(cluster=w3721, "Motion Status.Motion"=All_Motions."Sunshade Close 2" ("Current Motion"), "Sequence State.Step Data String"=w3722, "misc status.Serial Port Configured?"=FALSE ("Glass Motor?")) -> (w3720:T1)
          }
          frame "Sunshade Open" {
            n1197 = Bundle By Name(cluster=w3728, "Motion Status.Motion"=All_Motions."Sunshade Open" ("Current Motion"), "Sequence State.Step Data String"=w3729, "misc status.Serial Port Configured?"=FALSE ("Glass Motor?")) -> (w3727:T1)
          }
          frame "Sunshade Open 2" {
            n1198 = Bundle By Name(cluster=w3735, "Motion Status.Motion"=All_Motions."Sunshade Open 2" ("Current Motion"), "Sequence State.Step Data String"=w3736, "misc status.Serial Port Configured?"=FALSE ("Glass Motor?")) -> (w3734:T1)
          }
          frame "check NVH Operator result" {
            n1199 = Unbundle By Name(w3741) -> ("NVH Operator Check"=w3740:T40)
            n1200 = call "plc write bool.vi"("value"=TRUE, "addr,tag"=w3740) -> ()  [unwired: 9 in, 1 out]
            n1201 = Bundle By Name(cluster=w3742, "Sequence State.Step Data String"=w3744, "Sequence State.Step Description"=w3743, "Second Check?"=TRUE) -> (w3745:T1)
          }
          frame Default {
            n1202 = Bundle By Name(cluster=w3753, "Sequence State.Step Data String"=w3752, "Sequence State.Step Description"=w3749) -> (w3754:T1)
            n1203 = Build Array("wait for operator action") -> (w3751:string[])
          }
        }
      }
      frame Default {
        n1204 = Unbundle By Name(w3772) -> ("Store Data.Error Table"=w3768:string[][], "Sequence State"=w3760:T24, "Sequence State.Active Step"=w3757:u8, "Sequence State.Seqence"=w3758:T25[])
        n1205 = Index Array(array=w3758, index=w3757) -> (element=w3756:T25)
        n1206 = Number To Decimal String(number=w3757) -> (decimal integer string=w3761:string)  [unwired: 1 in]
        n1207 = Unbundle By Name(w3756) -> ("Name"=w3755:string)
        n1208 = Concatenate Strings(" Non-Existing State Called. Intended State was - " ("string"), w3775, ", current sequence step #" ("string"), w3761, ", " ("string"), w3755) -> (w3766:string)
        n1209 = call "pass fail action decision.vi"("Pass?"=FALSE, "Sequence State in"=w3760, "event queue in"=w3769) -> ("Sequence State out"=w3770:T24, "Event queue out"=w3774:string[])  [unwired: 7 in]
        n1210 = call "EOL Error Table.vi"("Error Description"=w3766, "error in"=w3764, "Error No."=u16 28, "Error Table In"=w3768) -> ("error out"=w3763:errorcluster, "Error Table Out"=w3767:string[][])  [unwired: 6 in]
        n1211 = Bundle By Name(cluster=w3772, "Store Data.Error Table"=w3767, "Sequence State"=w3770) -> (w3771:T1)
      }
    }
  }
  "error out" <- w13
  n1212 = Unbundle By Name("Main State Cluster") -> ("Application Status"=w3:string, "rs232 port map.PS Port"=w8:refnum<visa-resource-name>, "Station Index"=w7:i32, "misc station config.power supply type"=w9:T20, "ctl refs.exit program"=w6:refnum<vi>)
  n1213 = Empty String/Path?(string/path=w3) -> (empty?=w2:bool)
  n1214 = case shown="假" w2 {
    tunnel: w9 -> [w3780 _]
    tunnel: w8 -> [w3779 _]
    tunnel: w7 -> [w3778 _]
    tunnel: w6 -> [w3777 _]
    frame False {
      n1215 = case shown="\"ITECH\"" w3780 {
        tunnel: w3779 -> [w3782 w3785 _]
        tunnel: w3778 -> [_ w3784 _]
        tunnel: w3777 -> [w3781 w3783 _]
        frame "ITECH" {
          n1216 = call "EOL_ITECHData.vi"("Exit Program"=w3781, "VISA name"=w3782) -> ()  [unwired: 10 in]
        }
        frame "ZUPser" {
          n1217 = call "EOL_TDKData.vi"("Exit Program"=w3783, "idx"=w3784, "VISA name"=w3785) -> ()  [unwired: 9 in]
        }
        frame Default {
        }
      }
    }
    frame True {
    }
  }
  n1218 = Request Deallocation(w1) -> ()
